vi "Hardware-DI-B-Host.vi"() -> ()   [LabVIEW 2016]
uses:
  <vilib>/Powertrain Controls/Device Drivers/DCM/Rev0/UI/Bank B.ctl
  Shared/Typedefs/DI-Phase-Array-2D.ctl
  <vilib>/Powertrain Controls/Device Drivers/DCM/DI/RT/Phase.ctl
  <vilib>/Powertrain Controls/Device Drivers/DCM/Rev0/FPGA/DI - Drive State.ctl
  <vilib>/Powertrain Controls/Device Drivers/DCM/DI/FPGA/Phase Step.ctl
  <vilib>/Powertrain Controls/Device Drivers/DCM/DI/FPGA/Control.ctl
  <vilib>/Powertrain Controls/Device Drivers/DCM/Rev0/RT/Configuration.ctl
  <vilib>/Powertrain Controls/Device Drivers/DCM/Rev0/FPGA/DI - Bank Configuration.ctl
  Host SubVIs/DI Command Element.ctl
  <vilib>/Powertrain Controls/Device Drivers/DCM/Rev0/FPGA/Digital Channel.ctl
  Shared/Typedefs/DI-Command-Array.ctl
  <vilib>/Powertrain Controls/Device Drivers/DCM/DI/RT/Command.ctl
  <vilib>/Powertrain Controls/Device Drivers/DCM/DI/FPGA/Mode.ctl
  <vilib>/Powertrain Controls/Device Drivers/DCM/DI/RT/Command Sequence.ctl
  <vilib>/Powertrain Controls/Device Drivers/DCM/DI/RT/Angle Control.ctl
  Shared/Typedefs/DI-Phase-Array-1D.ctl
  <vilib>/addons/Software Calibration Management/XControls/SubHost.xctl
  <vilib>/Powertrain Controls/Device Drivers/DCM/Rev0/FPGA/DI - Faults.ctl
  Host SubVIs/Pump Command Element.ctl
  <vilib>/Powertrain Controls/Device Drivers/DCM/Rev0/FPGA/DI - ADC Signals.ctl
  <vilib>/Powertrain Controls/Device Drivers/DCM/DI/FPGA/Capture Event.ctl
  <vilib>/Powertrain Controls/Device Drivers/DCM/Rev0/RT/System State.ctl
  <vilib>/Powertrain Controls/Device Drivers/DCM/Rev0/RT/System ADC.ctl
  <vilib>/Powertrain Controls/Device Drivers/DCM/Rev0/RT/Internal Fault.ctl
  <vilib>/Powertrain Controls/Device Drivers/DCM/Rev0/RT/Run State.ctl
  <vilib>/Powertrain Controls/Device Drivers/DCM/Rev0/UI/Configuration.ctl
  <vilib>/Powertrain Controls/Device Drivers/DCM/Rev0/UI/System Configuration.ctl
  <vilib>/Powertrain Controls/Device Drivers/DCM/Rev0/UI/Injector Configuration.ctl
  <vilib>/Powertrain Controls/Device Drivers/DCM/Rev0/UI/Test Comparators.vi
  <vilib>/Powertrain Controls/Device Drivers/DCM/Rev0/UI/DAC Delay.vi
  <vilib>/Powertrain Controls/Device Drivers/DCM/DI/RT/Phase Convert.vi
  <vilib>/Powertrain Controls/Device Drivers/DCM/DI/RT/Skew.vi
  <vilib>/Powertrain Controls/Device Drivers/DCM/Rev0/UI/Calibrations.vi
  <vilib>/Powertrain Controls/Device Drivers/DCM/Rev0/UI/One Injection Command.vi
  <vilib>/Powertrain Controls/Device Drivers/DCM/DI/FPGA/Simulate Phase Array.vi
  <vilib>/Powertrain Controls/Device Drivers/DCM/Rev0/FPGA/DI - Setpoints.vi
  <vilib>/Powertrain Controls/Device Drivers/DCM/Rev0/UI/Phase State Control.vi
  <vilib>/Powertrain Controls/Device Drivers/DCM/Rev0/UI/Circuit Model Step.vi
  <vilib>/Powertrain Controls/Device Drivers/DCM/Rev0/UI/FET Movie Data.vi
  <vilib>/Powertrain Controls/Device Drivers/DCM/DI/FPGA/DCM - FPGA - DI.lvlib
  <vilib>/Powertrain Controls/Device Drivers/DCM/Rev0/UI/DCM - UI.lvlib
  <vilib>/Powertrain Controls/Device Drivers/DCM/Rev0/FPGA/DCM - FPGA.lvlib
  <vilib>/Powertrain Controls/Device Drivers/DCM/DI/RT/DCM - RT - DI.lvlib
  <vilib>/Powertrain Controls/Device Drivers/DCM/Rev0/RT/DCM - RT.lvclass
  Shared/DSI-Shared.lvlib
panel:
  out "RunState":T1
  out "_BoostSlider":cluster{dbl, dbl, dbl, dbl}(slide)={0.0, 166.94117647058823, 117.76470588235294, 190.23529411764707} scale=0.0..220.0
  out "_Bank B Status":T2 caption="Injector and Pump Simulation Settings" {"Boost Clamp [V]" format="%#_3p"; "Ext HV [V]" format="%#_3p"; "DRVP [V]" format="%#_3p"; "Pump Zener [V]" format="%#_3p"; "DI Zener [V]" format="%#_3p"; "Secondary 3-4 [V]" format="%#_3p"; "Secondary 1-2 [V]" format="%#_3p"; "Primary 3-4 [V]" format="%#_3p"; "Primary 1-2 [V]" format="%#_3p"}
  in  "_DI Bank_Configuration":T3 caption="DI Bank A_Configuration" {"Pump Zener Voltage [V]" min=0 max=240 format="%#_13g"; "DI Zener Voltage [V]" min=0 max=100 format="%#_13g"; "Boost Clamp [V]" min=0 max=220 format="%#_13g"; "Boost Voltage [V]" min=0 max=220 format="%#_13g"}
  in  "DI Scope":T5(xcontrol)
  in  "UserOS":bool
  in  "UserOSTime":sgl caption="[s]" format="%#.3p"
  in  "_Hidden Items":enum32{"DI-A Configurations Items"}(tab)
  out "dt":sgl=13.7
  out "_Bank A?":bool
  in  "_Redraw Slider":bool
  out "SYS|Exec|CalLoading":bool
  in  "_Refresh All":bool
  in  "_Redraw Pump Command":bool
  in  "_Redraw DI Command":bool
  in  "InjCmd":T6=[{"Mode"=enum."Off", "Digital Input"=enum."Unused", "Default Profile Index"=0, "Cal Freq [Hz]"=0.0, "Cal Duration [s]"=0.0, "Cal Increment [s]"=0.0, "Cal Pulses"=0, "TMP Command Sequence"=[{"Duration [s]"=0.0, "Level"=FALSE, "Run/Stop"=FALSE, "Profile Index"=0}, {"Duration [s]"=0.0, "Level"=FALSE, "Run/Stop"=FALSE, "Profile Index"=0}, {"Duration [s]"=0.0, "Level"=FALSE, "Run/Stop"=FALSE, "Profile Index"=0}, {"Duration [s]"=0.0, "Level"=FALSE, "Run/Stop"=FALSE, "Profile Index"=0}, {"Duration [s]"=0.0, "Level"=FALSE, "Run/Stop"=FALSE, "Profile Index"=0}, {"Duration [s]"=0.0, "Level"=FALSE, "Run/Stop"=FALSE, "Profile Index"=0}, {"Duration [s]"=0.0, "Level"=FALSE, "Run/Stop"=FALSE, "Profile Index"=0}, {"Duration [s]"=0.0, "Level"=FALSE, "Run/Stop"=FALSE, "Profile Index"=0}], "EPT TDC Offset [CAD]"=0.0, "EPT Window Start [DBTDC]"=0.0, "EPT Window End [DBTDC]"=0.0, "EPT Angles"=[{"Enable"=FALSE, "Timing [DBTDC]"=0.0, "Duration [s]"=0.0, "Profile Index"=0}, {"Enable"=FALSE, "Timing [DBTDC]"=0.0, "Duration [s]"=0.0, "Profile Index"=0}, {"Enable"=FALSE, "Timing [DBTDC]"=0.0, "Duration [s]"=0.0, "Profile Index"=0}, {"Enable"=FALSE, "Timing [DBTDC]"=0.0, "Duration [s]"=0.0, "Profile Index"=0}], "EPT Skip Fire"=FALSE, "EPT Skip Index"=0, "EPT Precharge Duration [s]"=0.0, "EPT Precharge Profile Index"=0}, {"Mode"=enum."Off", "Digital Input"=enum."Unused", "Default Profile Index"=0, "Cal Freq [Hz]"=0.0, "Cal Duration [s]"=0.0, "Cal Increment [s]"=0.0, "Cal Pulses"=0, "TMP Command Sequence"=[{"Duration [s]"=0.0, "Level"=FALSE, "Run/Stop"=FALSE, "Profile Index"=0}, {"Duration [s]"=0.0, "Level"=FALSE, "Run/Stop"=FALSE, "Profile Index"=0}, {"Duration [s]"=0.0, "Level"=FALSE, "Run/Stop"=FALSE, "Profile Index"=0}, {"Duration [s]"=0.0, "Level"=FALSE, "Run/Stop"=FALSE, "Profile Index"=0}, {"Duration [s]"=0.0, "Level"=FALSE, "Run/Stop"=FALSE, "Profile Index"=0}, {"Duration [s]"=0.0, "Level"=FALSE, "Run/Stop"=FALSE, "Profile Index"=0}, {"Duration [s]"=0.0, "Level"=FALSE, "Run/Stop"=FALSE, "Profile Index"=0}, {"Duration [s]"=0.0, "Level"=FALSE, "Run/Stop"=FALSE, "Profile Index"=0}], "EPT TDC Offset [CAD]"=0.0, "EPT Window Start [DBTDC]"=0.0, "EPT Window End [DBTDC]"=0.0, "EPT Angles"=[{"Enable"=FALSE, "Timing [DBTDC]"=0.0, "Duration [s]"=0.0, "Profile Index"=0}, {"Enable"=FALSE, "Timing [DBTDC]"=0.0, "Duration [s]"=0.0, "Profile Index"=0}, {"Enable"=FALSE, "Timing [DBTDC]"=0.0, "Duration [s]"=0.0, "Profile Index"=0}, {"Enable"=FALSE, "Timing [DBTDC]"=0.0, "Duration [s]"=0.0, "Profile Index"=0}], "EPT Skip Fire"=FALSE, "EPT Skip Index"=0, "EPT Precharge Duration [s]"=0.0, "EPT Precharge Profile Index"=0}, {"Mode"=enum."Off", "Digital Input"=enum."Unused", "Default Profile Index"=0, "Cal Freq [Hz]"=0.0, "Cal Duration [s]"=0.0, "Cal Increment [s]"=0.0, "Cal Pulses"=0, "TMP Command Sequence"=[{"Duration [s]"=0.0, "Level"=FALSE, "Run/Stop"=FALSE, "Profile Index"=0}, {"Duration [s]"=0.0, "Level"=FALSE, "Run/Stop"=FALSE, "Profile Index"=0}, {"Duration [s]"=0.0, "Level"=FALSE, "Run/Stop"=FALSE, "Profile Index"=0}, {"Duration [s]"=0.0, "Level"=FALSE, "Run/Stop"=FALSE, "Profile Index"=0}, {"Duration [s]"=0.0, "Level"=FALSE, "Run/Stop"=FALSE, "Profile Index"=0}, {"Duration [s]"=0.0, "Level"=FALSE, "Run/Stop"=FALSE, "Profile Index"=0}, {"Duration [s]"=0.0, "Level"=FALSE, "Run/Stop"=FALSE, "Profile Index"=0}, {"Duration [s]"=0.0, "Level"=FALSE, "Run/Stop"=FALSE, "Profile Index"=0}], "EPT TDC Offset [CAD]"=0.0, "EPT Window Start [DBTDC]"=0.0, "EPT Window End [DBTDC]"=0.0, "EPT Angles"=[{"Enable"=FALSE, "Timing [DBTDC]"=0.0, "Duration [s]"=0.0, "Profile Index"=0}, {"Enable"=FALSE, "Timing [DBTDC]"=0.0, "Duration [s]"=0.0, "Profile Index"=0}, {"Enable"=FALSE, "Timing [DBTDC]"=0.0, "Duration [s]"=0.0, "Profile Index"=0}, {"Enable"=FALSE, "Timing [DBTDC]"=0.0, "Duration [s]"=0.0, "Profile Index"=0}], "EPT Skip Fire"=FALSE, "EPT Skip Index"=0, "EPT Precharge Duration [s]"=0.0, "EPT Precharge Profile Index"=0}, {"Mode"=enum."Off", "Digital Input"=enum."Unused", "Default Profile Index"=0, "Cal Freq [Hz]"=0.0, "Cal Duration [s]"=0.0, "Cal Increment [s]"=0.0, "Cal Pulses"=0, "TMP Command Sequence"=[{"Duration [s]"=0.0, "Level"=FALSE, "Run/Stop"=FALSE, "Profile Index"=0}, {"Duration [s]"=0.0, "Level"=FALSE, "Run/Stop"=FALSE, "Profile Index"=0}, {"Duration [s]"=0.0, "Level"=FALSE, "Run/Stop"=FALSE, "Profile Index"=0}, {"Duration [s]"=0.0, "Level"=FALSE, "Run/Stop"=FALSE, "Profile Index"=0}, {"Duration [s]"=0.0, "Level"=FALSE, "Run/Stop"=FALSE, "Profile Index"=0}, {"Duration [s]"=0.0, "Level"=FALSE, "Run/Stop"=FALSE, "Profile Index"=0}, {"Duration [s]"=0.0, "Level"=FALSE, "Run/Stop"=FALSE, "Profile Index"=0}, {"Duration [s]"=0.0, "Level"=FALSE, "Run/Stop"=FALSE, "Profile Index"=0}], "EPT TDC Offset [CAD]"=0.0, "EPT Window Start [DBTDC]"=0.0, "EPT Window End [DBTDC]"=0.0, "EPT Angles"=[{"Enable"=FALSE, "Timing [DBTDC]"=0.0, "Duration [s]"=0.0, "Profile Index"=0}, {"Enable"=FALSE, "Timing [DBTDC]"=0.0, "Duration [s]"=0.0, "Profile Index"=0}, {"Enable"=FALSE, "Timing [DBTDC]"=0.0, "Duration [s]"=0.0, "Profile Index"=0}, {"Enable"=FALSE, "Timing [DBTDC]"=0.0, "Duration [s]"=0.0, "Profile Index"=0}], "EPT Skip Fire"=FALSE, "EPT Skip Index"=0, "EPT Precharge Duration [s]"=0.0, "EPT Precharge Profile Index"=0}, {"Mode"=enum."Off", "Digital Input"=enum."Unused", "Default Profile Index"=0, "Cal Freq [Hz]"=0.0, "Cal Duration [s]"=0.0, "Cal Increment [s]"=0.0, "Cal Pulses"=0, "TMP Command Sequence"=[{"Duration [s]"=0.0, "Level"=FALSE, "Run/Stop"=FALSE, "Profile Index"=0}, {"Duration [s]"=0.0, "Level"=FALSE, "Run/Stop"=FALSE, "Profile Index"=0}, {"Duration [s]"=0.0, "Level"=FALSE, "Run/Stop"=FALSE, "Profile Index"=0}, {"Duration [s]"=0.0, "Level"=FALSE, "Run/Stop"=FALSE, "Profile Index"=0}, {"Duration [s]"=0.0, "Level"=FALSE, "Run/Stop"=FALSE, "Profile Index"=0}, {"Duration [s]"=0.0, "Level"=FALSE, "Run/Stop"=FALSE, "Profile Index"=0}, {"Duration [s]"=0.0, "Level"=FALSE, "Run/Stop"=FALSE, "Profile Index"=0}, {"Duration [s]"=0.0, "Level"=FALSE, "Run/Stop"=FALSE, "Profile Index"=0}], "EPT TDC Offset [CAD]"=0.0, "EPT Window Start [DBTDC]"=0.0, "EPT Window End [DBTDC]"=0.0, "EPT Angles"=[{"Enable"=FALSE, "Timing [DBTDC]"=0.0, "Duration [s]"=0.0, "Profile Index"=0}, {"Enable"=FALSE, "Timing [DBTDC]"=0.0, "Duration [s]"=0.0, "Profile Index"=0}, {"Enable"=FALSE, "Timing [DBTDC]"=0.0, "Duration [s]"=0.0, "Profile Index"=0}, {"Enable"=FALSE, "Timing [DBTDC]"=0.0, "Duration [s]"=0.0, "Profile Index"=0}], "EPT Skip Fire"=FALSE, "EPT Skip Index"=0, "EPT Precharge Duration [s]"=0.0, "EPT Precharge Profile Index"=0}, {"Mode"=enum."Off", "Digital Input"=enum."Unused", "Default Profile Index"=0, "Cal Freq [Hz]"=0.0, "Cal Duration [s]"=0.0, "Cal Increment [s]"=0.0, "Cal Pulses"=0, "TMP Command Sequence"=[{"Duration [s]"=0.0, "Level"=FALSE, "Run/Stop"=FALSE, "Profile Index"=0}, {"Duration [s]"=0.0, "Level"=FALSE, "Run/Stop"=FALSE, "Profile Index"=0}, {"Duration [s]"=0.0, "Level"=FALSE, "Run/Stop"=FALSE, "Profile Index"=0}, {"Duration [s]"=0.0, "Level"=FALSE, "Run/Stop"=FALSE, "Profile Index"=0}, {"Duration [s]"=0.0, "Level"=FALSE, "Run/Stop"=FALSE, "Profile Index"=0}, {"Duration [s]"=0.0, "Level"=FALSE, "Run/Stop"=FALSE, "Profile Index"=0}, {"Duration [s]"=0.0, "Level"=FALSE, "Run/Stop"=FALSE, "Profile Index"=0}, {"Duration [s]"=0.0, "Level"=FALSE, "Run/Stop"=FALSE, "Profile Index"=0}], "EPT TDC Offset [CAD]"=0.0, "EPT Window Start [DBTDC]"=0.0, "EPT Window End [DBTDC]"=0.0, "EPT Angles"=[{"Enable"=FALSE, "Timing [DBTDC]"=0.0, "Duration [s]"=0.0, "Profile Index"=0}, {"Enable"=FALSE, "Timing [DBTDC]"=0.0, "Duration [s]"=0.0, "Profile Index"=0}, {"Enable"=FALSE, "Timing [DBTDC]"=0.0, "Duration [s]"=0.0, "Profile Index"=0}, {"Enable"=FALSE, "Timing [DBTDC]"=0.0, "Duration [s]"=0.0, "Profile Index"=0}], "EPT Skip Fire"=FALSE, "EPT Skip Index"=0, "EPT Precharge Duration [s]"=0.0, "EPT Precharge Profile Index"=0}, {"Mode"=enum."Off", "Digital Input"=enum."Unused", "Default Profile Index"=0, "Cal Freq [Hz]"=0.0, "Cal Duration [s]"=0.0, "Cal Increment [s]"=0.0, "Cal Pulses"=0, "TMP Command Sequence"=[{"Duration [s]"=0.0, "Level"=FALSE, "Run/Stop"=FALSE, "Profile Index"=0}, {"Duration [s]"=0.0, "Level"=FALSE, "Run/Stop"=FALSE, "Profile Index"=0}, {"Duration [s]"=0.0, "Level"=FALSE, "Run/Stop"=FALSE, "Profile Index"=0}, {"Duration [s]"=0.0, "Level"=FALSE, "Run/Stop"=FALSE, "Profile Index"=0}, {"Duration [s]"=0.0, "Level"=FALSE, "Run/Stop"=FALSE, "Profile Index"=0}, {"Duration [s]"=0.0, "Level"=FALSE, "Run/Stop"=FALSE, "Profile Index"=0}, {"Duration [s]"=0.0, "Level"=FALSE, "Run/Stop"=FALSE, "Profile Index"=0}, {"Duration [s]"=0.0, "Level"=FALSE, "Run/Stop"=FALSE, "Profile Index"=0}], "EPT TDC Offset [CAD]"=0.0, "EPT Window Start [DBTDC]"=0.0, "EPT Window End [DBTDC]"=0.0, "EPT Angles"=[{"Enable"=FALSE, "Timing [DBTDC]"=0.0, "Duration [s]"=0.0, "Profile Index"=0}, {"Enable"=FALSE, "Timing [DBTDC]"=0.0, "Duration [s]"=0.0, "Profile Index"=0}, {"Enable"=FALSE, "Timing [DBTDC]"=0.0, "Duration [s]"=0.0, "Profile Index"=0}, {"Enable"=FALSE, "Timing [DBTDC]"=0.0, "Duration [s]"=0.0, "Profile Index"=0}], "EPT Skip Fire"=FALSE, "EPT Skip Index"=0, "EPT Precharge Duration [s]"=0.0, "EPT Precharge Profile Index"=0}, {"Mode"=enum."Off", "Digital Input"=enum."Unused", "Default Profile Index"=0, "Cal Freq [Hz]"=0.0, "Cal Duration [s]"=0.0, "Cal Increment [s]"=0.0, "Cal Pulses"=0, "TMP Command Sequence"=[{"Duration [s]"=0.0, "Level"=FALSE, "Run/Stop"=FALSE, "Profile Index"=0}, {"Duration [s]"=0.0, "Level"=FALSE, "Run/Stop"=FALSE, "Profile Index"=0}, {"Duration [s]"=0.0, "Level"=FALSE, "Run/Stop"=FALSE, "Profile Index"=0}, {"Duration [s]"=0.0, "Level"=FALSE, "Run/Stop"=FALSE, "Profile Index"=0}, {"Duration [s]"=0.0, "Level"=FALSE, "Run/Stop"=FALSE, "Profile Index"=0}, {"Duration [s]"=0.0, "Level"=FALSE, "Run/Stop"=FALSE, "Profile Index"=0}, {"Duration [s]"=0.0, "Level"=FALSE, "Run/Stop"=FALSE, "Profile Index"=0}, {"Duration [s]"=0.0, "Level"=FALSE, "Run/Stop"=FALSE, "Profile Index"=0}], "EPT TDC Offset [CAD]"=0.0, "EPT Window Start [DBTDC]"=0.0, "EPT Window End [DBTDC]"=0.0, "EPT Angles"=[{"Enable"=FALSE, "Timing [DBTDC]"=0.0, "Duration [s]"=0.0, "Profile Index"=0}, {"Enable"=FALSE, "Timing [DBTDC]"=0.0, "Duration [s]"=0.0, "Profile Index"=0}, {"Enable"=FALSE, "Timing [DBTDC]"=0.0, "Duration [s]"=0.0, "Profile Index"=0}, {"Enable"=FALSE, "Timing [DBTDC]"=0.0, "Duration [s]"=0.0, "Profile Index"=0}], "EPT Skip Fire"=FALSE, "EPT Skip Index"=0, "EPT Precharge Duration [s]"=0.0, "EPT Precharge Profile Index"=0}] {"EPT Precharge Profile Index" max=15; "EPT Precharge Duration [s]" min=0 format="%#_4p"; "Default Profile Index" max=15; "Cal Increment [s]" format="%#_3p"; "TMP Command Sequence"."Profile Index" max=7; "TMP Command Sequence"."Duration [s]" min=0 max=100 format="%#_3p"; "Cal Pulses" max=511; "EPT Skip Index" max=7; "EPT Angles"."Profile Index" max=7; "EPT Angles"."Duration [s]" min=0 max=100 format="%#_3p"; "Cal Duration [s]" format="%#_3p"; "Cal Freq [Hz]" format="%#_3p"}
  in  "ChanSelect4":u8(ring) items=["I LS A1/A5", "I LS A2/A6", "I LS A3/A7", "I LS A4", "I LS A8/PumpA", "V PZ A1", "V PZ A2", "V PZ A3", "V PZ A4", "V S A1", "V S A2", "V S A3", "V S A4", "V S A5", "V S A6", "V S A7", "V S A8", "V Pump A", "V Secondary A1A2", "V Secondary A3A4", "V Ext HV A", "------------------------ ", "I LS B1/B5", "I LS B2/B6", "I LS B3/B7", "I LS B4", "I LS B8/PumpB", "V PZ B1", "V PZ B2", "V PZ B3", "V PZ B4", "V S B1", "V S B2", "V S B3", "V S B4", "V S B5", "V S B6", "V S B7", "V S B8", "V Pump B", "V Secondary B1B2", "V Secondary B3B4", "V Ext HV B", "-------------------------  ", "AI 1", "AI 2", "AI 3", "AI 4", "AI 5", "AI 6", "AI 7", "AI 8", "AI 9", "AI 10", "AI 11", "AI 12", "-------------------------   ", "V DRVP"]
  in  "ChanSelect3":u8(ring) items=["I LS A1/A5", "I LS A2/A6", "I LS A3/A7", "I LS A4", "I LS A8/PumpA", "V PZ A1", "V PZ A2", "V PZ A3", "V PZ A4", "V S A1", "V S A2", "V S A3", "V S A4", "V S A5", "V S A6", "V S A7", "V S A8", "V Pump A", "V Secondary A1A2", "V Secondary A3A4", "V Ext HV A", "------------------------ ", "I LS B1/B5", "I LS B2/B6", "I LS B3/B7", "I LS B4", "I LS B8/PumpB", "V PZ B1", "V PZ B2", "V PZ B3", "V PZ B4", "V S B1", "V S B2", "V S B3", "V S B4", "V S B5", "V S B6", "V S B7", "V S B8", "V Pump B", "V Secondary B1B2", "V Secondary B3B4", "V Ext HV B", "-------------------------  ", "AI 1", "AI 2", "AI 3", "AI 4", "AI 5", "AI 6", "AI 7", "AI 8", "AI 9", "AI 10", "AI 11", "AI 12", "-------------------------   ", "V DRVP"]
  in  "_Redraw Profiles Usage Tracker":bool
  in  "_Redraw Pump Timing Plot":bool
  in  "InjectEnable":bool
  in  "PSEnable":bool
  in  "Configuration":u8
  in  "BoostV":sgl format="%#_13g"
  in  "ZenerV":sgl format="%#_13g"
  in  "ZenerEnable":bool
  in  "PumpZenerV":sgl format="%#_13g"
  in  "BoostClampV":sgl format="%#_13g"
  in  "_Redraw Phase":bool
  in  "_Redraw Phase Plot":bool
  in  "_Redraw Phase Lists":bool
  in  "_Redraw Pump Phase Plot":bool
  in  "_Redraw Pump Phase List":bool
  in  "FaultClear":u8
  in  "ChanSelect2":u8(ring) items=["I LS A1/A5", "I LS A2/A6", "I LS A3/A7", "I LS A4", "I LS A8/PumpA", "V PZ A1", "V PZ A2", "V PZ A3", "V PZ A4", "V S A1", "V S A2", "V S A3", "V S A4", "V S A5", "V S A6", "V S A7", "V S A8", "V Pump A", "V Secondary A1A2", "V Secondary A3A4", "V Ext HV A", "------------------------ ", "I LS B1/B5", "I LS B2/B6", "I LS B3/B7", "I LS B4", "I LS B8/PumpB", "V PZ B1", "V PZ B2", "V PZ B3", "V PZ B4", "V S B1", "V S B2", "V S B3", "V S B4", "V S B5", "V S B6", "V S B7", "V S B8", "V Pump B", "V Secondary B1B2", "V Secondary B3B4", "V Ext HV B", "-------------------------  ", "AI 1", "AI 2", "AI 3", "AI 4", "AI 5", "AI 6", "AI 7", "AI 8", "AI 9", "AI 10", "AI 11", "AI 12", "-------------------------   ", "V DRVP"]
  in  "ChanSelect1":u8(ring) items=["I LS A1/A5", "I LS A2/A6", "I LS A3/A7", "I LS A4", "I LS A8/PumpA", "V PZ A1", "V PZ A2", "V PZ A3", "V PZ A4", "V S A1", "V S A2", "V S A3", "V S A4", "V S A5", "V S A6", "V S A7", "V S A8", "V Pump A", "V Secondary A1A2", "V Secondary A3A4", "V Ext HV A", "------------------------ ", "I LS B1/B5", "I LS B2/B6", "I LS B3/B7", "I LS B4", "I LS B8/PumpB", "V PZ B1", "V PZ B2", "V PZ B3", "V PZ B4", "V S B1", "V S B2", "V S B3", "V S B4", "V S B5", "V S B6", "V S B7", "V S B8", "V Pump B", "V Secondary B1B2", "V Secondary B3B4", "V Ext HV B", "-------------------------  ", "AI 1", "AI 2", "AI 3", "AI 4", "AI 5", "AI 6", "AI 7", "AI 8", "AI 9", "AI 10", "AI 11", "AI 12", "-------------------------   ", "V DRVP"]
  in  "ScopeEnable":bool
  in  "ScopeEvent":u8(ring) items=["Unused", "Injector A1", "Injector A2", "Injector A3", "Injector A4", "Injector A5", "Injector A6", "Injector A7", "Injector A8/PumpA", "Injector B1", "Injector B2", "Injector B3", "Injector B4", "Injector B5", "Injector B6", "Injector B7", "Injector B8/PumpB", "Diff IO 1", "Diff IO 2", "Diff IO 3", "Diff IO 4", "Diff IO 5", "Diff IO 6", "Diff IO 7", "Diff IO 8", "Aux 1", "Aux 2", "Aux 3", "Aux 4", "Aux 5", "Aux 6", "Aux 7", "Aux 8", "User OS"]
  out "Data":sgl[][](array[numeric])
  out "_Ref Pump Profiles":cluster{"Array":dbl[], "Array":dbl[]}[](array[cluster])
  out "_Ref Inj Profiles":cluster{"Array":dbl[], "Array":dbl[]}[](array[cluster])
  out "_SimuXY":cluster{"Array":dbl[], "Array":dbl[]}[](array[cluster])
  in  "PumpPhase":T12=[{"Drive"=enum."Idle", "Direction"=FALSE, "Phase Step"=enum."Duration", "Duration [s]"=0.0, "Current High [A]"=0.0, "Current Low [A]"=0.0, "Voltage High [V]"=0.0, "Voltage Low [V]"=0.0, "Change"=FALSE, "Current Control"=enum."Closed Loop", "Period [s]"=0.0, "Pulse Width [s]"=0.0, "Profile"=0, "Voltage Control"=FALSE}, {"Drive"=enum."Idle", "Direction"=FALSE, "Phase Step"=enum."Duration", "Duration [s]"=0.0, "Current High [A]"=0.0, "Current Low [A]"=0.0, "Voltage High [V]"=0.0, "Voltage Low [V]"=0.0, "Change"=FALSE, "Current Control"=enum."Closed Loop", "Period [s]"=0.0, "Pulse Width [s]"=0.0, "Profile"=0, "Voltage Control"=FALSE}, {"Drive"=enum."Idle", "Direction"=FALSE, "Phase Step"=enum."Duration", "Duration [s]"=0.0, "Current High [A]"=0.0, "Current Low [A]"=0.0, "Voltage High [V]"=0.0, "Voltage Low [V]"=0.0, "Change"=FALSE, "Current Control"=enum."Closed Loop", "Period [s]"=0.0, "Pulse Width [s]"=0.0, "Profile"=0, "Voltage Control"=FALSE}, {"Drive"=enum."Idle", "Direction"=FALSE, "Phase Step"=enum."Duration", "Duration [s]"=0.0, "Current High [A]"=0.0, "Current Low [A]"=0.0, "Voltage High [V]"=0.0, "Voltage Low [V]"=0.0, "Change"=FALSE, "Current Control"=enum."Closed Loop", "Period [s]"=0.0, "Pulse Width [s]"=0.0, "Profile"=0, "Voltage Control"=FALSE}, {"Drive"=enum."Idle", "Direction"=FALSE, "Phase Step"=enum."Duration", "Duration [s]"=0.0, "Current High [A]"=0.0, "Current Low [A]"=0.0, "Voltage High [V]"=0.0, "Voltage Low [V]"=0.0, "Change"=FALSE, "Current Control"=enum."Closed Loop", "Period [s]"=0.0, "Pulse Width [s]"=0.0, "Profile"=0, "Voltage Control"=FALSE}, {"Drive"=enum."Idle", "Direction"=FALSE, "Phase Step"=enum."Duration", "Duration [s]"=0.0, "Current High [A]"=0.0, "Current Low [A]"=0.0, "Voltage High [V]"=0.0, "Voltage Low [V]"=0.0, "Change"=FALSE, "Current Control"=enum."Closed Loop", "Period [s]"=0.0, "Pulse Width [s]"=0.0, "Profile"=0, "Voltage Control"=FALSE}, {"Drive"=enum."Idle", "Direction"=FALSE, "Phase Step"=enum."Duration", "Duration [s]"=0.0, "Current High [A]"=0.0, "Current Low [A]"=0.0, "Voltage High [V]"=0.0, "Voltage Low [V]"=0.0, "Change"=FALSE, "Current Control"=enum."Closed Loop", "Period [s]"=0.0, "Pulse Width [s]"=0.0, "Profile"=0, "Voltage Control"=FALSE}, {"Drive"=enum."Idle", "Direction"=FALSE, "Phase Step"=enum."Duration", "Duration [s]"=0.0, "Current High [A]"=0.0, "Current Low [A]"=0.0, "Voltage High [V]"=0.0, "Voltage Low [V]"=0.0, "Change"=FALSE, "Current Control"=enum."Closed Loop", "Period [s]"=0.0, "Pulse Width [s]"=0.0, "Profile"=0, "Voltage Control"=FALSE}, {"Drive"=enum."Idle", "Direction"=FALSE, "Phase Step"=enum."Duration", "Duration [s]"=0.0, "Current High [A]"=0.0, "Current Low [A]"=0.0, "Voltage High [V]"=0.0, "Voltage Low [V]"=0.0, "Change"=FALSE, "Current Control"=enum."Closed Loop", "Period [s]"=0.0, "Pulse Width [s]"=0.0, "Profile"=0, "Voltage Control"=FALSE}, {"Drive"=enum."Idle", "Direction"=FALSE, "Phase Step"=enum."Duration", "Duration [s]"=0.0, "Current High [A]"=0.0, "Current Low [A]"=0.0, "Voltage High [V]"=0.0, "Voltage Low [V]"=0.0, "Change"=FALSE, "Current Control"=enum."Closed Loop", "Period [s]"=0.0, "Pulse Width [s]"=0.0, "Profile"=0, "Voltage Control"=FALSE}, {"Drive"=enum."Idle", "Direction"=FALSE, "Phase Step"=enum."Duration", "Duration [s]"=0.0, "Current High [A]"=0.0, "Current Low [A]"=0.0, "Voltage High [V]"=0.0, "Voltage Low [V]"=0.0, "Change"=FALSE, "Current Control"=enum."Closed Loop", "Period [s]"=0.0, "Pulse Width [s]"=0.0, "Profile"=0, "Voltage Control"=FALSE}, {"Drive"=enum."Idle", "Direction"=FALSE, "Phase Step"=enum."Duration", "Duration [s]"=0.0, "Current High [A]"=0.0, "Current Low [A]"=0.0, "Voltage High [V]"=0.0, "Voltage Low [V]"=0.0, "Change"=FALSE, "Current Control"=enum."Closed Loop", "Period [s]"=0.0, "Pulse Width [s]"=0.0, "Profile"=0, "Voltage Control"=FALSE}, {"Drive"=enum."Idle", "Direction"=FALSE, "Phase Step"=enum."Duration", "Duration [s]"=0.0, "Current High [A]"=0.0, "Current Low [A]"=0.0, "Voltage High [V]"=0.0, "Voltage Low [V]"=0.0, "Change"=FALSE, "Current Control"=enum."Closed Loop", "Period [s]"=0.0, "Pulse Width [s]"=0.0, "Profile"=0, "Voltage Control"=FALSE}, {"Drive"=enum."Idle", "Direction"=FALSE, "Phase Step"=enum."Duration", "Duration [s]"=0.0, "Current High [A]"=0.0, "Current Low [A]"=0.0, "Voltage High [V]"=0.0, "Voltage Low [V]"=0.0, "Change"=FALSE, "Current Control"=enum."Closed Loop", "Period [s]"=0.0, "Pulse Width [s]"=0.0, "Profile"=0, "Voltage Control"=FALSE}, {"Drive"=enum."Idle", "Direction"=FALSE, "Phase Step"=enum."Duration", "Duration [s]"=0.0, "Current High [A]"=0.0, "Current Low [A]"=0.0, "Voltage High [V]"=0.0, "Voltage Low [V]"=0.0, "Change"=FALSE, "Current Control"=enum."Closed Loop", "Period [s]"=0.0, "Pulse Width [s]"=0.0, "Profile"=0, "Voltage Control"=FALSE}, {"Drive"=enum."Idle", "Direction"=FALSE, "Phase Step"=enum."Duration", "Duration [s]"=0.0, "Current High [A]"=0.0, "Current Low [A]"=0.0, "Voltage High [V]"=0.0, "Voltage Low [V]"=0.0, "Change"=FALSE, "Current Control"=enum."Closed Loop", "Period [s]"=0.0, "Pulse Width [s]"=0.0, "Profile"=0, "Voltage Control"=FALSE}] caption="Pump A Phase Arrays" {"Profile" max=15; "Period [s]" min=4e-06 max=0.000102 format="%#_3p"; "Pulse Width [s]" min=0 max=0.000102 format="%#_3p"; "Voltage Low [V]" min=-220 max=220 format="%#_3p"; "Voltage High [V]" min=-220 max=220 format="%#_3p"; "Current Low [A]" min=-40 max=40 format="%#_3p"; "Current High [A]" min=-40 max=40 format="%#_3p"; "Duration [s]" min=0 max=1.67772 format="%#_3p"}
  in  "_Redraw Timing Plot":bool
  in  "_Redraw Injection List":bool
  in  "InjAdaptMode":u32
  in  "InjPhasePlotColors":sgl[](array[numeric])
  in  "RefInjTimeAxisMultiplier":sgl
  in  "RefInjTimeAxisOffset":sgl
  in  "RefInjCurrentMultiplier":sgl
  in  "RefInjCurrentOffset":sgl
  in  "RefInjVoltageMultiplier":sgl
  in  "RefInjVoltageOffset":sgl
  in  "RefPumpTimeAxisMultiplier":sgl
  in  "RefPumpTimeAxisOffset":sgl
  in  "RefPumpCurrentMultiplier":sgl
  in  "RefPumpCurrentOffset":sgl
  in  "RefPumpVoltageMultiplier":sgl
  in  "RefPumpVoltageOffset":sgl
  in  "InjPhasePlotLineWidths":sgl[](array[numeric])
  in  "InjPhasePlotLineTypes":sgl[](array[numeric])
  in  "InjCmdPlotColors":sgl[](array[numeric])
  in  "InjCmdPlotLineWidths":sgl[](array[numeric])
  in  "InjCmdPlotLineTypes":sgl[](array[numeric])
  in  "PumpPhasePlotColors":sgl[](array[numeric])
  in  "PumpPhasePlotLineWidths":sgl[](array[numeric])
  in  "PumpPhasePlotLineTypes":sgl[](array[numeric])
  in  "PumpCmdPlotColors":sgl[](array[numeric])
  in  "PumpCmdPlotLineWidths":sgl[](array[numeric])
  in  "PumpCmdPlotLineTypes":sgl[](array[numeric])
  in  "PumpCapacitance":sgl=5e-06 format="%#_6p"
  in  "PumpInductance":sgl=0.0001 format="%#_6p"
  in  "PumpResistance":sgl=1.0 format="%#_6p"
  in  "SimSpeed":sgl=5e-06 format="%#_6p"
  in  "SimRotations":u8
  in  "InjCapacitance":sgl=5e-06 format="%#_6p"
  in  "InjInductance":sgl=0.0001 format="%#_6p"
  in  "InjResistance":sgl=1.0 format="%#_6p"
  in  "SimBatt":sgl=13.7 min=6 max=32
  in  "_Redraw Pump Phase":bool
  in  "InjPhase":T17=[[{"Drive"=enum."Idle", "Direction"=FALSE, "Phase Step"=enum."Duration", "Duration [s]"=0.0, "Current High [A]"=0.0, "Current Low [A]"=0.0, "Voltage High [V]"=0.0, "Voltage Low [V]"=0.0, "Change"=FALSE, "Current Control"=enum."Closed Loop", "Period [s]"=0.0, "Pulse Width [s]"=0.0, "Profile"=0, "Voltage Control"=FALSE}, {"Drive"=enum."Idle", "Direction"=FALSE, "Phase Step"=enum."Duration", "Duration [s]"=0.0, "Current High [A]"=0.0, "Current Low [A]"=0.0, "Voltage High [V]"=0.0, "Voltage Low [V]"=0.0, "Change"=FALSE, "Current Control"=enum."Closed Loop", "Period [s]"=0.0, "Pulse Width [s]"=0.0, "Profile"=0, "Voltage Control"=FALSE}, {"Drive"=enum."Idle", "Direction"=FALSE, "Phase Step"=enum."Duration", "Duration [s]"=0.0, "Current High [A]"=0.0, "Current Low [A]"=0.0, "Voltage High [V]"=0.0, "Voltage Low [V]"=0.0, "Change"=FALSE, "Current Control"=enum."Closed Loop", "Period [s]"=0.0, "Pulse Width [s]"=0.0, "Profile"=0, "Voltage Control"=FALSE}, {"Drive"=enum."Idle", "Direction"=FALSE, "Phase Step"=enum."Duration", "Duration [s]"=0.0, "Current High [A]"=0.0, "Current Low [A]"=0.0, "Voltage High [V]"=0.0, "Voltage Low [V]"=0.0, "Change"=FALSE, "Current Control"=enum."Closed Loop", "Period [s]"=0.0, "Pulse Width [s]"=0.0, "Profile"=0, "Voltage Control"=FALSE}, {"Drive"=enum."Idle", "Direction"=FALSE, "Phase Step"=enum."Duration", "Duration [s]"=0.0, "Current High [A]"=0.0, "Current Low [A]"=0.0, "Voltage High [V]"=0.0, "Voltage Low [V]"=0.0, "Change"=FALSE, "Current Control"=enum."Closed Loop", "Period [s]"=0.0, "Pulse Width [s]"=0.0, "Profile"=0, "Voltage Control"=FALSE}, {"Drive"=enum."Idle", "Direction"=FALSE, "Phase Step"=enum."Duration", "Duration [s]"=0.0, "Current High [A]"=0.0, "Current Low [A]"=0.0, "Voltage High [V]"=0.0, "Voltage Low [V]"=0.0, "Change"=FALSE, "Current Control"=enum."Closed Loop", "Period [s]"=0.0, "Pulse Width [s]"=0.0, "Profile"=0, "Voltage Control"=FALSE}, {"Drive"=enum."Idle", "Direction"=FALSE, "Phase Step"=enum."Duration", "Duration [s]"=0.0, "Current High [A]"=0.0, "Current Low [A]"=0.0, "Voltage High [V]"=0.0, "Voltage Low [V]"=0.0, "Change"=FALSE, "Current Control"=enum."Closed Loop", "Period [s]"=0.0, "Pulse Width [s]"=0.0, "Profile"=0, "Voltage Control"=FALSE}, {"Drive"=enum."Idle", "Direction"=FALSE, "Phase Step"=enum."Duration", "Duration [s]"=0.0, "Current High [A]"=0.0, "Current Low [A]"=0.0, "Voltage High [V]"=0.0, "Voltage Low [V]"=0.0, "Change"=FALSE, "Current Control"=enum."Closed Loop", "Period [s]"=0.0, "Pulse Width [s]"=0.0, "Profile"=0, "Voltage Control"=FALSE}, {"Drive"=enum."Idle", "Direction"=FALSE, "Phase Step"=enum."Duration", "Duration [s]"=0.0, "Current High [A]"=0.0, "Current Low [A]"=0.0, "Voltage High [V]"=0.0, "Voltage Low [V]"=0.0, "Change"=FALSE, "Current Control"=enum."Closed Loop", "Period [s]"=0.0, "Pulse Width [s]"=0.0, "Profile"=0, "Voltage Control"=FALSE}, {"Drive"=enum."Idle", "Direction"=FALSE, "Phase Step"=enum."Duration", "Duration [s]"=0.0, "Current High [A]"=0.0, "Current Low [A]"=0.0, "Voltage High [V]"=0.0, "Voltage Low [V]"=0.0, "Change"=FALSE, "Current Control"=enum."Closed Loop", "Period [s]"=0.0, "Pulse Width [s]"=0.0, "Profile"=0, "Voltage Control"=FALSE}, {"Drive"=enum."Idle", "Direction"=FALSE, "Phase Step"=enum."Duration", "Duration [s]"=0.0, "Current High [A]"=0.0, "Current Low [A]"=0.0, "Voltage High [V]"=0.0, "Voltage Low [V]"=0.0, "Change"=FALSE, "Current Control"=enum."Closed Loop", "Period [s]"=0.0, "Pulse Width [s]"=0.0, "Profile"=0, "Voltage Control"=FALSE}, {"Drive"=enum."Idle", "Direction"=FALSE, "Phase Step"=enum."Duration", "Duration [s]"=0.0, "Current High [A]"=0.0, "Current Low [A]"=0.0, "Voltage High [V]"=0.0, "Voltage Low [V]"=0.0, "Change"=FALSE, "Current Control"=enum."Closed Loop", "Period [s]"=0.0, "Pulse Width [s]"=0.0, "Profile"=0, "Voltage Control"=FALSE}, {"Drive"=enum."Idle", "Direction"=FALSE, "Phase Step"=enum."Duration", "Duration [s]"=0.0, "Current High [A]"=0.0, "Current Low [A]"=0.0, "Voltage High [V]"=0.0, "Voltage Low [V]"=0.0, "Change"=FALSE, "Current Control"=enum."Closed Loop", "Period [s]"=0.0, "Pulse Width [s]"=0.0, "Profile"=0, "Voltage Control"=FALSE}, {"Drive"=enum."Idle", "Direction"=FALSE, "Phase Step"=enum."Duration", "Duration [s]"=0.0, "Current High [A]"=0.0, "Current Low [A]"=0.0, "Voltage High [V]"=0.0, "Voltage Low [V]"=0.0, "Change"=FALSE, "Current Control"=enum."Closed Loop", "Period [s]"=0.0, "Pulse Width [s]"=0.0, "Profile"=0, "Voltage Control"=FALSE}, {"Drive"=enum."Idle", "Direction"=FALSE, "Phase Step"=enum."Duration", "Duration [s]"=0.0, "Current High [A]"=0.0, "Current Low [A]"=0.0, "Voltage High [V]"=0.0, "Voltage Low [V]"=0.0, "Change"=FALSE, "Current Control"=enum."Closed Loop", "Period [s]"=0.0, "Pulse Width [s]"=0.0, "Profile"=0, "Voltage Control"=FALSE}, {"Drive"=enum."Idle", "Direction"=FALSE, "Phase Step"=enum."Duration", "Duration [s]"=0.0, "Current High [A]"=0.0, "Current Low [A]"=0.0, "Voltage High [V]"=0.0, "Voltage Low [V]"=0.0, "Change"=FALSE, "Current Control"=enum."Closed Loop", "Period [s]"=0.0, "Pulse Width [s]"=0.0, "Profile"=0, "Voltage Control"=FALSE}], [{"Drive"=enum."Idle", "Direction"=FALSE, "Phase Step"=enum."Duration", "Duration [s]"=0.0, "Current High [A]"=0.0, "Current Low [A]"=0.0, "Voltage High [V]"=0.0, "Voltage Low [V]"=0.0, "Change"=FALSE, "Current Control"=enum."Closed Loop", "Period [s]"=0.0, "Pulse Width [s]"=0.0, "Profile"=0, "Voltage Control"=FALSE}, {"Drive"=enum."Idle", "Direction"=FALSE, "Phase Step"=enum."Duration", "Duration [s]"=0.0, "Current High [A]"=0.0, "Current Low [A]"=0.0, "Voltage High [V]"=0.0, "Voltage Low [V]"=0.0, "Change"=FALSE, "Current Control"=enum."Closed Loop", "Period [s]"=0.0, "Pulse Width [s]"=0.0, "Profile"=0, "Voltage Control"=FALSE}, {"Drive"=enum."Idle", "Direction"=FALSE, "Phase Step"=enum."Duration", "Duration [s]"=0.0, "Current High [A]"=0.0, "Current Low [A]"=0.0, "Voltage High [V]"=0.0, "Voltage Low [V]"=0.0, "Change"=FALSE, "Current Control"=enum."Closed Loop", "Period [s]"=0.0, "Pulse Width [s]"=0.0, "Profile"=0, "Voltage Control"=FALSE}, {"Drive"=enum."Idle", "Direction"=FALSE, "Phase Step"=enum."Duration", "Duration [s]"=0.0, "Current High [A]"=0.0, "Current Low [A]"=0.0, "Voltage High [V]"=0.0, "Voltage Low [V]"=0.0, "Change"=FALSE, "Current Control"=enum."Closed Loop", "Period [s]"=0.0, "Pulse Width [s]"=0.0, "Profile"=0, "Voltage Control"=FALSE}, {"Drive"=enum."Idle", "Direction"=FALSE, "Phase Step"=enum."Duration", "Duration [s]"=0.0, "Current High [A]"=0.0, "Current Low [A]"=0.0, "Voltage High [V]"=0.0, "Voltage Low [V]"=0.0, "Change"=FALSE, "Current Control"=enum."Closed Loop", "Period [s]"=0.0, "Pulse Width [s]"=0.0, "Profile"=0, "Voltage Control"=FALSE}, {"Drive"=enum."Idle", "Direction"=FALSE, "Phase Step"=enum."Duration", "Duration [s]"=0.0, "Current High [A]"=0.0, "Current Low [A]"=0.0, "Voltage High [V]"=0.0, "Voltage Low [V]"=0.0, "Change"=FALSE, "Current Control"=enum."Closed Loop", "Period [s]"=0.0, "Pulse Width [s]"=0.0, "Profile"=0, "Voltage Control"=FALSE}, {"Drive"=enum."Idle", "Direction"=FALSE, "Phase Step"=enum."Duration", "Duration [s]"=0.0, "Current High [A]"=0.0, "Current Low [A]"=0.0, "Voltage High [V]"=0.0, "Voltage Low [V]"=0.0, "Change"=FALSE, "Current Control"=enum."Closed Loop", "Period [s]"=0.0, "Pulse Width [s]"=0.0, "Profile"=0, "Voltage Control"=FALSE}, {"Drive"=enum."Idle", "Direction"=FALSE, "Phase Step"=enum."Duration", "Duration [s]"=0.0, "Current High [A]"=0.0, "Current Low [A]"=0.0, "Voltage High [V]"=0.0, "Voltage Low [V]"=0.0, "Change"=FALSE, "Current Control"=enum."Closed Loop", "Period [s]"=0.0, "Pulse Width [s]"=0.0, "Profile"=0, "Voltage Control"=FALSE}, {"Drive"=enum."Idle", "Direction"=FALSE, "Phase Step"=enum."Duration", "Duration [s]"=0.0, "Current High [A]"=0.0, "Current Low [A]"=0.0, "Voltage High [V]"=0.0, "Voltage Low [V]"=0.0, "Change"=FALSE, "Current Control"=enum."Closed Loop", "Period [s]"=0.0, "Pulse Width [s]"=0.0, "Profile"=0, "Voltage Control"=FALSE}, {"Drive"=enum."Idle", "Direction"=FALSE, "Phase Step"=enum."Duration", "Duration [s]"=0.0, "Current High [A]"=0.0, "Current Low [A]"=0.0, "Voltage High [V]"=0.0, "Voltage Low [V]"=0.0, "Change"=FALSE, "Current Control"=enum."Closed Loop", "Period [s]"=0.0, "Pulse Width [s]"=0.0, "Profile"=0, "Voltage Control"=FALSE}, {"Drive"=enum."Idle", "Direction"=FALSE, "Phase Step"=enum."Duration", "Duration [s]"=0.0, "Current High [A]"=0.0, "Current Low [A]"=0.0, "Voltage High [V]"=0.0, "Voltage Low [V]"=0.0, "Change"=FALSE, "Current Control"=enum."Closed Loop", "Period [s]"=0.0, "Pulse Width [s]"=0.0, "Profile"=0, "Voltage Control"=FALSE}, {"Drive"=enum."Idle", "Direction"=FALSE, "Phase Step"=enum."Duration", "Duration [s]"=0.0, "Current High [A]"=0.0, "Current Low [A]"=0.0, "Voltage High [V]"=0.0, "Voltage Low [V]"=0.0, "Change"=FALSE, "Current Control"=enum."Closed Loop", "Period [s]"=0.0, "Pulse Width [s]"=0.0, "Profile"=0, "Voltage Control"=FALSE}, {"Drive"=enum."Idle", "Direction"=FALSE, "Phase Step"=enum."Duration", "Duration [s]"=0.0, "Current High [A]"=0.0, "Current Low [A]"=0.0, "Voltage High [V]"=0.0, "Voltage Low [V]"=0.0, "Change"=FALSE, "Current Control"=enum."Closed Loop", "Period [s]"=0.0, "Pulse Width [s]"=0.0, "Profile"=0, "Voltage Control"=FALSE}, {"Drive"=enum."Idle", "Direction"=FALSE, "Phase Step"=enum."Duration", "Duration [s]"=0.0, "Current High [A]"=0.0, "Current Low [A]"=0.0, "Voltage High [V]"=0.0, "Voltage Low [V]"=0.0, "Change"=FALSE, "Current Control"=enum."Closed Loop", "Period [s]"=0.0, "Pulse Width [s]"=0.0, "Profile"=0, "Voltage Control"=FALSE}, {"Drive"=enum."Idle", "Direction"=FALSE, "Phase Step"=enum."Duration", "Duration [s]"=0.0, "Current High [A]"=0.0, "Current Low [A]"=0.0, "Voltage High [V]"=0.0, "Voltage Low [V]"=0.0, "Change"=FALSE, "Current Control"=enum."Closed Loop", "Period [s]"=0.0, "Pulse Width [s]"=0.0, "Profile"=0, "Voltage Control"=FALSE}, {"Drive"=enum."Idle", "Direction"=FALSE, "Phase Step"=enum."Duration", "Duration [s]"=0.0, "Current High [A]"=0.0, "Current Low [A]"=0.0, "Voltage High [V]"=0.0, "Voltage Low [V]"=0.0, "Change"=FALSE, "Current Control"=enum."Closed Loop", "Period [s]"=0.0, "Pulse Width [s]"=0.0, "Profile"=0, "Voltage Control"=FALSE}], [{"Drive"=enum."Idle", "Direction"=FALSE, "Phase Step"=enum."Duration", "Duration [s]"=0.0, "Current High [A]"=0.0, "Current Low [A]"=0.0, "Voltage High [V]"=0.0, "Voltage Low [V]"=0.0, "Change"=FALSE, "Current Control"=enum."Closed Loop", "Period [s]"=0.0, "Pulse Width [s]"=0.0, "Profile"=0, "Voltage Control"=FALSE}, {"Drive"=enum."Idle", "Direction"=FALSE, "Phase Step"=enum."Duration", "Duration [s]"=0.0, "Current High [A]"=0.0, "Current Low [A]"=0.0, "Voltage High [V]"=0.0, "Voltage Low [V]"=0.0, "Change"=FALSE, "Current Control"=enum."Closed Loop", "Period [s]"=0.0, "Pulse Width [s]"=0.0, "Profile"=0, "Voltage Control"=FALSE}, {"Drive"=enum."Idle", "Direction"=FALSE, "Phase Step"=enum."Duration", "Duration [s]"=0.0, "Current High [A]"=0.0, "Current Low [A]"=0.0, "Voltage High [V]"=0.0, "Voltage Low [V]"=0.0, "Change"=FALSE, "Current Control"=enum."Closed Loop", "Period [s]"=0.0, "Pulse Width [s]"=0.0, "Profile"=0, "Voltage Control"=FALSE}, {"Drive"=enum."Idle", "Direction"=FALSE, "Phase Step"=enum."Duration", "Duration [s]"=0.0, "Current High [A]"=0.0, "Current Low [A]"=0.0, "Voltage High [V]"=0.0, "Voltage Low [V]"=0.0, "Change"=FALSE, "Current Control"=enum."Closed Loop", "Period [s]"=0.0, "Pulse Width [s]"=0.0, "Profile"=0, "Voltage Control"=FALSE}, {"Drive"=enum."Idle", "Direction"=FALSE, "Phase Step"=enum."Duration", "Duration [s]"=0.0, "Current High [A]"=0.0, "Current Low [A]"=0.0, "Voltage High [V]"=0.0, "Voltage Low [V]"=0.0, "Change"=FALSE, "Current Control"=enum."Closed Loop", "Period [s]"=0.0, "Pulse Width [s]"=0.0, "Profile"=0, "Voltage Control"=FALSE}, {"Drive"=enum."Idle", "Direction"=FALSE, "Phase Step"=enum."Duration", "Duration [s]"=0.0, "Current High [A]"=0.0, "Current Low [A]"=0.0, "Voltage High [V]"=0.0, "Voltage Low [V]"=0.0, "Change"=FALSE, "Current Control"=enum."Closed Loop", "Period [s]"=0.0, "Pulse Width [s]"=0.0, "Profile"=0, "Voltage Control"=FALSE}, {"Drive"=enum."Idle", "Direction"=FALSE, "Phase Step"=enum."Duration", "Duration [s]"=0.0, "Current High [A]"=0.0, "Current Low [A]"=0.0, "Voltage High [V]"=0.0, "Voltage Low [V]"=0.0, "Change"=FALSE, "Current Control"=enum."Closed Loop", "Period [s]"=0.0, "Pulse Width [s]"=0.0, "Profile"=0, "Voltage Control"=FALSE}, {"Drive"=enum."Idle", "Direction"=FALSE, "Phase Step"=enum."Duration", "Duration [s]"=0.0, "Current High [A]"=0.0, "Current Low [A]"=0.0, "Voltage High [V]"=0.0, "Voltage Low [V]"=0.0, "Change"=FALSE, "Current Control"=enum."Closed Loop", "Period [s]"=0.0, "Pulse Width [s]"=0.0, "Profile"=0, "Voltage Control"=FALSE}, {"Drive"=enum."Idle", "Direction"=FALSE, "Phase Step"=enum."Duration", "Duration [s]"=0.0, "Current High [A]"=0.0, "Current Low [A]"=0.0, "Voltage High [V]"=0.0, "Voltage Low [V]"=0.0, "Change"=FALSE, "Current Control"=enum."Closed Loop", "Period [s]"=0.0, "Pulse Width [s]"=0.0, "Profile"=0, "Voltage Control"=FALSE}, {"Drive"=enum."Idle", "Direction"=FALSE, "Phase Step"=enum."Duration", "Duration [s]"=0.0, "Current High [A]"=0.0, "Current Low [A]"=0.0, "Voltage High [V]"=0.0, "Voltage Low [V]"=0.0, "Change"=FALSE, "Current Control"=enum."Closed Loop", "Period [s]"=0.0, "Pulse Width [s]"=0.0, "Profile"=0, "Voltage Control"=FALSE}, {"Drive"=enum."Idle", "Direction"=FALSE, "Phase Step"=enum."Duration", "Duration [s]"=0.0, "Current High [A]"=0.0, "Current Low [A]"=0.0, "Voltage High [V]"=0.0, "Voltage Low [V]"=0.0, "Change"=FALSE, "Current Control"=enum."Closed Loop", "Period [s]"=0.0, "Pulse Width [s]"=0.0, "Profile"=0, "Voltage Control"=FALSE}, {"Drive"=enum."Idle", "Direction"=FALSE, "Phase Step"=enum."Duration", "Duration [s]"=0.0, "Current High [A]"=0.0, "Current Low [A]"=0.0, "Voltage High [V]"=0.0, "Voltage Low [V]"=0.0, "Change"=FALSE, "Current Control"=enum."Closed Loop", "Period [s]"=0.0, "Pulse Width [s]"=0.0, "Profile"=0, "Voltage Control"=FALSE}, {"Drive"=enum."Idle", "Direction"=FALSE, "Phase Step"=enum."Duration", "Duration [s]"=0.0, "Current High [A]"=0.0, "Current Low [A]"=0.0, "Voltage High [V]"=0.0, "Voltage Low [V]"=0.0, "Change"=FALSE, "Current Control"=enum."Closed Loop", "Period [s]"=0.0, "Pulse Width [s]"=0.0, "Profile"=0, "Voltage Control"=FALSE}, {"Drive"=enum."Idle", "Direction"=FALSE, "Phase Step"=enum."Duration", "Duration [s]"=0.0, "Current High [A]"=0.0, "Current Low [A]"=0.0, "Voltage High [V]"=0.0, "Voltage Low [V]"=0.0, "Change"=FALSE, "Current Control"=enum."Closed Loop", "Period [s]"=0.0, "Pulse Width [s]"=0.0, "Profile"=0, "Voltage Control"=FALSE}, {"Drive"=enum."Idle", "Direction"=FALSE, "Phase Step"=enum."Duration", "Duration [s]"=0.0, "Current High [A]"=0.0, "Current Low [A]"=0.0, "Voltage High [V]"=0.0, "Voltage Low [V]"=0.0, "Change"=FALSE, "Current Control"=enum."Closed Loop", "Period [s]"=0.0, "Pulse Width [s]"=0.0, "Profile"=0, "Voltage Control"=FALSE}, {"Drive"=enum."Idle", "Direction"=FALSE, "Phase Step"=enum."Duration", "Duration [s]"=0.0, "Current High [A]"=0.0, "Current Low [A]"=0.0, "Voltage High [V]"=0.0, "Voltage Low [V]"=0.0, "Change"=FALSE, "Current Control"=enum."Closed Loop", "Period [s]"=0.0, "Pulse Width [s]"=0.0, "Profile"=0, "Voltage Control"=FALSE}], [{"Drive"=enum."Idle", "Direction"=FALSE, "Phase Step"=enum."Duration", "Duration [s]"=0.0, "Current High [A]"=0.0, "Current Low [A]"=0.0, "Voltage High [V]"=0.0, "Voltage Low [V]"=0.0, "Change"=FALSE, "Current Control"=enum."Closed Loop", "Period [s]"=0.0, "Pulse Width [s]"=0.0, "Profile"=0, "Voltage Control"=FALSE}, {"Drive"=enum."Idle", "Direction"=FALSE, "Phase Step"=enum."Duration", "Duration [s]"=0.0, "Current High [A]"=0.0, "Current Low [A]"=0.0, "Voltage High [V]"=0.0, "Voltage Low [V]"=0.0, "Change"=FALSE, "Current Control"=enum."Closed Loop", "Period [s]"=0.0, "Pulse Width [s]"=0.0, "Profile"=0, "Voltage Control"=FALSE}, {"Drive"=enum."Idle", "Direction"=FALSE, "Phase Step"=enum."Duration", "Duration [s]"=0.0, "Current High [A]"=0.0, "Current Low [A]"=0.0, "Voltage High [V]"=0.0, "Voltage Low [V]"=0.0, "Change"=FALSE, "Current Control"=enum."Closed Loop", "Period [s]"=0.0, "Pulse Width [s]"=0.0, "Profile"=0, "Voltage Control"=FALSE}, {"Drive"=enum."Idle", "Direction"=FALSE, "Phase Step"=enum."Duration", "Duration [s]"=0.0, "Current High [A]"=0.0, "Current Low [A]"=0.0, "Voltage High [V]"=0.0, "Voltage Low [V]"=0.0, "Change"=FALSE, "Current Control"=enum."Closed Loop", "Period [s]"=0.0, "Pulse Width [s]"=0.0, "Profile"=0, "Voltage Control"=FALSE}, {"Drive"=enum."Idle", "Direction"=FALSE, "Phase Step"=enum."Duration", "Duration [s]"=0.0, "Current High [A]"=0.0, "Current Low [A]"=0.0, "Voltage High [V]"=0.0, "Voltage Low [V]"=0.0, "Change"=FALSE, "Current Control"=enum."Closed Loop", "Period [s]"=0.0, "Pulse Width [s]"=0.0, "Profile"=0, "Voltage Control"=FALSE}, {"Drive"=enum."Idle", "Direction"=FALSE, "Phase Step"=enum."Duration", "Duration [s]"=0.0, "Current High [A]"=0.0, "Current Low [A]"=0.0, "Voltage High [V]"=0.0, "Voltage Low [V]"=0.0, "Change"=FALSE, "Current Control"=enum."Closed Loop", "Period [s]"=0.0, "Pulse Width [s]"=0.0, "Profile"=0, "Voltage Control"=FALSE}, {"Drive"=enum."Idle", "Direction"=FALSE, "Phase Step"=enum."Duration", "Duration [s]"=0.0, "Current High [A]"=0.0, "Current Low [A]"=0.0, "Voltage High [V]"=0.0, "Voltage Low [V]"=0.0, "Change"=FALSE, "Current Control"=enum."Closed Loop", "Period [s]"=0.0, "Pulse Width [s]"=0.0, "Profile"=0, "Voltage Control"=FALSE}, {"Drive"=enum."Idle", "Direction"=FALSE, "Phase Step"=enum."Duration", "Duration [s]"=0.0, "Current High [A]"=0.0, "Current Low [A]"=0.0, "Voltage High [V]"=0.0, "Voltage Low [V]"=0.0, "Change"=FALSE, "Current Control"=enum."Closed Loop", "Period [s]"=0.0, "Pulse Width [s]"=0.0, "Profile"=0, "Voltage Control"=FALSE}, {"Drive"=enum."Idle", "Direction"=FALSE, "Phase Step"=enum."Duration", "Duration [s]"=0.0, "Current High [A]"=0.0, "Current Low [A]"=0.0, "Voltage High [V]"=0.0, "Voltage Low [V]"=0.0, "Change"=FALSE, "Current Control"=enum."Closed Loop", "Period [s]"=0.0, "Pulse Width [s]"=0.0, "Profile"=0, "Voltage Control"=FALSE}, {"Drive"=enum."Idle", "Direction"=FALSE, "Phase Step"=enum."Duration", "Duration [s]"=0.0, "Current High [A]"=0.0, "Current Low [A]"=0.0, "Voltage High [V]"=0.0, "Voltage Low [V]"=0.0, "Change"=FALSE, "Current Control"=enum."Closed Loop", "Period [s]"=0.0, "Pulse Width [s]"=0.0, "Profile"=0, "Voltage Control"=FALSE}, {"Drive"=enum."Idle", "Direction"=FALSE, "Phase Step"=enum."Duration", "Duration [s]"=0.0, "Current High [A]"=0.0, "Current Low [A]"=0.0, "Voltage High [V]"=0.0, "Voltage Low [V]"=0.0, "Change"=FALSE, "Current Control"=enum."Closed Loop", "Period [s]"=0.0, "Pulse Width [s]"=0.0, "Profile"=0, "Voltage Control"=FALSE}, {"Drive"=enum."Idle", "Direction"=FALSE, "Phase Step"=enum."Duration", "Duration [s]"=0.0, "Current High [A]"=0.0, "Current Low [A]"=0.0, "Voltage High [V]"=0.0, "Voltage Low [V]"=0.0, "Change"=FALSE, "Current Control"=enum."Closed Loop", "Period [s]"=0.0, "Pulse Width [s]"=0.0, "Profile"=0, "Voltage Control"=FALSE}, {"Drive"=enum."Idle", "Direction"=FALSE, "Phase Step"=enum."Duration", "Duration [s]"=0.0, "Current High [A]"=0.0, "Current Low [A]"=0.0, "Voltage High [V]"=0.0, "Voltage Low [V]"=0.0, "Change"=FALSE, "Current Control"=enum."Closed Loop", "Period [s]"=0.0, "Pulse Width [s]"=0.0, "Profile"=0, "Voltage Control"=FALSE}, {"Drive"=enum."Idle", "Direction"=FALSE, "Phase Step"=enum."Duration", "Duration [s]"=0.0, "Current High [A]"=0.0, "Current Low [A]"=0.0, "Voltage High [V]"=0.0, "Voltage Low [V]"=0.0, "Change"=FALSE, "Current Control"=enum."Closed Loop", "Period [s]"=0.0, "Pulse Width [s]"=0.0, "Profile"=0, "Voltage Control"=FALSE}, {"Drive"=enum."Idle", "Direction"=FALSE, "Phase Step"=enum."Duration", "Duration [s]"=0.0, "Current High [A]"=0.0, "Current Low [A]"=0.0, "Voltage High [V]"=0.0, "Voltage Low [V]"=0.0, "Change"=FALSE, "Current Control"=enum."Closed Loop", "Period [s]"=0.0, "Pulse Width [s]"=0.0, "Profile"=0, "Voltage Control"=FALSE}, {"Drive"=enum."Idle", "Direction"=FALSE, "Phase Step"=enum."Duration", "Duration [s]"=0.0, "Current High [A]"=0.0, "Current Low [A]"=0.0, "Voltage High [V]"=0.0, "Voltage Low [V]"=0.0, "Change"=FALSE, "Current Control"=enum."Closed Loop", "Period [s]"=0.0, "Pulse Width [s]"=0.0, "Profile"=0, "Voltage Control"=FALSE}], [{"Drive"=enum."Idle", "Direction"=FALSE, "Phase Step"=enum."Duration", "Duration [s]"=0.0, "Current High [A]"=0.0, "Current Low [A]"=0.0, "Voltage High [V]"=0.0, "Voltage Low [V]"=0.0, "Change"=FALSE, "Current Control"=enum."Closed Loop", "Period [s]"=0.0, "Pulse Width [s]"=0.0, "Profile"=0, "Voltage Control"=FALSE}, {"Drive"=enum."Idle", "Direction"=FALSE, "Phase Step"=enum."Duration", "Duration [s]"=0.0, "Current High [A]"=0.0, "Current Low [A]"=0.0, "Voltage High [V]"=0.0, "Voltage Low [V]"=0.0, "Change"=FALSE, "Current Control"=enum."Closed Loop", "Period [s]"=0.0, "Pulse Width [s]"=0.0, "Profile"=0, "Voltage Control"=FALSE}, {"Drive"=enum."Idle", "Direction"=FALSE, "Phase Step"=enum."Duration", "Duration [s]"=0.0, "Current High [A]"=0.0, "Current Low [A]"=0.0, "Voltage High [V]"=0.0, "Voltage Low [V]"=0.0, "Change"=FALSE, "Current Control"=enum."Closed Loop", "Period [s]"=0.0, "Pulse Width [s]"=0.0, "Profile"=0, "Voltage Control"=FALSE}, {"Drive"=enum."Idle", "Direction"=FALSE, "Phase Step"=enum."Duration", "Duration [s]"=0.0, "Current High [A]"=0.0, "Current Low [A]"=0.0, "Voltage High [V]"=0.0, "Voltage Low [V]"=0.0, "Change"=FALSE, "Current Control"=enum."Closed Loop", "Period [s]"=0.0, "Pulse Width [s]"=0.0, "Profile"=0, "Voltage Control"=FALSE}, {"Drive"=enum."Idle", "Direction"=FALSE, "Phase Step"=enum."Duration", "Duration [s]"=0.0, "Current High [A]"=0.0, "Current Low [A]"=0.0, "Voltage High [V]"=0.0, "Voltage Low [V]"=0.0, "Change"=FALSE, "Current Control"=enum."Closed Loop", "Period [s]"=0.0, "Pulse Width [s]"=0.0, "Profile"=0, "Voltage Control"=FALSE}, {"Drive"=enum."Idle", "Direction"=FALSE, "Phase Step"=enum."Duration", "Duration [s]"=0.0, "Current High [A]"=0.0, "Current Low [A]"=0.0, "Voltage High [V]"=0.0, "Voltage Low [V]"=0.0, "Change"=FALSE, "Current Control"=enum."Closed Loop", "Period [s]"=0.0, "Pulse Width [s]"=0.0, "Profile"=0, "Voltage Control"=FALSE}, {"Drive"=enum."Idle", "Direction"=FALSE, "Phase Step"=enum."Duration", "Duration [s]"=0.0, "Current High [A]"=0.0, "Current Low [A]"=0.0, "Voltage High [V]"=0.0, "Voltage Low [V]"=0.0, "Change"=FALSE, "Current Control"=enum."Closed Loop", "Period [s]"=0.0, "Pulse Width [s]"=0.0, "Profile"=0, "Voltage Control"=FALSE}, {"Drive"=enum."Idle", "Direction"=FALSE, "Phase Step"=enum."Duration", "Duration [s]"=0.0, "Current High [A]"=0.0, "Current Low [A]"=0.0, "Voltage High [V]"=0.0, "Voltage Low [V]"=0.0, "Change"=FALSE, "Current Control"=enum."Closed Loop", "Period [s]"=0.0, "Pulse Width [s]"=0.0, "Profile"=0, "Voltage Control"=FALSE}, {"Drive"=enum."Idle", "Direction"=FALSE, "Phase Step"=enum."Duration", "Duration [s]"=0.0, "Current High [A]"=0.0, "Current Low [A]"=0.0, "Voltage High [V]"=0.0, "Voltage Low [V]"=0.0, "Change"=FALSE, "Current Control"=enum."Closed Loop", "Period [s]"=0.0, "Pulse Width [s]"=0.0, "Profile"=0, "Voltage Control"=FALSE}, {"Drive"=enum."Idle", "Direction"=FALSE, "Phase Step"=enum."Duration", "Duration [s]"=0.0, "Current High [A]"=0.0, "Current Low [A]"=0.0, "Voltage High [V]"=0.0, "Voltage Low [V]"=0.0, "Change"=FALSE, "Current Control"=enum."Closed Loop", "Period [s]"=0.0, "Pulse Width [s]"=0.0, "Profile"=0, "Voltage Control"=FALSE}, {"Drive"=enum."Idle", "Direction"=FALSE, "Phase Step"=enum."Duration", "Duration [s]"=0.0, "Current High [A]"=0.0, "Current Low [A]"=0.0, "Voltage High [V]"=0.0, "Voltage Low [V]"=0.0, "Change"=FALSE, "Current Control"=enum."Closed Loop", "Period [s]"=0.0, "Pulse Width [s]"=0.0, "Profile"=0, "Voltage Control"=FALSE}, {"Drive"=enum."Idle", "Direction"=FALSE, "Phase Step"=enum."Duration", "Duration [s]"=0.0, "Current High [A]"=0.0, "Current Low [A]"=0.0, "Voltage High [V]"=0.0, "Voltage Low [V]"=0.0, "Change"=FALSE, "Current Control"=enum."Closed Loop", "Period [s]"=0.0, "Pulse Width [s]"=0.0, "Profile"=0, "Voltage Control"=FALSE}, {"Drive"=enum."Idle", "Direction"=FALSE, "Phase Step"=enum."Duration", "Duration [s]"=0.0, "Current High [A]"=0.0, "Current Low [A]"=0.0, "Voltage High [V]"=0.0, "Voltage Low [V]"=0.0, "Change"=FALSE, "Current Control"=enum."Closed Loop", "Period [s]"=0.0, "Pulse Width [s]"=0.0, "Profile"=0, "Voltage Control"=FALSE}, {"Drive"=enum."Idle", "Direction"=FALSE, "Phase Step"=enum."Duration", "Duration [s]"=0.0, "Current High [A]"=0.0, "Current Low [A]"=0.0, "Voltage High [V]"=0.0, "Voltage Low [V]"=0.0, "Change"=FALSE, "Current Control"=enum."Closed Loop", "Period [s]"=0.0, "Pulse Width [s]"=0.0, "Profile"=0, "Voltage Control"=FALSE}, {"Drive"=enum."Idle", "Direction"=FALSE, "Phase Step"=enum."Duration", "Duration [s]"=0.0, "Current High [A]"=0.0, "Current Low [A]"=0.0, "Voltage High [V]"=0.0, "Voltage Low [V]"=0.0, "Change"=FALSE, "Current Control"=enum."Closed Loop", "Period [s]"=0.0, "Pulse Width [s]"=0.0, "Profile"=0, "Voltage Control"=FALSE}, {"Drive"=enum."Idle", "Direction"=FALSE, "Phase Step"=enum."Duration", "Duration [s]"=0.0, "Current High [A]"=0.0, "Current Low [A]"=0.0, "Voltage High [V]"=0.0, "Voltage Low [V]"=0.0, "Change"=FALSE, "Current Control"=enum."Closed Loop", "Period [s]"=0.0, "Pulse Width [s]"=0.0, "Profile"=0, "Voltage Control"=FALSE}], [{"Drive"=enum."Idle", "Direction"=FALSE, "Phase Step"=enum."Duration", "Duration [s]"=0.0, "Current High [A]"=0.0, "Current Low [A]"=0.0, "Voltage High [V]"=0.0, "Voltage Low [V]"=0.0, "Change"=FALSE, "Current Control"=enum."Closed Loop", "Period [s]"=0.0, "Pulse Width [s]"=0.0, "Profile"=0, "Voltage Control"=FALSE}, {"Drive"=enum."Idle", "Direction"=FALSE, "Phase Step"=enum."Duration", "Duration [s]"=0.0, "Current High [A]"=0.0, "Current Low [A]"=0.0, "Voltage High [V]"=0.0, "Voltage Low [V]"=0.0, "Change"=FALSE, "Current Control"=enum."Closed Loop", "Period [s]"=0.0, "Pulse Width [s]"=0.0, "Profile"=0, "Voltage Control"=FALSE}, {"Drive"=enum."Idle", "Direction"=FALSE, "Phase Step"=enum."Duration", "Duration [s]"=0.0, "Current High [A]"=0.0, "Current Low [A]"=0.0, "Voltage High [V]"=0.0, "Voltage Low [V]"=0.0, "Change"=FALSE, "Current Control"=enum."Closed Loop", "Period [s]"=0.0, "Pulse Width [s]"=0.0, "Profile"=0, "Voltage Control"=FALSE}, {"Drive"=enum."Idle", "Direction"=FALSE, "Phase Step"=enum."Duration", "Duration [s]"=0.0, "Current High [A]"=0.0, "Current Low [A]"=0.0, "Voltage High [V]"=0.0, "Voltage Low [V]"=0.0, "Change"=FALSE, "Current Control"=enum."Closed Loop", "Period [s]"=0.0, "Pulse Width [s]"=0.0, "Profile"=0, "Voltage Control"=FALSE}, {"Drive"=enum."Idle", "Direction"=FALSE, "Phase Step"=enum."Duration", "Duration [s]"=0.0, "Current High [A]"=0.0, "Current Low [A]"=0.0, "Voltage High [V]"=0.0, "Voltage Low [V]"=0.0, "Change"=FALSE, "Current Control"=enum."Closed Loop", "Period [s]"=0.0, "Pulse Width [s]"=0.0, "Profile"=0, "Voltage Control"=FALSE}, {"Drive"=enum."Idle", "Direction"=FALSE, "Phase Step"=enum."Duration", "Duration [s]"=0.0, "Current High [A]"=0.0, "Current Low [A]"=0.0, "Voltage High [V]"=0.0, "Voltage Low [V]"=0.0, "Change"=FALSE, "Current Control"=enum."Closed Loop", "Period [s]"=0.0, "Pulse Width [s]"=0.0, "Profile"=0, "Voltage Control"=FALSE}, {"Drive"=enum."Idle", "Direction"=FALSE, "Phase Step"=enum."Duration", "Duration [s]"=0.0, "Current High [A]"=0.0, "Current Low [A]"=0.0, "Voltage High [V]"=0.0, "Voltage Low [V]"=0.0, "Change"=FALSE, "Current Control"=enum."Closed Loop", "Period [s]"=0.0, "Pulse Width [s]"=0.0, "Profile"=0, "Voltage Control"=FALSE}, {"Drive"=enum."Idle", "Direction"=FALSE, "Phase Step"=enum."Duration", "Duration [s]"=0.0, "Current High [A]"=0.0, "Current Low [A]"=0.0, "Voltage High [V]"=0.0, "Voltage Low [V]"=0.0, "Change"=FALSE, "Current Control"=enum."Closed Loop", "Period [s]"=0.0, "Pulse Width [s]"=0.0, "Profile"=0, "Voltage Control"=FALSE}, {"Drive"=enum."Idle", "Direction"=FALSE, "Phase Step"=enum."Duration", "Duration [s]"=0.0, "Current High [A]"=0.0, "Current Low [A]"=0.0, "Voltage High [V]"=0.0, "Voltage Low [V]"=0.0, "Change"=FALSE, "Current Control"=enum."Closed Loop", "Period [s]"=0.0, "Pulse Width [s]"=0.0, "Profile"=0, "Voltage Control"=FALSE}, {"Drive"=enum."Idle", "Direction"=FALSE, "Phase Step"=enum."Duration", "Duration [s]"=0.0, "Current High [A]"=0.0, "Current Low [A]"=0.0, "Voltage High [V]"=0.0, "Voltage Low [V]"=0.0, "Change"=FALSE, "Current Control"=enum."Closed Loop", "Period [s]"=0.0, "Pulse Width [s]"=0.0, "Profile"=0, "Voltage Control"=FALSE}, {"Drive"=enum."Idle", "Direction"=FALSE, "Phase Step"=enum."Duration", "Duration [s]"=0.0, "Current High [A]"=0.0, "Current Low [A]"=0.0, "Voltage High [V]"=0.0, "Voltage Low [V]"=0.0, "Change"=FALSE, "Current Control"=enum."Closed Loop", "Period [s]"=0.0, "Pulse Width [s]"=0.0, "Profile"=0, "Voltage Control"=FALSE}, {"Drive"=enum."Idle", "Direction"=FALSE, "Phase Step"=enum."Duration", "Duration [s]"=0.0, "Current High [A]"=0.0, "Current Low [A]"=0.0, "Voltage High [V]"=0.0, "Voltage Low [V]"=0.0, "Change"=FALSE, "Current Control"=enum."Closed Loop", "Period [s]"=0.0, "Pulse Width [s]"=0.0, "Profile"=0, "Voltage Control"=FALSE}, {"Drive"=enum."Idle", "Direction"=FALSE, "Phase Step"=enum."Duration", "Duration [s]"=0.0, "Current High [A]"=0.0, "Current Low [A]"=0.0, "Voltage High [V]"=0.0, "Voltage Low [V]"=0.0, "Change"=FALSE, "Current Control"=enum."Closed Loop", "Period [s]"=0.0, "Pulse Width [s]"=0.0, "Profile"=0, "Voltage Control"=FALSE}, {"Drive"=enum."Idle", "Direction"=FALSE, "Phase Step"=enum."Duration", "Duration [s]"=0.0, "Current High [A]"=0.0, "Current Low [A]"=0.0, "Voltage High [V]"=0.0, "Voltage Low [V]"=0.0, "Change"=FALSE, "Current Control"=enum."Closed Loop", "Period [s]"=0.0, "Pulse Width [s]"=0.0, "Profile"=0, "Voltage Control"=FALSE}, {"Drive"=enum."Idle", "Direction"=FALSE, "Phase Step"=enum."Duration", "Duration [s]"=0.0, "Current High [A]"=0.0, "Current Low [A]"=0.0, "Voltage High [V]"=0.0, "Voltage Low [V]"=0.0, "Change"=FALSE, "Current Control"=enum."Closed Loop", "Period [s]"=0.0, "Pulse Width [s]"=0.0, "Profile"=0, "Voltage Control"=FALSE}, {"Drive"=enum."Idle", "Direction"=FALSE, "Phase Step"=enum."Duration", "Duration [s]"=0.0, "Current High [A]"=0.0, "Current Low [A]"=0.0, "Voltage High [V]"=0.0, "Voltage Low [V]"=0.0, "Change"=FALSE, "Current Control"=enum."Closed Loop", "Period [s]"=0.0, "Pulse Width [s]"=0.0, "Profile"=0, "Voltage Control"=FALSE}], [{"Drive"=enum."Idle", "Direction"=FALSE, "Phase Step"=enum."Duration", "Duration [s]"=0.0, "Current High [A]"=0.0, "Current Low [A]"=0.0, "Voltage High [V]"=0.0, "Voltage Low [V]"=0.0, "Change"=FALSE, "Current Control"=enum."Closed Loop", "Period [s]"=0.0, "Pulse Width [s]"=0.0, "Profile"=0, "Voltage Control"=FALSE}, {"Drive"=enum."Idle", "Direction"=FALSE, "Phase Step"=enum."Duration", "Duration [s]"=0.0, "Current High [A]"=0.0, "Current Low [A]"=0.0, "Voltage High [V]"=0.0, "Voltage Low [V]"=0.0, "Change"=FALSE, "Current Control"=enum."Closed Loop", "Period [s]"=0.0, "Pulse Width [s]"=0.0, "Profile"=0, "Voltage Control"=FALSE}, {"Drive"=enum."Idle", "Direction"=FALSE, "Phase Step"=enum."Duration", "Duration [s]"=0.0, "Current High [A]"=0.0, "Current Low [A]"=0.0, "Voltage High [V]"=0.0, "Voltage Low [V]"=0.0, "Change"=FALSE, "Current Control"=enum."Closed Loop", "Period [s]"=0.0, "Pulse Width [s]"=0.0, "Profile"=0, "Voltage Control"=FALSE}, {"Drive"=enum."Idle", "Direction"=FALSE, "Phase Step"=enum."Duration", "Duration [s]"=0.0, "Current High [A]"=0.0, "Current Low [A]"=0.0, "Voltage High [V]"=0.0, "Voltage Low [V]"=0.0, "Change"=FALSE, "Current Control"=enum."Closed Loop", "Period [s]"=0.0, "Pulse Width [s]"=0.0, "Profile"=0, "Voltage Control"=FALSE}, {"Drive"=enum."Idle", "Direction"=FALSE, "Phase Step"=enum."Duration", "Duration [s]"=0.0, "Current High [A]"=0.0, "Current Low [A]"=0.0, "Voltage High [V]"=0.0, "Voltage Low [V]"=0.0, "Change"=FALSE, "Current Control"=enum."Closed Loop", "Period [s]"=0.0, "Pulse Width [s]"=0.0, "Profile"=0, "Voltage Control"=FALSE}, {"Drive"=enum."Idle", "Direction"=FALSE, "Phase Step"=enum."Duration", "Duration [s]"=0.0, "Current High [A]"=0.0, "Current Low [A]"=0.0, "Voltage High [V]"=0.0, "Voltage Low [V]"=0.0, "Change"=FALSE, "Current Control"=enum."Closed Loop", "Period [s]"=0.0, "Pulse Width [s]"=0.0, "Profile"=0, "Voltage Control"=FALSE}, {"Drive"=enum."Idle", "Direction"=FALSE, "Phase Step"=enum."Duration", "Duration [s]"=0.0, "Current High [A]"=0.0, "Current Low [A]"=0.0, "Voltage High [V]"=0.0, "Voltage Low [V]"=0.0, "Change"=FALSE, "Current Control"=enum."Closed Loop", "Period [s]"=0.0, "Pulse Width [s]"=0.0, "Profile"=0, "Voltage Control"=FALSE}, {"Drive"=enum."Idle", "Direction"=FALSE, "Phase Step"=enum."Duration", "Duration [s]"=0.0, "Current High [A]"=0.0, "Current Low [A]"=0.0, "Voltage High [V]"=0.0, "Voltage Low [V]"=0.0, "Change"=FALSE, "Current Control"=enum."Closed Loop", "Period [s]"=0.0, "Pulse Width [s]"=0.0, "Profile"=0, "Voltage Control"=FALSE}, {"Drive"=enum."Idle", "Direction"=FALSE, "Phase Step"=enum."Duration", "Duration [s]"=0.0, "Current High [A]"=0.0, "Current Low [A]"=0.0, "Voltage High [V]"=0.0, "Voltage Low [V]"=0.0, "Change"=FALSE, "Current Control"=enum."Closed Loop", "Period [s]"=0.0, "Pulse Width [s]"=0.0, "Profile"=0, "Voltage Control"=FALSE}, {"Drive"=enum."Idle", "Direction"=FALSE, "Phase Step"=enum."Duration", "Duration [s]"=0.0, "Current High [A]"=0.0, "Current Low [A]"=0.0, "Voltage High [V]"=0.0, "Voltage Low [V]"=0.0, "Change"=FALSE, "Current Control"=enum."Closed Loop", "Period [s]"=0.0, "Pulse Width [s]"=0.0, "Profile"=0, "Voltage Control"=FALSE}, {"Drive"=enum."Idle", "Direction"=FALSE, "Phase Step"=enum."Duration", "Duration [s]"=0.0, "Current High [A]"=0.0, "Current Low [A]"=0.0, "Voltage High [V]"=0.0, "Voltage Low [V]"=0.0, "Change"=FALSE, "Current Control"=enum."Closed Loop", "Period [s]"=0.0, "Pulse Width [s]"=0.0, "Profile"=0, "Voltage Control"=FALSE}, {"Drive"=enum."Idle", "Direction"=FALSE, "Phase Step"=enum."Duration", "Duration [s]"=0.0, "Current High [A]"=0.0, "Current Low [A]"=0.0, "Voltage High [V]"=0.0, "Voltage Low [V]"=0.0, "Change"=FALSE, "Current Control"=enum."Closed Loop", "Period [s]"=0.0, "Pulse Width [s]"=0.0, "Profile"=0, "Voltage Control"=FALSE}, {"Drive"=enum."Idle", "Direction"=FALSE, "Phase Step"=enum."Duration", "Duration [s]"=0.0, "Current High [A]"=0.0, "Current Low [A]"=0.0, "Voltage High [V]"=0.0, "Voltage Low [V]"=0.0, "Change"=FALSE, "Current Control"=enum."Closed Loop", "Period [s]"=0.0, "Pulse Width [s]"=0.0, "Profile"=0, "Voltage Control"=FALSE}, {"Drive"=enum."Idle", "Direction"=FALSE, "Phase Step"=enum."Duration", "Duration [s]"=0.0, "Current High [A]"=0.0, "Current Low [A]"=0.0, "Voltage High [V]"=0.0, "Voltage Low [V]"=0.0, "Change"=FALSE, "Current Control"=enum."Closed Loop", "Period [s]"=0.0, "Pulse Width [s]"=0.0, "Profile"=0, "Voltage Control"=FALSE}, {"Drive"=enum."Idle", "Direction"=FALSE, "Phase Step"=enum."Duration", "Duration [s]"=0.0, "Current High [A]"=0.0, "Current Low [A]"=0.0, "Voltage High [V]"=0.0, "Voltage Low [V]"=0.0, "Change"=FALSE, "Current Control"=enum."Closed Loop", "Period [s]"=0.0, "Pulse Width [s]"=0.0, "Profile"=0, "Voltage Control"=FALSE}, {"Drive"=enum."Idle", "Direction"=FALSE, "Phase Step"=enum."Duration", "Duration [s]"=0.0, "Current High [A]"=0.0, "Current Low [A]"=0.0, "Voltage High [V]"=0.0, "Voltage Low [V]"=0.0, "Change"=FALSE, "Current Control"=enum."Closed Loop", "Period [s]"=0.0, "Pulse Width [s]"=0.0, "Profile"=0, "Voltage Control"=FALSE}], [{"Drive"=enum."Idle", "Direction"=FALSE, "Phase Step"=enum."Duration", "Duration [s]"=0.0, "Current High [A]"=0.0, "Current Low [A]"=0.0, "Voltage High [V]"=0.0, "Voltage Low [V]"=0.0, "Change"=FALSE, "Current Control"=enum."Closed Loop", "Period [s]"=0.0, "Pulse Width [s]"=0.0, "Profile"=0, "Voltage Control"=FALSE}, {"Drive"=enum."Idle", "Direction"=FALSE, "Phase Step"=enum."Duration", "Duration [s]"=0.0, "Current High [A]"=0.0, "Current Low [A]"=0.0, "Voltage High [V]"=0.0, "Voltage Low [V]"=0.0, "Change"=FALSE, "Current Control"=enum."Closed Loop", "Period [s]"=0.0, "Pulse Width [s]"=0.0, "Profile"=0, "Voltage Control"=FALSE}, {"Drive"=enum."Idle", "Direction"=FALSE, "Phase Step"=enum."Duration", "Duration [s]"=0.0, "Current High [A]"=0.0, "Current Low [A]"=0.0, "Voltage High [V]"=0.0, "Voltage Low [V]"=0.0, "Change"=FALSE, "Current Control"=enum."Closed Loop", "Period [s]"=0.0, "Pulse Width [s]"=0.0, "Profile"=0, "Voltage Control"=FALSE}, {"Drive"=enum."Idle", "Direction"=FALSE, "Phase Step"=enum."Duration", "Duration [s]"=0.0, "Current High [A]"=0.0, "Current Low [A]"=0.0, "Voltage High [V]"=0.0, "Voltage Low [V]"=0.0, "Change"=FALSE, "Current Control"=enum."Closed Loop", "Period [s]"=0.0, "Pulse Width [s]"=0.0, "Profile"=0, "Voltage Control"=FALSE}, {"Drive"=enum."Idle", "Direction"=FALSE, "Phase Step"=enum."Duration", "Duration [s]"=0.0, "Current High [A]"=0.0, "Current Low [A]"=0.0, "Voltage High [V]"=0.0, "Voltage Low [V]"=0.0, "Change"=FALSE, "Current Control"=enum."Closed Loop", "Period [s]"=0.0, "Pulse Width [s]"=0.0, "Profile"=0, "Voltage Control"=FALSE}, {"Drive"=enum."Idle", "Direction"=FALSE, "Phase Step"=enum."Duration", "Duration [s]"=0.0, "Current High [A]"=0.0, "Current Low [A]"=0.0, "Voltage High [V]"=0.0, "Voltage Low [V]"=0.0, "Change"=FALSE, "Current Control"=enum."Closed Loop", "Period [s]"=0.0, "Pulse Width [s]"=0.0, "Profile"=0, "Voltage Control"=FALSE}, {"Drive"=enum."Idle", "Direction"=FALSE, "Phase Step"=enum."Duration", "Duration [s]"=0.0, "Current High [A]"=0.0, "Current Low [A]"=0.0, "Voltage High [V]"=0.0, "Voltage Low [V]"=0.0, "Change"=FALSE, "Current Control"=enum."Closed Loop", "Period [s]"=0.0, "Pulse Width [s]"=0.0, "Profile"=0, "Voltage Control"=FALSE}, {"Drive"=enum."Idle", "Direction"=FALSE, "Phase Step"=enum."Duration", "Duration [s]"=0.0, "Current High [A]"=0.0, "Current Low [A]"=0.0, "Voltage High [V]"=0.0, "Voltage Low [V]"=0.0, "Change"=FALSE, "Current Control"=enum."Closed Loop", "Period [s]"=0.0, "Pulse Width [s]"=0.0, "Profile"=0, "Voltage Control"=FALSE}, {"Drive"=enum."Idle", "Direction"=FALSE, "Phase Step"=enum."Duration", "Duration [s]"=0.0, "Current High [A]"=0.0, "Current Low [A]"=0.0, "Voltage High [V]"=0.0, "Voltage Low [V]"=0.0, "Change"=FALSE, "Current Control"=enum."Closed Loop", "Period [s]"=0.0, "Pulse Width [s]"=0.0, "Profile"=0, "Voltage Control"=FALSE}, {"Drive"=enum."Idle", "Direction"=FALSE, "Phase Step"=enum."Duration", "Duration [s]"=0.0, "Current High [A]"=0.0, "Current Low [A]"=0.0, "Voltage High [V]"=0.0, "Voltage Low [V]"=0.0, "Change"=FALSE, "Current Control"=enum."Closed Loop", "Period [s]"=0.0, "Pulse Width [s]"=0.0, "Profile"=0, "Voltage Control"=FALSE}, {"Drive"=enum."Idle", "Direction"=FALSE, "Phase Step"=enum."Duration", "Duration [s]"=0.0, "Current High [A]"=0.0, "Current Low [A]"=0.0, "Voltage High [V]"=0.0, "Voltage Low [V]"=0.0, "Change"=FALSE, "Current Control"=enum."Closed Loop", "Period [s]"=0.0, "Pulse Width [s]"=0.0, "Profile"=0, "Voltage Control"=FALSE}, {"Drive"=enum."Idle", "Direction"=FALSE, "Phase Step"=enum."Duration", "Duration [s]"=0.0, "Current High [A]"=0.0, "Current Low [A]"=0.0, "Voltage High [V]"=0.0, "Voltage Low [V]"=0.0, "Change"=FALSE, "Current Control"=enum."Closed Loop", "Period [s]"=0.0, "Pulse Width [s]"=0.0, "Profile"=0, "Voltage Control"=FALSE}, {"Drive"=enum."Idle", "Direction"=FALSE, "Phase Step"=enum."Duration", "Duration [s]"=0.0, "Current High [A]"=0.0, "Current Low [A]"=0.0, "Voltage High [V]"=0.0, "Voltage Low [V]"=0.0, "Change"=FALSE, "Current Control"=enum."Closed Loop", "Period [s]"=0.0, "Pulse Width [s]"=0.0, "Profile"=0, "Voltage Control"=FALSE}, {"Drive"=enum."Idle", "Direction"=FALSE, "Phase Step"=enum."Duration", "Duration [s]"=0.0, "Current High [A]"=0.0, "Current Low [A]"=0.0, "Voltage High [V]"=0.0, "Voltage Low [V]"=0.0, "Change"=FALSE, "Current Control"=enum."Closed Loop", "Period [s]"=0.0, "Pulse Width [s]"=0.0, "Profile"=0, "Voltage Control"=FALSE}, {"Drive"=enum."Idle", "Direction"=FALSE, "Phase Step"=enum."Duration", "Duration [s]"=0.0, "Current High [A]"=0.0, "Current Low [A]"=0.0, "Voltage High [V]"=0.0, "Voltage Low [V]"=0.0, "Change"=FALSE, "Current Control"=enum."Closed Loop", "Period [s]"=0.0, "Pulse Width [s]"=0.0, "Profile"=0, "Voltage Control"=FALSE}, {"Drive"=enum."Idle", "Direction"=FALSE, "Phase Step"=enum."Duration", "Duration [s]"=0.0, "Current High [A]"=0.0, "Current Low [A]"=0.0, "Voltage High [V]"=0.0, "Voltage Low [V]"=0.0, "Change"=FALSE, "Current Control"=enum."Closed Loop", "Period [s]"=0.0, "Pulse Width [s]"=0.0, "Profile"=0, "Voltage Control"=FALSE}], [{"Drive"=enum."Idle", "Direction"=FALSE, "Phase Step"=enum."Duration", "Duration [s]"=0.0, "Current High [A]"=0.0, "Current Low [A]"=0.0, "Voltage High [V]"=0.0, "Voltage Low [V]"=0.0, "Change"=FALSE, "Current Control"=enum."Closed Loop", "Period [s]"=0.0, "Pulse Width [s]"=0.0, "Profile"=0, "Voltage Control"=FALSE}, {"Drive"=enum."Idle", "Direction"=FALSE, "Phase Step"=enum."Duration", "Duration [s]"=0.0, "Current High [A]"=0.0, "Current Low [A]"=0.0, "Voltage High [V]"=0.0, "Voltage Low [V]"=0.0, "Change"=FALSE, "Current Control"=enum."Closed Loop", "Period [s]"=0.0, "Pulse Width [s]"=0.0, "Profile"=0, "Voltage Control"=FALSE}, {"Drive"=enum."Idle", "Direction"=FALSE, "Phase Step"=enum."Duration", "Duration [s]"=0.0, "Current High [A]"=0.0, "Current Low [A]"=0.0, "Voltage High [V]"=0.0, "Voltage Low [V]"=0.0, "Change"=FALSE, "Current Control"=enum."Closed Loop", "Period [s]"=0.0, "Pulse Width [s]"=0.0, "Profile"=0, "Voltage Control"=FALSE}, {"Drive"=enum."Idle", "Direction"=FALSE, "Phase Step"=enum."Duration", "Duration [s]"=0.0, "Current High [A]"=0.0, "Current Low [A]"=0.0, "Voltage High [V]"=0.0, "Voltage Low [V]"=0.0, "Change"=FALSE, "Current Control"=enum."Closed Loop", "Period [s]"=0.0, "Pulse Width [s]"=0.0, "Profile"=0, "Voltage Control"=FALSE}, {"Drive"=enum."Idle", "Direction"=FALSE, "Phase Step"=enum."Duration", "Duration [s]"=0.0, "Current High [A]"=0.0, "Current Low [A]"=0.0, "Voltage High [V]"=0.0, "Voltage Low [V]"=0.0, "Change"=FALSE, "Current Control"=enum."Closed Loop", "Period [s]"=0.0, "Pulse Width [s]"=0.0, "Profile"=0, "Voltage Control"=FALSE}, {"Drive"=enum."Idle", "Direction"=FALSE, "Phase Step"=enum."Duration", "Duration [s]"=0.0, "Current High [A]"=0.0, "Current Low [A]"=0.0, "Voltage High [V]"=0.0, "Voltage Low [V]"=0.0, "Change"=FALSE, "Current Control"=enum."Closed Loop", "Period [s]"=0.0, "Pulse Width [s]"=0.0, "Profile"=0, "Voltage Control"=FALSE}, {"Drive"=enum."Idle", "Direction"=FALSE, "Phase Step"=enum."Duration", "Duration [s]"=0.0, "Current High [A]"=0.0, "Current Low [A]"=0.0, "Voltage High [V]"=0.0, "Voltage Low [V]"=0.0, "Change"=FALSE, "Current Control"=enum."Closed Loop", "Period [s]"=0.0, "Pulse Width [s]"=0.0, "Profile"=0, "Voltage Control"=FALSE}, {"Drive"=enum."Idle", "Direction"=FALSE, "Phase Step"=enum."Duration", "Duration [s]"=0.0, "Current High [A]"=0.0, "Current Low [A]"=0.0, "Voltage High [V]"=0.0, "Voltage Low [V]"=0.0, "Change"=FALSE, "Current Control"=enum."Closed Loop", "Period [s]"=0.0, "Pulse Width [s]"=0.0, "Profile"=0, "Voltage Control"=FALSE}, {"Drive"=enum."Idle", "Direction"=FALSE, "Phase Step"=enum."Duration", "Duration [s]"=0.0, "Current High [A]"=0.0, "Current Low [A]"=0.0, "Voltage High [V]"=0.0, "Voltage Low [V]"=0.0, "Change"=FALSE, "Current Control"=enum."Closed Loop", "Period [s]"=0.0, "Pulse Width [s]"=0.0, "Profile"=0, "Voltage Control"=FALSE}, {"Drive"=enum."Idle", "Direction"=FALSE, "Phase Step"=enum."Duration", "Duration [s]"=0.0, "Current High [A]"=0.0, "Current Low [A]"=0.0, "Voltage High [V]"=0.0, "Voltage Low [V]"=0.0, "Change"=FALSE, "Current Control"=enum."Closed Loop", "Period [s]"=0.0, "Pulse Width [s]"=0.0, "Profile"=0, "Voltage Control"=FALSE}, {"Drive"=enum."Idle", "Direction"=FALSE, "Phase Step"=enum."Duration", "Duration [s]"=0.0, "Current High [A]"=0.0, "Current Low [A]"=0.0, "Voltage High [V]"=0.0, "Voltage Low [V]"=0.0, "Change"=FALSE, "Current Control"=enum."Closed Loop", "Period [s]"=0.0, "Pulse Width [s]"=0.0, "Profile"=0, "Voltage Control"=FALSE}, {"Drive"=enum."Idle", "Direction"=FALSE, "Phase Step"=enum."Duration", "Duration [s]"=0.0, "Current High [A]"=0.0, "Current Low [A]"=0.0, "Voltage High [V]"=0.0, "Voltage Low [V]"=0.0, "Change"=FALSE, "Current Control"=enum."Closed Loop", "Period [s]"=0.0, "Pulse Width [s]"=0.0, "Profile"=0, "Voltage Control"=FALSE}, {"Drive"=enum."Idle", "Direction"=FALSE, "Phase Step"=enum."Duration", "Duration [s]"=0.0, "Current High [A]"=0.0, "Current Low [A]"=0.0, "Voltage High [V]"=0.0, "Voltage Low [V]"=0.0, "Change"=FALSE, "Current Control"=enum."Closed Loop", "Period [s]"=0.0, "Pulse Width [s]"=0.0, "Profile"=0, "Voltage Control"=FALSE}, {"Drive"=enum."Idle", "Direction"=FALSE, "Phase Step"=enum."Duration", "Duration [s]"=0.0, "Current High [A]"=0.0, "Current Low [A]"=0.0, "Voltage High [V]"=0.0, "Voltage Low [V]"=0.0, "Change"=FALSE, "Current Control"=enum."Closed Loop", "Period [s]"=0.0, "Pulse Width [s]"=0.0, "Profile"=0, "Voltage Control"=FALSE}, {"Drive"=enum."Idle", "Direction"=FALSE, "Phase Step"=enum."Duration", "Duration [s]"=0.0, "Current High [A]"=0.0, "Current Low [A]"=0.0, "Voltage High [V]"=0.0, "Voltage Low [V]"=0.0, "Change"=FALSE, "Current Control"=enum."Closed Loop", "Period [s]"=0.0, "Pulse Width [s]"=0.0, "Profile"=0, "Voltage Control"=FALSE}, {"Drive"=enum."Idle", "Direction"=FALSE, "Phase Step"=enum."Duration", "Duration [s]"=0.0, "Current High [A]"=0.0, "Current Low [A]"=0.0, "Voltage High [V]"=0.0, "Voltage Low [V]"=0.0, "Change"=FALSE, "Current Control"=enum."Closed Loop", "Period [s]"=0.0, "Pulse Width [s]"=0.0, "Profile"=0, "Voltage Control"=FALSE}], [{"Drive"=enum."Idle", "Direction"=FALSE, "Phase Step"=enum."Duration", "Duration [s]"=0.0, "Current High [A]"=0.0, "Current Low [A]"=0.0, "Voltage High [V]"=0.0, "Voltage Low [V]"=0.0, "Change"=FALSE, "Current Control"=enum."Closed Loop", "Period [s]"=0.0, "Pulse Width [s]"=0.0, "Profile"=0, "Voltage Control"=FALSE}, {"Drive"=enum."Idle", "Direction"=FALSE, "Phase Step"=enum."Duration", "Duration [s]"=0.0, "Current High [A]"=0.0, "Current Low [A]"=0.0, "Voltage High [V]"=0.0, "Voltage Low [V]"=0.0, "Change"=FALSE, "Current Control"=enum."Closed Loop", "Period [s]"=0.0, "Pulse Width [s]"=0.0, "Profile"=0, "Voltage Control"=FALSE}, {"Drive"=enum."Idle", "Direction"=FALSE, "Phase Step"=enum."Duration", "Duration [s]"=0.0, "Current High [A]"=0.0, "Current Low [A]"=0.0, "Voltage High [V]"=0.0, "Voltage Low [V]"=0.0, "Change"=FALSE, "Current Control"=enum."Closed Loop", "Period [s]"=0.0, "Pulse Width [s]"=0.0, "Profile"=0, "Voltage Control"=FALSE}, {"Drive"=enum."Idle", "Direction"=FALSE, "Phase Step"=enum."Duration", "Duration [s]"=0.0, "Current High [A]"=0.0, "Current Low [A]"=0.0, "Voltage High [V]"=0.0, "Voltage Low [V]"=0.0, "Change"=FALSE, "Current Control"=enum."Closed Loop", "Period [s]"=0.0, "Pulse Width [s]"=0.0, "Profile"=0, "Voltage Control"=FALSE}, {"Drive"=enum."Idle", "Direction"=FALSE, "Phase Step"=enum."Duration", "Duration [s]"=0.0, "Current High [A]"=0.0, "Current Low [A]"=0.0, "Voltage High [V]"=0.0, "Voltage Low [V]"=0.0, "Change"=FALSE, "Current Control"=enum."Closed Loop", "Period [s]"=0.0, "Pulse Width [s]"=0.0, "Profile"=0, "Voltage Control"=FALSE}, {"Drive"=enum."Idle", "Direction"=FALSE, "Phase Step"=enum."Duration", "Duration [s]"=0.0, "Current High [A]"=0.0, "Current Low [A]"=0.0, "Voltage High [V]"=0.0, "Voltage Low [V]"=0.0, "Change"=FALSE, "Current Control"=enum."Closed Loop", "Period [s]"=0.0, "Pulse Width [s]"=0.0, "Profile"=0, "Voltage Control"=FALSE}, {"Drive"=enum."Idle", "Direction"=FALSE, "Phase Step"=enum."Duration", "Duration [s]"=0.0, "Current High [A]"=0.0, "Current Low [A]"=0.0, "Voltage High [V]"=0.0, "Voltage Low [V]"=0.0, "Change"=FALSE, "Current Control"=enum."Closed Loop", "Period [s]"=0.0, "Pulse Width [s]"=0.0, "Profile"=0, "Voltage Control"=FALSE}, {"Drive"=enum."Idle", "Direction"=FALSE, "Phase Step"=enum."Duration", "Duration [s]"=0.0, "Current High [A]"=0.0, "Current Low [A]"=0.0, "Voltage High [V]"=0.0, "Voltage Low [V]"=0.0, "Change"=FALSE, "Current Control"=enum."Closed Loop", "Period [s]"=0.0, "Pulse Width [s]"=0.0, "Profile"=0, "Voltage Control"=FALSE}, {"Drive"=enum."Idle", "Direction"=FALSE, "Phase Step"=enum."Duration", "Duration [s]"=0.0, "Current High [A]"=0.0, "Current Low [A]"=0.0, "Voltage High [V]"=0.0, "Voltage Low [V]"=0.0, "Change"=FALSE, "Current Control"=enum."Closed Loop", "Period [s]"=0.0, "Pulse Width [s]"=0.0, "Profile"=0, "Voltage Control"=FALSE}, {"Drive"=enum."Idle", "Direction"=FALSE, "Phase Step"=enum."Duration", "Duration [s]"=0.0, "Current High [A]"=0.0, "Current Low [A]"=0.0, "Voltage High [V]"=0.0, "Voltage Low [V]"=0.0, "Change"=FALSE, "Current Control"=enum."Closed Loop", "Period [s]"=0.0, "Pulse Width [s]"=0.0, "Profile"=0, "Voltage Control"=FALSE}, {"Drive"=enum."Idle", "Direction"=FALSE, "Phase Step"=enum."Duration", "Duration [s]"=0.0, "Current High [A]"=0.0, "Current Low [A]"=0.0, "Voltage High [V]"=0.0, "Voltage Low [V]"=0.0, "Change"=FALSE, "Current Control"=enum."Closed Loop", "Period [s]"=0.0, "Pulse Width [s]"=0.0, "Profile"=0, "Voltage Control"=FALSE}, {"Drive"=enum."Idle", "Direction"=FALSE, "Phase Step"=enum."Duration", "Duration [s]"=0.0, "Current High [A]"=0.0, "Current Low [A]"=0.0, "Voltage High [V]"=0.0, "Voltage Low [V]"=0.0, "Change"=FALSE, "Current Control"=enum."Closed Loop", "Period [s]"=0.0, "Pulse Width [s]"=0.0, "Profile"=0, "Voltage Control"=FALSE}, {"Drive"=enum."Idle", "Direction"=FALSE, "Phase Step"=enum."Duration", "Duration [s]"=0.0, "Current High [A]"=0.0, "Current Low [A]"=0.0, "Voltage High [V]"=0.0, "Voltage Low [V]"=0.0, "Change"=FALSE, "Current Control"=enum."Closed Loop", "Period [s]"=0.0, "Pulse Width [s]"=0.0, "Profile"=0, "Voltage Control"=FALSE}, {"Drive"=enum."Idle", "Direction"=FALSE, "Phase Step"=enum."Duration", "Duration [s]"=0.0, "Current High [A]"=0.0, "Current Low [A]"=0.0, "Voltage High [V]"=0.0, "Voltage Low [V]"=0.0, "Change"=FALSE, "Current Control"=enum."Closed Loop", "Period [s]"=0.0, "Pulse Width [s]"=0.0, "Profile"=0, "Voltage Control"=FALSE}, {"Drive"=enum."Idle", "Direction"=FALSE, "Phase Step"=enum."Duration", "Duration [s]"=0.0, "Current High [A]"=0.0, "Current Low [A]"=0.0, "Voltage High [V]"=0.0, "Voltage Low [V]"=0.0, "Change"=FALSE, "Current Control"=enum."Closed Loop", "Period [s]"=0.0, "Pulse Width [s]"=0.0, "Profile"=0, "Voltage Control"=FALSE}, {"Drive"=enum."Idle", "Direction"=FALSE, "Phase Step"=enum."Duration", "Duration [s]"=0.0, "Current High [A]"=0.0, "Current Low [A]"=0.0, "Voltage High [V]"=0.0, "Voltage Low [V]"=0.0, "Change"=FALSE, "Current Control"=enum."Closed Loop", "Period [s]"=0.0, "Pulse Width [s]"=0.0, "Profile"=0, "Voltage Control"=FALSE}], [{"Drive"=enum."Idle", "Direction"=FALSE, "Phase Step"=enum."Duration", "Duration [s]"=0.0, "Current High [A]"=0.0, "Current Low [A]"=0.0, "Voltage High [V]"=0.0, "Voltage Low [V]"=0.0, "Change"=FALSE, "Current Control"=enum."Closed Loop", "Period [s]"=0.0, "Pulse Width [s]"=0.0, "Profile"=0, "Voltage Control"=FALSE}, {"Drive"=enum."Idle", "Direction"=FALSE, "Phase Step"=enum."Duration", "Duration [s]"=0.0, "Current High [A]"=0.0, "Current Low [A]"=0.0, "Voltage High [V]"=0.0, "Voltage Low [V]"=0.0, "Change"=FALSE, "Current Control"=enum."Closed Loop", "Period [s]"=0.0, "Pulse Width [s]"=0.0, "Profile"=0, "Voltage Control"=FALSE}, {"Drive"=enum."Idle", "Direction"=FALSE, "Phase Step"=enum."Duration", "Duration [s]"=0.0, "Current High [A]"=0.0, "Current Low [A]"=0.0, "Voltage High [V]"=0.0, "Voltage Low [V]"=0.0, "Change"=FALSE, "Current Control"=enum."Closed Loop", "Period [s]"=0.0, "Pulse Width [s]"=0.0, "Profile"=0, "Voltage Control"=FALSE}, {"Drive"=enum."Idle", "Direction"=FALSE, "Phase Step"=enum."Duration", "Duration [s]"=0.0, "Current High [A]"=0.0, "Current Low [A]"=0.0, "Voltage High [V]"=0.0, "Voltage Low [V]"=0.0, "Change"=FALSE, "Current Control"=enum."Closed Loop", "Period [s]"=0.0, "Pulse Width [s]"=0.0, "Profile"=0, "Voltage Control"=FALSE}, {"Drive"=enum."Idle", "Direction"=FALSE, "Phase Step"=enum."Duration", "Duration [s]"=0.0, "Current High [A]"=0.0, "Current Low [A]"=0.0, "Voltage High [V]"=0.0, "Voltage Low [V]"=0.0, "Change"=FALSE, "Current Control"=enum."Closed Loop", "Period [s]"=0.0, "Pulse Width [s]"=0.0, "Profile"=0, "Voltage Control"=FALSE}, {"Drive"=enum."Idle", "Direction"=FALSE, "Phase Step"=enum."Duration", "Duration [s]"=0.0, "Current High [A]"=0.0, "Current Low [A]"=0.0, "Voltage High [V]"=0.0, "Voltage Low [V]"=0.0, "Change"=FALSE, "Current Control"=enum."Closed Loop", "Period [s]"=0.0, "Pulse Width [s]"=0.0, "Profile"=0, "Voltage Control"=FALSE}, {"Drive"=enum."Idle", "Direction"=FALSE, "Phase Step"=enum."Duration", "Duration [s]"=0.0, "Current High [A]"=0.0, "Current Low [A]"=0.0, "Voltage High [V]"=0.0, "Voltage Low [V]"=0.0, "Change"=FALSE, "Current Control"=enum."Closed Loop", "Period [s]"=0.0, "Pulse Width [s]"=0.0, "Profile"=0, "Voltage Control"=FALSE}, {"Drive"=enum."Idle", "Direction"=FALSE, "Phase Step"=enum."Duration", "Duration [s]"=0.0, "Current High [A]"=0.0, "Current Low [A]"=0.0, "Voltage High [V]"=0.0, "Voltage Low [V]"=0.0, "Change"=FALSE, "Current Control"=enum."Closed Loop", "Period [s]"=0.0, "Pulse Width [s]"=0.0, "Profile"=0, "Voltage Control"=FALSE}, {"Drive"=enum."Idle", "Direction"=FALSE, "Phase Step"=enum."Duration", "Duration [s]"=0.0, "Current High [A]"=0.0, "Current Low [A]"=0.0, "Voltage High [V]"=0.0, "Voltage Low [V]"=0.0, "Change"=FALSE, "Current Control"=enum."Closed Loop", "Period [s]"=0.0, "Pulse Width [s]"=0.0, "Profile"=0, "Voltage Control"=FALSE}, {"Drive"=enum."Idle", "Direction"=FALSE, "Phase Step"=enum."Duration", "Duration [s]"=0.0, "Current High [A]"=0.0, "Current Low [A]"=0.0, "Voltage High [V]"=0.0, "Voltage Low [V]"=0.0, "Change"=FALSE, "Current Control"=enum."Closed Loop", "Period [s]"=0.0, "Pulse Width [s]"=0.0, "Profile"=0, "Voltage Control"=FALSE}, {"Drive"=enum."Idle", "Direction"=FALSE, "Phase Step"=enum."Duration", "Duration [s]"=0.0, "Current High [A]"=0.0, "Current Low [A]"=0.0, "Voltage High [V]"=0.0, "Voltage Low [V]"=0.0, "Change"=FALSE, "Current Control"=enum."Closed Loop", "Period [s]"=0.0, "Pulse Width [s]"=0.0, "Profile"=0, "Voltage Control"=FALSE}, {"Drive"=enum."Idle", "Direction"=FALSE, "Phase Step"=enum."Duration", "Duration [s]"=0.0, "Current High [A]"=0.0, "Current Low [A]"=0.0, "Voltage High [V]"=0.0, "Voltage Low [V]"=0.0, "Change"=FALSE, "Current Control"=enum."Closed Loop", "Period [s]"=0.0, "Pulse Width [s]"=0.0, "Profile"=0, "Voltage Control"=FALSE}, {"Drive"=enum."Idle", "Direction"=FALSE, "Phase Step"=enum."Duration", "Duration [s]"=0.0, "Current High [A]"=0.0, "Current Low [A]"=0.0, "Voltage High [V]"=0.0, "Voltage Low [V]"=0.0, "Change"=FALSE, "Current Control"=enum."Closed Loop", "Period [s]"=0.0, "Pulse Width [s]"=0.0, "Profile"=0, "Voltage Control"=FALSE}, {"Drive"=enum."Idle", "Direction"=FALSE, "Phase Step"=enum."Duration", "Duration [s]"=0.0, "Current High [A]"=0.0, "Current Low [A]"=0.0, "Voltage High [V]"=0.0, "Voltage Low [V]"=0.0, "Change"=FALSE, "Current Control"=enum."Closed Loop", "Period [s]"=0.0, "Pulse Width [s]"=0.0, "Profile"=0, "Voltage Control"=FALSE}, {"Drive"=enum."Idle", "Direction"=FALSE, "Phase Step"=enum."Duration", "Duration [s]"=0.0, "Current High [A]"=0.0, "Current Low [A]"=0.0, "Voltage High [V]"=0.0, "Voltage Low [V]"=0.0, "Change"=FALSE, "Current Control"=enum."Closed Loop", "Period [s]"=0.0, "Pulse Width [s]"=0.0, "Profile"=0, "Voltage Control"=FALSE}, {"Drive"=enum."Idle", "Direction"=FALSE, "Phase Step"=enum."Duration", "Duration [s]"=0.0, "Current High [A]"=0.0, "Current Low [A]"=0.0, "Voltage High [V]"=0.0, "Voltage Low [V]"=0.0, "Change"=FALSE, "Current Control"=enum."Closed Loop", "Period [s]"=0.0, "Pulse Width [s]"=0.0, "Profile"=0, "Voltage Control"=FALSE}], [{"Drive"=enum."Idle", "Direction"=FALSE, "Phase Step"=enum."Duration", "Duration [s]"=0.0, "Current High [A]"=0.0, "Current Low [A]"=0.0, "Voltage High [V]"=0.0, "Voltage Low [V]"=0.0, "Change"=FALSE, "Current Control"=enum."Closed Loop", "Period [s]"=0.0, "Pulse Width [s]"=0.0, "Profile"=0, "Voltage Control"=FALSE}, {"Drive"=enum."Idle", "Direction"=FALSE, "Phase Step"=enum."Duration", "Duration [s]"=0.0, "Current High [A]"=0.0, "Current Low [A]"=0.0, "Voltage High [V]"=0.0, "Voltage Low [V]"=0.0, "Change"=FALSE, "Current Control"=enum."Closed Loop", "Period [s]"=0.0, "Pulse Width [s]"=0.0, "Profile"=0, "Voltage Control"=FALSE}, {"Drive"=enum."Idle", "Direction"=FALSE, "Phase Step"=enum."Duration", "Duration [s]"=0.0, "Current High [A]"=0.0, "Current Low [A]"=0.0, "Voltage High [V]"=0.0, "Voltage Low [V]"=0.0, "Change"=FALSE, "Current Control"=enum."Closed Loop", "Period [s]"=0.0, "Pulse Width [s]"=0.0, "Profile"=0, "Voltage Control"=FALSE}, {"Drive"=enum."Idle", "Direction"=FALSE, "Phase Step"=enum."Duration", "Duration [s]"=0.0, "Current High [A]"=0.0, "Current Low [A]"=0.0, "Voltage High [V]"=0.0, "Voltage Low [V]"=0.0, "Change"=FALSE, "Current Control"=enum."Closed Loop", "Period [s]"=0.0, "Pulse Width [s]"=0.0, "Profile"=0, "Voltage Control"=FALSE}, {"Drive"=enum."Idle", "Direction"=FALSE, "Phase Step"=enum."Duration", "Duration [s]"=0.0, "Current High [A]"=0.0, "Current Low [A]"=0.0, "Voltage High [V]"=0.0, "Voltage Low [V]"=0.0, "Change"=FALSE, "Current Control"=enum."Closed Loop", "Period [s]"=0.0, "Pulse Width [s]"=0.0, "Profile"=0, "Voltage Control"=FALSE}, {"Drive"=enum."Idle", "Direction"=FALSE, "Phase Step"=enum."Duration", "Duration [s]"=0.0, "Current High [A]"=0.0, "Current Low [A]"=0.0, "Voltage High [V]"=0.0, "Voltage Low [V]"=0.0, "Change"=FALSE, "Current Control"=enum."Closed Loop", "Period [s]"=0.0, "Pulse Width [s]"=0.0, "Profile"=0, "Voltage Control"=FALSE}, {"Drive"=enum."Idle", "Direction"=FALSE, "Phase Step"=enum."Duration", "Duration [s]"=0.0, "Current High [A]"=0.0, "Current Low [A]"=0.0, "Voltage High [V]"=0.0, "Voltage Low [V]"=0.0, "Change"=FALSE, "Current Control"=enum."Closed Loop", "Period [s]"=0.0, "Pulse Width [s]"=0.0, "Profile"=0, "Voltage Control"=FALSE}, {"Drive"=enum."Idle", "Direction"=FALSE, "Phase Step"=enum."Duration", "Duration [s]"=0.0, "Current High [A]"=0.0, "Current Low [A]"=0.0, "Voltage High [V]"=0.0, "Voltage Low [V]"=0.0, "Change"=FALSE, "Current Control"=enum."Closed Loop", "Period [s]"=0.0, "Pulse Width [s]"=0.0, "Profile"=0, "Voltage Control"=FALSE}, {"Drive"=enum."Idle", "Direction"=FALSE, "Phase Step"=enum."Duration", "Duration [s]"=0.0, "Current High [A]"=0.0, "Current Low [A]"=0.0, "Voltage High [V]"=0.0, "Voltage Low [V]"=0.0, "Change"=FALSE, "Current Control"=enum."Closed Loop", "Period [s]"=0.0, "Pulse Width [s]"=0.0, "Profile"=0, "Voltage Control"=FALSE}, {"Drive"=enum."Idle", "Direction"=FALSE, "Phase Step"=enum."Duration", "Duration [s]"=0.0, "Current High [A]"=0.0, "Current Low [A]"=0.0, "Voltage High [V]"=0.0, "Voltage Low [V]"=0.0, "Change"=FALSE, "Current Control"=enum."Closed Loop", "Period [s]"=0.0, "Pulse Width [s]"=0.0, "Profile"=0, "Voltage Control"=FALSE}, {"Drive"=enum."Idle", "Direction"=FALSE, "Phase Step"=enum."Duration", "Duration [s]"=0.0, "Current High [A]"=0.0, "Current Low [A]"=0.0, "Voltage High [V]"=0.0, "Voltage Low [V]"=0.0, "Change"=FALSE, "Current Control"=enum."Closed Loop", "Period [s]"=0.0, "Pulse Width [s]"=0.0, "Profile"=0, "Voltage Control"=FALSE}, {"Drive"=enum."Idle", "Direction"=FALSE, "Phase Step"=enum."Duration", "Duration [s]"=0.0, "Current High [A]"=0.0, "Current Low [A]"=0.0, "Voltage High [V]"=0.0, "Voltage Low [V]"=0.0, "Change"=FALSE, "Current Control"=enum."Closed Loop", "Period [s]"=0.0, "Pulse Width [s]"=0.0, "Profile"=0, "Voltage Control"=FALSE}, {"Drive"=enum."Idle", "Direction"=FALSE, "Phase Step"=enum."Duration", "Duration [s]"=0.0, "Current High [A]"=0.0, "Current Low [A]"=0.0, "Voltage High [V]"=0.0, "Voltage Low [V]"=0.0, "Change"=FALSE, "Current Control"=enum."Closed Loop", "Period [s]"=0.0, "Pulse Width [s]"=0.0, "Profile"=0, "Voltage Control"=FALSE}, {"Drive"=enum."Idle", "Direction"=FALSE, "Phase Step"=enum."Duration", "Duration [s]"=0.0, "Current High [A]"=0.0, "Current Low [A]"=0.0, "Voltage High [V]"=0.0, "Voltage Low [V]"=0.0, "Change"=FALSE, "Current Control"=enum."Closed Loop", "Period [s]"=0.0, "Pulse Width [s]"=0.0, "Profile"=0, "Voltage Control"=FALSE}, {"Drive"=enum."Idle", "Direction"=FALSE, "Phase Step"=enum."Duration", "Duration [s]"=0.0, "Current High [A]"=0.0, "Current Low [A]"=0.0, "Voltage High [V]"=0.0, "Voltage Low [V]"=0.0, "Change"=FALSE, "Current Control"=enum."Closed Loop", "Period [s]"=0.0, "Pulse Width [s]"=0.0, "Profile"=0, "Voltage Control"=FALSE}, {"Drive"=enum."Idle", "Direction"=FALSE, "Phase Step"=enum."Duration", "Duration [s]"=0.0, "Current High [A]"=0.0, "Current Low [A]"=0.0, "Voltage High [V]"=0.0, "Voltage Low [V]"=0.0, "Change"=FALSE, "Current Control"=enum."Closed Loop", "Period [s]"=0.0, "Pulse Width [s]"=0.0, "Profile"=0, "Voltage Control"=FALSE}], [{"Drive"=enum."Idle", "Direction"=FALSE, "Phase Step"=enum."Duration", "Duration [s]"=0.0, "Current High [A]"=0.0, "Current Low [A]"=0.0, "Voltage High [V]"=0.0, "Voltage Low [V]"=0.0, "Change"=FALSE, "Current Control"=enum."Closed Loop", "Period [s]"=0.0, "Pulse Width [s]"=0.0, "Profile"=0, "Voltage Control"=FALSE}, {"Drive"=enum."Idle", "Direction"=FALSE, "Phase Step"=enum."Duration", "Duration [s]"=0.0, "Current High [A]"=0.0, "Current Low [A]"=0.0, "Voltage High [V]"=0.0, "Voltage Low [V]"=0.0, "Change"=FALSE, "Current Control"=enum."Closed Loop", "Period [s]"=0.0, "Pulse Width [s]"=0.0, "Profile"=0, "Voltage Control"=FALSE}, {"Drive"=enum."Idle", "Direction"=FALSE, "Phase Step"=enum."Duration", "Duration [s]"=0.0, "Current High [A]"=0.0, "Current Low [A]"=0.0, "Voltage High [V]"=0.0, "Voltage Low [V]"=0.0, "Change"=FALSE, "Current Control"=enum."Closed Loop", "Period [s]"=0.0, "Pulse Width [s]"=0.0, "Profile"=0, "Voltage Control"=FALSE}, {"Drive"=enum."Idle", "Direction"=FALSE, "Phase Step"=enum."Duration", "Duration [s]"=0.0, "Current High [A]"=0.0, "Current Low [A]"=0.0, "Voltage High [V]"=0.0, "Voltage Low [V]"=0.0, "Change"=FALSE, "Current Control"=enum."Closed Loop", "Period [s]"=0.0, "Pulse Width [s]"=0.0, "Profile"=0, "Voltage Control"=FALSE}, {"Drive"=enum."Idle", "Direction"=FALSE, "Phase Step"=enum."Duration", "Duration [s]"=0.0, "Current High [A]"=0.0, "Current Low [A]"=0.0, "Voltage High [V]"=0.0, "Voltage Low [V]"=0.0, "Change"=FALSE, "Current Control"=enum."Closed Loop", "Period [s]"=0.0, "Pulse Width [s]"=0.0, "Profile"=0, "Voltage Control"=FALSE}, {"Drive"=enum."Idle", "Direction"=FALSE, "Phase Step"=enum."Duration", "Duration [s]"=0.0, "Current High [A]"=0.0, "Current Low [A]"=0.0, "Voltage High [V]"=0.0, "Voltage Low [V]"=0.0, "Change"=FALSE, "Current Control"=enum."Closed Loop", "Period [s]"=0.0, "Pulse Width [s]"=0.0, "Profile"=0, "Voltage Control"=FALSE}, {"Drive"=enum."Idle", "Direction"=FALSE, "Phase Step"=enum."Duration", "Duration [s]"=0.0, "Current High [A]"=0.0, "Current Low [A]"=0.0, "Voltage High [V]"=0.0, "Voltage Low [V]"=0.0, "Change"=FALSE, "Current Control"=enum."Closed Loop", "Period [s]"=0.0, "Pulse Width [s]"=0.0, "Profile"=0, "Voltage Control"=FALSE}, {"Drive"=enum."Idle", "Direction"=FALSE, "Phase Step"=enum."Duration", "Duration [s]"=0.0, "Current High [A]"=0.0, "Current Low [A]"=0.0, "Voltage High [V]"=0.0, "Voltage Low [V]"=0.0, "Change"=FALSE, "Current Control"=enum."Closed Loop", "Period [s]"=0.0, "Pulse Width [s]"=0.0, "Profile"=0, "Voltage Control"=FALSE}, {"Drive"=enum."Idle", "Direction"=FALSE, "Phase Step"=enum."Duration", "Duration [s]"=0.0, "Current High [A]"=0.0, "Current Low [A]"=0.0, "Voltage High [V]"=0.0, "Voltage Low [V]"=0.0, "Change"=FALSE, "Current Control"=enum."Closed Loop", "Period [s]"=0.0, "Pulse Width [s]"=0.0, "Profile"=0, "Voltage Control"=FALSE}, {"Drive"=enum."Idle", "Direction"=FALSE, "Phase Step"=enum."Duration", "Duration [s]"=0.0, "Current High [A]"=0.0, "Current Low [A]"=0.0, "Voltage High [V]"=0.0, "Voltage Low [V]"=0.0, "Change"=FALSE, "Current Control"=enum."Closed Loop", "Period [s]"=0.0, "Pulse Width [s]"=0.0, "Profile"=0, "Voltage Control"=FALSE}, {"Drive"=enum."Idle", "Direction"=FALSE, "Phase Step"=enum."Duration", "Duration [s]"=0.0, "Current High [A]"=0.0, "Current Low [A]"=0.0, "Voltage High [V]"=0.0, "Voltage Low [V]"=0.0, "Change"=FALSE, "Current Control"=enum."Closed Loop", "Period [s]"=0.0, "Pulse Width [s]"=0.0, "Profile"=0, "Voltage Control"=FALSE}, {"Drive"=enum."Idle", "Direction"=FALSE, "Phase Step"=enum."Duration", "Duration [s]"=0.0, "Current High [A]"=0.0, "Current Low [A]"=0.0, "Voltage High [V]"=0.0, "Voltage Low [V]"=0.0, "Change"=FALSE, "Current Control"=enum."Closed Loop", "Period [s]"=0.0, "Pulse Width [s]"=0.0, "Profile"=0, "Voltage Control"=FALSE}, {"Drive"=enum."Idle", "Direction"=FALSE, "Phase Step"=enum."Duration", "Duration [s]"=0.0, "Current High [A]"=0.0, "Current Low [A]"=0.0, "Voltage High [V]"=0.0, "Voltage Low [V]"=0.0, "Change"=FALSE, "Current Control"=enum."Closed Loop", "Period [s]"=0.0, "Pulse Width [s]"=0.0, "Profile"=0, "Voltage Control"=FALSE}, {"Drive"=enum."Idle", "Direction"=FALSE, "Phase Step"=enum."Duration", "Duration [s]"=0.0, "Current High [A]"=0.0, "Current Low [A]"=0.0, "Voltage High [V]"=0.0, "Voltage Low [V]"=0.0, "Change"=FALSE, "Current Control"=enum."Closed Loop", "Period [s]"=0.0, "Pulse Width [s]"=0.0, "Profile"=0, "Voltage Control"=FALSE}, {"Drive"=enum."Idle", "Direction"=FALSE, "Phase Step"=enum."Duration", "Duration [s]"=0.0, "Current High [A]"=0.0, "Current Low [A]"=0.0, "Voltage High [V]"=0.0, "Voltage Low [V]"=0.0, "Change"=FALSE, "Current Control"=enum."Closed Loop", "Period [s]"=0.0, "Pulse Width [s]"=0.0, "Profile"=0, "Voltage Control"=FALSE}, {"Drive"=enum."Idle", "Direction"=FALSE, "Phase Step"=enum."Duration", "Duration [s]"=0.0, "Current High [A]"=0.0, "Current Low [A]"=0.0, "Voltage High [V]"=0.0, "Voltage Low [V]"=0.0, "Change"=FALSE, "Current Control"=enum."Closed Loop", "Period [s]"=0.0, "Pulse Width [s]"=0.0, "Profile"=0, "Voltage Control"=FALSE}], [{"Drive"=enum."Idle", "Direction"=FALSE, "Phase Step"=enum."Duration", "Duration [s]"=0.0, "Current High [A]"=0.0, "Current Low [A]"=0.0, "Voltage High [V]"=0.0, "Voltage Low [V]"=0.0, "Change"=FALSE, "Current Control"=enum."Closed Loop", "Period [s]"=0.0, "Pulse Width [s]"=0.0, "Profile"=0, "Voltage Control"=FALSE}, {"Drive"=enum."Idle", "Direction"=FALSE, "Phase Step"=enum."Duration", "Duration [s]"=0.0, "Current High [A]"=0.0, "Current Low [A]"=0.0, "Voltage High [V]"=0.0, "Voltage Low [V]"=0.0, "Change"=FALSE, "Current Control"=enum."Closed Loop", "Period [s]"=0.0, "Pulse Width [s]"=0.0, "Profile"=0, "Voltage Control"=FALSE}, {"Drive"=enum."Idle", "Direction"=FALSE, "Phase Step"=enum."Duration", "Duration [s]"=0.0, "Current High [A]"=0.0, "Current Low [A]"=0.0, "Voltage High [V]"=0.0, "Voltage Low [V]"=0.0, "Change"=FALSE, "Current Control"=enum."Closed Loop", "Period [s]"=0.0, "Pulse Width [s]"=0.0, "Profile"=0, "Voltage Control"=FALSE}, {"Drive"=enum."Idle", "Direction"=FALSE, "Phase Step"=enum."Duration", "Duration [s]"=0.0, "Current High [A]"=0.0, "Current Low [A]"=0.0, "Voltage High [V]"=0.0, "Voltage Low [V]"=0.0, "Change"=FALSE, "Current Control"=enum."Closed Loop", "Period [s]"=0.0, "Pulse Width [s]"=0.0, "Profile"=0, "Voltage Control"=FALSE}, {"Drive"=enum."Idle", "Direction"=FALSE, "Phase Step"=enum."Duration", "Duration [s]"=0.0, "Current High [A]"=0.0, "Current Low [A]"=0.0, "Voltage High [V]"=0.0, "Voltage Low [V]"=0.0, "Change"=FALSE, "Current Control"=enum."Closed Loop", "Period [s]"=0.0, "Pulse Width [s]"=0.0, "Profile"=0, "Voltage Control"=FALSE}, {"Drive"=enum."Idle", "Direction"=FALSE, "Phase Step"=enum."Duration", "Duration [s]"=0.0, "Current High [A]"=0.0, "Current Low [A]"=0.0, "Voltage High [V]"=0.0, "Voltage Low [V]"=0.0, "Change"=FALSE, "Current Control"=enum."Closed Loop", "Period [s]"=0.0, "Pulse Width [s]"=0.0, "Profile"=0, "Voltage Control"=FALSE}, {"Drive"=enum."Idle", "Direction"=FALSE, "Phase Step"=enum."Duration", "Duration [s]"=0.0, "Current High [A]"=0.0, "Current Low [A]"=0.0, "Voltage High [V]"=0.0, "Voltage Low [V]"=0.0, "Change"=FALSE, "Current Control"=enum."Closed Loop", "Period [s]"=0.0, "Pulse Width [s]"=0.0, "Profile"=0, "Voltage Control"=FALSE}, {"Drive"=enum."Idle", "Direction"=FALSE, "Phase Step"=enum."Duration", "Duration [s]"=0.0, "Current High [A]"=0.0, "Current Low [A]"=0.0, "Voltage High [V]"=0.0, "Voltage Low [V]"=0.0, "Change"=FALSE, "Current Control"=enum."Closed Loop", "Period [s]"=0.0, "Pulse Width [s]"=0.0, "Profile"=0, "Voltage Control"=FALSE}, {"Drive"=enum."Idle", "Direction"=FALSE, "Phase Step"=enum."Duration", "Duration [s]"=0.0, "Current High [A]"=0.0, "Current Low [A]"=0.0, "Voltage High [V]"=0.0, "Voltage Low [V]"=0.0, "Change"=FALSE, "Current Control"=enum."Closed Loop", "Period [s]"=0.0, "Pulse Width [s]"=0.0, "Profile"=0, "Voltage Control"=FALSE}, {"Drive"=enum."Idle", "Direction"=FALSE, "Phase Step"=enum."Duration", "Duration [s]"=0.0, "Current High [A]"=0.0, "Current Low [A]"=0.0, "Voltage High [V]"=0.0, "Voltage Low [V]"=0.0, "Change"=FALSE, "Current Control"=enum."Closed Loop", "Period [s]"=0.0, "Pulse Width [s]"=0.0, "Profile"=0, "Voltage Control"=FALSE}, {"Drive"=enum."Idle", "Direction"=FALSE, "Phase Step"=enum."Duration", "Duration [s]"=0.0, "Current High [A]"=0.0, "Current Low [A]"=0.0, "Voltage High [V]"=0.0, "Voltage Low [V]"=0.0, "Change"=FALSE, "Current Control"=enum."Closed Loop", "Period [s]"=0.0, "Pulse Width [s]"=0.0, "Profile"=0, "Voltage Control"=FALSE}, {"Drive"=enum."Idle", "Direction"=FALSE, "Phase Step"=enum."Duration", "Duration [s]"=0.0, "Current High [A]"=0.0, "Current Low [A]"=0.0, "Voltage High [V]"=0.0, "Voltage Low [V]"=0.0, "Change"=FALSE, "Current Control"=enum."Closed Loop", "Period [s]"=0.0, "Pulse Width [s]"=0.0, "Profile"=0, "Voltage Control"=FALSE}, {"Drive"=enum."Idle", "Direction"=FALSE, "Phase Step"=enum."Duration", "Duration [s]"=0.0, "Current High [A]"=0.0, "Current Low [A]"=0.0, "Voltage High [V]"=0.0, "Voltage Low [V]"=0.0, "Change"=FALSE, "Current Control"=enum."Closed Loop", "Period [s]"=0.0, "Pulse Width [s]"=0.0, "Profile"=0, "Voltage Control"=FALSE}, {"Drive"=enum."Idle", "Direction"=FALSE, "Phase Step"=enum."Duration", "Duration [s]"=0.0, "Current High [A]"=0.0, "Current Low [A]"=0.0, "Voltage High [V]"=0.0, "Voltage Low [V]"=0.0, "Change"=FALSE, "Current Control"=enum."Closed Loop", "Period [s]"=0.0, "Pulse Width [s]"=0.0, "Profile"=0, "Voltage Control"=FALSE}, {"Drive"=enum."Idle", "Direction"=FALSE, "Phase Step"=enum."Duration", "Duration [s]"=0.0, "Current High [A]"=0.0, "Current Low [A]"=0.0, "Voltage High [V]"=0.0, "Voltage Low [V]"=0.0, "Change"=FALSE, "Current Control"=enum."Closed Loop", "Period [s]"=0.0, "Pulse Width [s]"=0.0, "Profile"=0, "Voltage Control"=FALSE}, {"Drive"=enum."Idle", "Direction"=FALSE, "Phase Step"=enum."Duration", "Duration [s]"=0.0, "Current High [A]"=0.0, "Current Low [A]"=0.0, "Voltage High [V]"=0.0, "Voltage Low [V]"=0.0, "Change"=FALSE, "Current Control"=enum."Closed Loop", "Period [s]"=0.0, "Pulse Width [s]"=0.0, "Profile"=0, "Voltage Control"=FALSE}], [{"Drive"=enum."Idle", "Direction"=FALSE, "Phase Step"=enum."Duration", "Duration [s]"=0.0, "Current High [A]"=0.0, "Current Low [A]"=0.0, "Voltage High [V]"=0.0, "Voltage Low [V]"=0.0, "Change"=FALSE, "Current Control"=enum."Closed Loop", "Period [s]"=0.0, "Pulse Width [s]"=0.0, "Profile"=0, "Voltage Control"=FALSE}, {"Drive"=enum."Idle", "Direction"=FALSE, "Phase Step"=enum."Duration", "Duration [s]"=0.0, "Current High [A]"=0.0, "Current Low [A]"=0.0, "Voltage High [V]"=0.0, "Voltage Low [V]"=0.0, "Change"=FALSE, "Current Control"=enum."Closed Loop", "Period [s]"=0.0, "Pulse Width [s]"=0.0, "Profile"=0, "Voltage Control"=FALSE}, {"Drive"=enum."Idle", "Direction"=FALSE, "Phase Step"=enum."Duration", "Duration [s]"=0.0, "Current High [A]"=0.0, "Current Low [A]"=0.0, "Voltage High [V]"=0.0, "Voltage Low [V]"=0.0, "Change"=FALSE, "Current Control"=enum."Closed Loop", "Period [s]"=0.0, "Pulse Width [s]"=0.0, "Profile"=0, "Voltage Control"=FALSE}, {"Drive"=enum."Idle", "Direction"=FALSE, "Phase Step"=enum."Duration", "Duration [s]"=0.0, "Current High [A]"=0.0, "Current Low [A]"=0.0, "Voltage High [V]"=0.0, "Voltage Low [V]"=0.0, "Change"=FALSE, "Current Control"=enum."Closed Loop", "Period [s]"=0.0, "Pulse Width [s]"=0.0, "Profile"=0, "Voltage Control"=FALSE}, {"Drive"=enum."Idle", "Direction"=FALSE, "Phase Step"=enum."Duration", "Duration [s]"=0.0, "Current High [A]"=0.0, "Current Low [A]"=0.0, "Voltage High [V]"=0.0, "Voltage Low [V]"=0.0, "Change"=FALSE, "Current Control"=enum."Closed Loop", "Period [s]"=0.0, "Pulse Width [s]"=0.0, "Profile"=0, "Voltage Control"=FALSE}, {"Drive"=enum."Idle", "Direction"=FALSE, "Phase Step"=enum."Duration", "Duration [s]"=0.0, "Current High [A]"=0.0, "Current Low [A]"=0.0, "Voltage High [V]"=0.0, "Voltage Low [V]"=0.0, "Change"=FALSE, "Current Control"=enum."Closed Loop", "Period [s]"=0.0, "Pulse Width [s]"=0.0, "Profile"=0, "Voltage Control"=FALSE}, {"Drive"=enum."Idle", "Direction"=FALSE, "Phase Step"=enum."Duration", "Duration [s]"=0.0, "Current High [A]"=0.0, "Current Low [A]"=0.0, "Voltage High [V]"=0.0, "Voltage Low [V]"=0.0, "Change"=FALSE, "Current Control"=enum."Closed Loop", "Period [s]"=0.0, "Pulse Width [s]"=0.0, "Profile"=0, "Voltage Control"=FALSE}, {"Drive"=enum."Idle", "Direction"=FALSE, "Phase Step"=enum."Duration", "Duration [s]"=0.0, "Current High [A]"=0.0, "Current Low [A]"=0.0, "Voltage High [V]"=0.0, "Voltage Low [V]"=0.0, "Change"=FALSE, "Current Control"=enum."Closed Loop", "Period [s]"=0.0, "Pulse Width [s]"=0.0, "Profile"=0, "Voltage Control"=FALSE}, {"Drive"=enum."Idle", "Direction"=FALSE, "Phase Step"=enum."Duration", "Duration [s]"=0.0, "Current High [A]"=0.0, "Current Low [A]"=0.0, "Voltage High [V]"=0.0, "Voltage Low [V]"=0.0, "Change"=FALSE, "Current Control"=enum."Closed Loop", "Period [s]"=0.0, "Pulse Width [s]"=0.0, "Profile"=0, "Voltage Control"=FALSE}, {"Drive"=enum."Idle", "Direction"=FALSE, "Phase Step"=enum."Duration", "Duration [s]"=0.0, "Current High [A]"=0.0, "Current Low [A]"=0.0, "Voltage High [V]"=0.0, "Voltage Low [V]"=0.0, "Change"=FALSE, "Current Control"=enum."Closed Loop", "Period [s]"=0.0, "Pulse Width [s]"=0.0, "Profile"=0, "Voltage Control"=FALSE}, {"Drive"=enum."Idle", "Direction"=FALSE, "Phase Step"=enum."Duration", "Duration [s]"=0.0, "Current High [A]"=0.0, "Current Low [A]"=0.0, "Voltage High [V]"=0.0, "Voltage Low [V]"=0.0, "Change"=FALSE, "Current Control"=enum."Closed Loop", "Period [s]"=0.0, "Pulse Width [s]"=0.0, "Profile"=0, "Voltage Control"=FALSE}, {"Drive"=enum."Idle", "Direction"=FALSE, "Phase Step"=enum."Duration", "Duration [s]"=0.0, "Current High [A]"=0.0, "Current Low [A]"=0.0, "Voltage High [V]"=0.0, "Voltage Low [V]"=0.0, "Change"=FALSE, "Current Control"=enum."Closed Loop", "Period [s]"=0.0, "Pulse Width [s]"=0.0, "Profile"=0, "Voltage Control"=FALSE}, {"Drive"=enum."Idle", "Direction"=FALSE, "Phase Step"=enum."Duration", "Duration [s]"=0.0, "Current High [A]"=0.0, "Current Low [A]"=0.0, "Voltage High [V]"=0.0, "Voltage Low [V]"=0.0, "Change"=FALSE, "Current Control"=enum."Closed Loop", "Period [s]"=0.0, "Pulse Width [s]"=0.0, "Profile"=0, "Voltage Control"=FALSE}, {"Drive"=enum."Idle", "Direction"=FALSE, "Phase Step"=enum."Duration", "Duration [s]"=0.0, "Current High [A]"=0.0, "Current Low [A]"=0.0, "Voltage High [V]"=0.0, "Voltage Low [V]"=0.0, "Change"=FALSE, "Current Control"=enum."Closed Loop", "Period [s]"=0.0, "Pulse Width [s]"=0.0, "Profile"=0, "Voltage Control"=FALSE}, {"Drive"=enum."Idle", "Direction"=FALSE, "Phase Step"=enum."Duration", "Duration [s]"=0.0, "Current High [A]"=0.0, "Current Low [A]"=0.0, "Voltage High [V]"=0.0, "Voltage Low [V]"=0.0, "Change"=FALSE, "Current Control"=enum."Closed Loop", "Period [s]"=0.0, "Pulse Width [s]"=0.0, "Profile"=0, "Voltage Control"=FALSE}, {"Drive"=enum."Idle", "Direction"=FALSE, "Phase Step"=enum."Duration", "Duration [s]"=0.0, "Current High [A]"=0.0, "Current Low [A]"=0.0, "Voltage High [V]"=0.0, "Voltage Low [V]"=0.0, "Change"=FALSE, "Current Control"=enum."Closed Loop", "Period [s]"=0.0, "Pulse Width [s]"=0.0, "Profile"=0, "Voltage Control"=FALSE}], [{"Drive"=enum."Idle", "Direction"=FALSE, "Phase Step"=enum."Duration", "Duration [s]"=0.0, "Current High [A]"=0.0, "Current Low [A]"=0.0, "Voltage High [V]"=0.0, "Voltage Low [V]"=0.0, "Change"=FALSE, "Current Control"=enum."Closed Loop", "Period [s]"=0.0, "Pulse Width [s]"=0.0, "Profile"=0, "Voltage Control"=FALSE}, {"Drive"=enum."Idle", "Direction"=FALSE, "Phase Step"=enum."Duration", "Duration [s]"=0.0, "Current High [A]"=0.0, "Current Low [A]"=0.0, "Voltage High [V]"=0.0, "Voltage Low [V]"=0.0, "Change"=FALSE, "Current Control"=enum."Closed Loop", "Period [s]"=0.0, "Pulse Width [s]"=0.0, "Profile"=0, "Voltage Control"=FALSE}, {"Drive"=enum."Idle", "Direction"=FALSE, "Phase Step"=enum."Duration", "Duration [s]"=0.0, "Current High [A]"=0.0, "Current Low [A]"=0.0, "Voltage High [V]"=0.0, "Voltage Low [V]"=0.0, "Change"=FALSE, "Current Control"=enum."Closed Loop", "Period [s]"=0.0, "Pulse Width [s]"=0.0, "Profile"=0, "Voltage Control"=FALSE}, {"Drive"=enum."Idle", "Direction"=FALSE, "Phase Step"=enum."Duration", "Duration [s]"=0.0, "Current High [A]"=0.0, "Current Low [A]"=0.0, "Voltage High [V]"=0.0, "Voltage Low [V]"=0.0, "Change"=FALSE, "Current Control"=enum."Closed Loop", "Period [s]"=0.0, "Pulse Width [s]"=0.0, "Profile"=0, "Voltage Control"=FALSE}, {"Drive"=enum."Idle", "Direction"=FALSE, "Phase Step"=enum."Duration", "Duration [s]"=0.0, "Current High [A]"=0.0, "Current Low [A]"=0.0, "Voltage High [V]"=0.0, "Voltage Low [V]"=0.0, "Change"=FALSE, "Current Control"=enum."Closed Loop", "Period [s]"=0.0, "Pulse Width [s]"=0.0, "Profile"=0, "Voltage Control"=FALSE}, {"Drive"=enum."Idle", "Direction"=FALSE, "Phase Step"=enum."Duration", "Duration [s]"=0.0, "Current High [A]"=0.0, "Current Low [A]"=0.0, "Voltage High [V]"=0.0, "Voltage Low [V]"=0.0, "Change"=FALSE, "Current Control"=enum."Closed Loop", "Period [s]"=0.0, "Pulse Width [s]"=0.0, "Profile"=0, "Voltage Control"=FALSE}, {"Drive"=enum."Idle", "Direction"=FALSE, "Phase Step"=enum."Duration", "Duration [s]"=0.0, "Current High [A]"=0.0, "Current Low [A]"=0.0, "Voltage High [V]"=0.0, "Voltage Low [V]"=0.0, "Change"=FALSE, "Current Control"=enum."Closed Loop", "Period [s]"=0.0, "Pulse Width [s]"=0.0, "Profile"=0, "Voltage Control"=FALSE}, {"Drive"=enum."Idle", "Direction"=FALSE, "Phase Step"=enum."Duration", "Duration [s]"=0.0, "Current High [A]"=0.0, "Current Low [A]"=0.0, "Voltage High [V]"=0.0, "Voltage Low [V]"=0.0, "Change"=FALSE, "Current Control"=enum."Closed Loop", "Period [s]"=0.0, "Pulse Width [s]"=0.0, "Profile"=0, "Voltage Control"=FALSE}, {"Drive"=enum."Idle", "Direction"=FALSE, "Phase Step"=enum."Duration", "Duration [s]"=0.0, "Current High [A]"=0.0, "Current Low [A]"=0.0, "Voltage High [V]"=0.0, "Voltage Low [V]"=0.0, "Change"=FALSE, "Current Control"=enum."Closed Loop", "Period [s]"=0.0, "Pulse Width [s]"=0.0, "Profile"=0, "Voltage Control"=FALSE}, {"Drive"=enum."Idle", "Direction"=FALSE, "Phase Step"=enum."Duration", "Duration [s]"=0.0, "Current High [A]"=0.0, "Current Low [A]"=0.0, "Voltage High [V]"=0.0, "Voltage Low [V]"=0.0, "Change"=FALSE, "Current Control"=enum."Closed Loop", "Period [s]"=0.0, "Pulse Width [s]"=0.0, "Profile"=0, "Voltage Control"=FALSE}, {"Drive"=enum."Idle", "Direction"=FALSE, "Phase Step"=enum."Duration", "Duration [s]"=0.0, "Current High [A]"=0.0, "Current Low [A]"=0.0, "Voltage High [V]"=0.0, "Voltage Low [V]"=0.0, "Change"=FALSE, "Current Control"=enum."Closed Loop", "Period [s]"=0.0, "Pulse Width [s]"=0.0, "Profile"=0, "Voltage Control"=FALSE}, {"Drive"=enum."Idle", "Direction"=FALSE, "Phase Step"=enum."Duration", "Duration [s]"=0.0, "Current High [A]"=0.0, "Current Low [A]"=0.0, "Voltage High [V]"=0.0, "Voltage Low [V]"=0.0, "Change"=FALSE, "Current Control"=enum."Closed Loop", "Period [s]"=0.0, "Pulse Width [s]"=0.0, "Profile"=0, "Voltage Control"=FALSE}, {"Drive"=enum."Idle", "Direction"=FALSE, "Phase Step"=enum."Duration", "Duration [s]"=0.0, "Current High [A]"=0.0, "Current Low [A]"=0.0, "Voltage High [V]"=0.0, "Voltage Low [V]"=0.0, "Change"=FALSE, "Current Control"=enum."Closed Loop", "Period [s]"=0.0, "Pulse Width [s]"=0.0, "Profile"=0, "Voltage Control"=FALSE}, {"Drive"=enum."Idle", "Direction"=FALSE, "Phase Step"=enum."Duration", "Duration [s]"=0.0, "Current High [A]"=0.0, "Current Low [A]"=0.0, "Voltage High [V]"=0.0, "Voltage Low [V]"=0.0, "Change"=FALSE, "Current Control"=enum."Closed Loop", "Period [s]"=0.0, "Pulse Width [s]"=0.0, "Profile"=0, "Voltage Control"=FALSE}, {"Drive"=enum."Idle", "Direction"=FALSE, "Phase Step"=enum."Duration", "Duration [s]"=0.0, "Current High [A]"=0.0, "Current Low [A]"=0.0, "Voltage High [V]"=0.0, "Voltage Low [V]"=0.0, "Change"=FALSE, "Current Control"=enum."Closed Loop", "Period [s]"=0.0, "Pulse Width [s]"=0.0, "Profile"=0, "Voltage Control"=FALSE}, {"Drive"=enum."Idle", "Direction"=FALSE, "Phase Step"=enum."Duration", "Duration [s]"=0.0, "Current High [A]"=0.0, "Current Low [A]"=0.0, "Voltage High [V]"=0.0, "Voltage Low [V]"=0.0, "Change"=FALSE, "Current Control"=enum."Closed Loop", "Period [s]"=0.0, "Pulse Width [s]"=0.0, "Profile"=0, "Voltage Control"=FALSE}]] {"Profile" max=15; "Period [s]" min=4e-06 max=0.000102 format="%#_3p"; "Pulse Width [s]" min=0 max=0.000102 format="%#_3p"; "Voltage Low [V]" min=-220 max=220 format="%#_3p"; "Voltage High [V]" min=-220 max=220 format="%#_3p"; "Current Low [A]" min=-40 max=40 format="%#_3p"; "Current High [A]" min=-40 max=40 format="%#_3p"; "Duration [s]" min=0 max=1.67772 format="%#_3p"}
  in  "_DI Scope Event":T18
  out "State":T19 {"System ADC"."Fan [V]" format="%#_3p"; "System ADC"."Primary B1B2 [V]" format="%#_3p"; "System ADC"."Primary B3B4 [V]" format="%#_3p"; "System ADC"."Primary A3A4 [V]" format="%#_3p"; "System ADC"."Primary A1A2 [V]" format="%#_3p"; "System ADC"."MPRD [V]" format="%#_3p"; "System ADC"."Ext HV B [V]" format="%#_3p"; "System ADC"."Ext HV A [V]" format="%#_3p"; "System ADC"."Pump Zener B [V]" format="%#_3p"; "System ADC"."Pump Zener A [V]" format="%#_3p"; "System ADC"."DI Zener B [V]" format="%#_3p"; "System ADC"."DI Zener A [V]" format="%#_3p"; "System ADC"."Key [V]" format="%#_3p"; "System ADC"."DRVP [V]" format="%#_3p"; "System ADC"."Battery [V]" format="%#_3p"; "System ADC"."FET Driver [V]" format="%#_3p"; "System ADC"."Secondary B1B2 [V]" format="%#_3p"; "System ADC"."Secondary B3B4 [V]" format="%#_3p"; "System ADC"."Secondary A3A4 [V]" format="%#_3p"; "System ADC"."Secondary A1A2 [V]" format="%#_3p"; "System ADC"."Primary Range [V]" format="%#_3p"; "System ADC"."Temp Boost B [C]" format="%#_3p"; "System ADC"."Temp Primary A [C]" format="%#_3p"; "System ADC"."Temp Secondary A [C]" format="%#_3p"; "System ADC"."Temp Fan Intake [C]" format="%#_3p"; "System ADC"."Temp CPU [C]" format="%#_3p"; "System ADC"."Temp DI Zener B [C]" format="%#_3p"; "System ADC"."Temp DI B [C]" format="%#_3p"; "System ADC"."Temp DI Zener A [C]" format="%#_3p"; "System ADC"."Temp DI A [C]" format="%#_3p"; "System ADC"."Temp HH 7-12 [C]" format="%#_3p"; "System ADC"."Temp HH 1-6 [C]" format="%#_3p"; "System ADC"."AI 12 [V]" format="%#_3p"; "System ADC"."AI 11 [V]" format="%#_3p"; "System ADC"."AI 10 [V]" format="%#_3p"; "System ADC"."AI 9 [V]" format="%#_3p"; "System ADC"."AI 8 [V]" format="%#_3p"; "System ADC"."AI 7 [V]" format="%#_3p"; "System ADC"."AI 6 [V]" format="%#_3p"; "System ADC"."AI 5 [V]" format="%#_3p"; "System ADC"."AI 4 [V]" format="%#_3p"; "System ADC"."AI 3 [V]" format="%#_3p"; "System ADC"."AI 2 [V]" format="%#_3p"; "System ADC"."AI 1 [V]" format="%#_3p"}
  in  "PumpZenerEnable":bool
  in  "_DI ADC Select":T22
  in  "_Tab Control":T23(tab)
  in  "DI-B Inj Ref Setup":T5(xcontrol)
  in  "_MovePhaseArrayListUp":bool
  in  "_MovePhaseArrayListDown":bool
  in  "_Remove Phase":bool
  in  "_Insert Phase":bool
  in  "Phase Array":i32(listbox)
  in  "PhaseArraysList":i32(listbox)
  out "_Phase Plot":cluster{"Array":dbl[], "Array":dbl[]}[](graph)
  in  "SimInjDuration":sgl=0.001 caption="Simulation Duration [s]" format="%#.3p"
  in  "_Phase":T13 caption="Phase" {"Profile" max=15; "Period [s]" min=4e-06 max=0.000102 format="%#_3p"; "Pulse Width [s]" min=0 max=0.000102 format="%#_3p"; "Voltage Low [V]" min=-220 max=220 format="%#_3p"; "Voltage High [V]" min=-220 max=220 format="%#_3p"; "Current Low [A]" min=-40 max=40 format="%#_3p"; "Current High [A]" min=-40 max=40 format="%#_3p"; "Duration [s]" min=0 max=1.67772 format="%#_3p"}
  in  "_Ref Inj FilePath":path caption="Reference Inj Profile File Path"
  in  "_Save Profile":bool
  in  "_Apply Profile":bool
  in  "DI-B Sim Settings":T5(xcontrol) caption="DI Scope"
  out "_Pump Phase Plot":cluster{"Array":dbl[], "Array":dbl[]}[](graph)
  in  "DI-B Pump Ref Setup":T5(xcontrol)
  in  "_Ref Pump Current Profile FilePath":path caption="Reference Pump Profile File Path"
  in  "_Remove Pump Phase":bool
  in  "_Insert Pump Phase":bool
  in  "PumpPhase Array":i32(listbox)
  in  "_Pump Phase":T13 caption="Pump Phase" {"Profile" max=15; "Period [s]" min=4e-06 max=0.000102 format="%#_3p"; "Pulse Width [s]" min=0 max=0.000102 format="%#_3p"; "Voltage Low [V]" min=-220 max=220 format="%#_3p"; "Voltage High [V]" min=-220 max=220 format="%#_3p"; "Current Low [A]" min=-40 max=40 format="%#_3p"; "Current High [A]" min=-40 max=40 format="%#_3p"; "Duration [s]" min=0 max=1.67772 format="%#_3p"}
  in  "SimPumpDuration":sgl=0.001 caption="Simulation Duration [s]" format="%#.3p"
  in  "DI-B Sim Settings":T5(xcontrol) caption="DI Scope"
  in  "ProfilesAdapt":bool
  out "_Profiles usage tracker":i32(listbox) caption="Profiles usage tracker [Profile, Phase]"
  in  "Profiles":sgl[][](array[numeric]) caption="[]" min=0 max=0.0001 format="%#_6p"
  in  "_InjAdaptMode":bool
  in  "_DI_CopyToAllChannelConf":bool
  in  "_ChannelConfigurationList":i32(listbox)
  in  "_InjCmd Element":T24={"Mode"=enum."Off", "Digital Input"=enum."Unused", "Default Profile Index"=0, "Cal Freq [Hz]"=0.0, "Cal Duration [s]"=0.0, "Cal Increment [s]"=0.0, "Cal Pulses"=0, "TMP Command Sequence"=[{"Duration [s]"=0.0, "CmdLevel"=FALSE, "Continue"=FALSE, "Profile Select"=0}, {"Duration [s]"=0.0, "CmdLevel"=FALSE, "Continue"=FALSE, "Profile Select"=0}, {"Duration [s]"=0.0, "CmdLevel"=FALSE, "Continue"=FALSE, "Profile Select"=0}, {"Duration [s]"=0.0, "CmdLevel"=FALSE, "Continue"=FALSE, "Profile Select"=0}, {"Duration [s]"=0.0, "CmdLevel"=FALSE, "Continue"=FALSE, "Profile Select"=0}, {"Duration [s]"=0.0, "CmdLevel"=FALSE, "Continue"=FALSE, "Profile Select"=0}, {"Duration [s]"=0.0, "CmdLevel"=FALSE, "Continue"=FALSE, "Profile Select"=0}, {"Duration [s]"=0.0, "CmdLevel"=FALSE, "Continue"=FALSE, "Profile Select"=0}], "EPT TDC Offset [CAD]"=0.0, "EPT Window Start [DBTDC]"=0.0, "EPT Window End [DBTDC]"=0.0, "EPT Angles"=[{"Enable"=FALSE, "Timing [CAD]"=0.0, "Duration [s]"=0.0, "Profile Select"=0}, {"Enable"=FALSE, "Timing [CAD]"=0.0, "Duration [s]"=0.0, "Profile Select"=0}, {"Enable"=FALSE, "Timing [CAD]"=0.0, "Duration [s]"=0.0, "Profile Select"=0}, {"Enable"=FALSE, "Timing [CAD]"=0.0, "Duration [s]"=0.0, "Profile Select"=0}, {"Enable"=FALSE, "Timing [CAD]"=0.0, "Duration [s]"=0.0, "Profile Select"=0}, {"Enable"=FALSE, "Timing [CAD]"=0.0, "Duration [s]"=0.0, "Profile Select"=0}, {"Enable"=FALSE, "Timing [CAD]"=0.0, "Duration [s]"=0.0, "Profile Select"=0}, {"Enable"=FALSE, "Timing [CAD]"=0.0, "Duration [s]"=0.0, "Profile Select"=0}], "EPT Skip Fire"=FALSE, "Skip Fire Index"=0, "EPT Precharge Duration [s]"=0.0, "EPT Precharge Profile Index"=0} {"EPT Precharge Profile Index" max=15; "EPT Precharge Duration [s]" min=0 format="%#_4p"; "EPT Angles"."Profile Select" max=15; "EPT Angles"."Duration [s]" min=0 max=1.677722 format="%#_4p"; "EPT Angles"."Timing [CAD]" min=-720 max=720 format="%#_3p"; "TMP Command Sequence"."Profile Select" max=15; "TMP Command Sequence"."Duration [s]" min=0 max=1.677722 format="%#_3p"; "Default Profile Index" max=15; "EPT Window End [DBTDC]" min=-720 max=720; "Skip Fire Index" max=15; "EPT Window Start [DBTDC]" min=-720 max=720; "EPT TDC Offset [CAD]" min=-720 max=720; "Cal Increment [s]" min=0 format="%#_4p"; "Cal Pulses" max=500; "Cal Duration [s]" min=0 max=1.677722 format="%#_4p"; "Cal Freq [Hz]" min=0 format="%#_4p"}
  in  "_Plot Selector (T=TMP, F=EPT)":bool
  out "_Timing Plot":cluster{sgl[], sgl[]}[](graph)
  in  "_Bank Wiring Diagram":T25
  in  "PumpCmd":T26={"Mode"=enum."Off", "Digital Input"=enum."Unused", "Default Profile Index"=0, "Cal Freq [Hz]"=0.0, "Cal Duration [s]"=0.0, "Cal Increment [s]"=0.0, "Cal Pulses"=0, "TMP Command Sequence"=[{"Duration [s]"=0.0, "CmdLevel"=FALSE, "Continue"=FALSE, "Profile Select"=0}, {"Duration [s]"=0.0, "CmdLevel"=FALSE, "Continue"=FALSE, "Profile Select"=0}, {"Duration [s]"=0.0, "CmdLevel"=FALSE, "Continue"=FALSE, "Profile Select"=0}, {"Duration [s]"=0.0, "CmdLevel"=FALSE, "Continue"=FALSE, "Profile Select"=0}, {"Duration [s]"=0.0, "CmdLevel"=FALSE, "Continue"=FALSE, "Profile Select"=0}, {"Duration [s]"=0.0, "CmdLevel"=FALSE, "Continue"=FALSE, "Profile Select"=0}, {"Duration [s]"=0.0, "CmdLevel"=FALSE, "Continue"=FALSE, "Profile Select"=0}, {"Duration [s]"=0.0, "CmdLevel"=FALSE, "Continue"=FALSE, "Profile Select"=0}], "EPT TDC Offset [CAD]"=0.0, "EPT Window Start [DBTDC]"=0.0, "EPT Window End [DBTDC]"=0.0, "EPT Angles"=[{"Enable"=FALSE, "Timing [CAD]"=0.0, "Duration [s]"=0.0, "Profile Select"=0}, {"Enable"=FALSE, "Timing [CAD]"=0.0, "Duration [s]"=0.0, "Profile Select"=0}, {"Enable"=FALSE, "Timing [CAD]"=0.0, "Duration [s]"=0.0, "Profile Select"=0}, {"Enable"=FALSE, "Timing [CAD]"=0.0, "Duration [s]"=0.0, "Profile Select"=0}, {"Enable"=FALSE, "Timing [CAD]"=0.0, "Duration [s]"=0.0, "Profile Select"=0}, {"Enable"=FALSE, "Timing [CAD]"=0.0, "Duration [s]"=0.0, "Profile Select"=0}, {"Enable"=FALSE, "Timing [CAD]"=0.0, "Duration [s]"=0.0, "Profile Select"=0}, {"Enable"=FALSE, "Timing [CAD]"=0.0, "Duration [s]"=0.0, "Profile Select"=0}], "EPT Skip Fire"=FALSE, "Skip Fire Index"=0, "EPT Precharge Duration [s]"=0.0, "EPT Precharge Profile Index"=0} {"EPT Precharge Profile Index" max=15; "EPT Precharge Duration [s]" min=0 format="%#_4p"; "EPT Angles"."Profile Select" max=15; "EPT Angles"."Duration [s]" min=0 max=1.677722 format="%#_4p"; "EPT Angles"."Timing [CAD]" min=-720 max=720 format="%#_3p"; "TMP Command Sequence"."Profile Select" max=15; "TMP Command Sequence"."Duration [s]" min=0 max=1.677722 format="%#_3p"; "Default Profile Index" max=15; "EPT Window End [DBTDC]" min=-720 max=720; "Skip Fire Index" max=15; "EPT Window Start [DBTDC]" min=-720 max=720; "EPT TDC Offset [CAD]" min=-720 max=720; "Cal Increment [s]" min=0 format="%#_4p"; "Cal Pulses" max=500; "Cal Duration [s]" min=0 max=1.677722 format="%#_4p"; "Cal Freq [Hz]" min=0 format="%#_4p"}
  in  "PumpAdaptMode":bool
  in  "_Pump A Plot Selector (T=TMP, F=EPT)":bool
  out "_Pump Timing Plot":cluster{sgl[], sgl[]}[](graph)
  out "_Temp DI":sgl(slide)=21.08 caption="[C]" scale=0.0..80.0 scale format="%#.4f"
  out "_Temp Boost Primary":sgl(slide)=100.0 caption="[C]" max=100 scale=0.0..80.0 scale format="%#_2f"
  out "_Temp DI Zener":sgl(slide)=21.08 caption="[C]" scale=0.0..80.0 scale format="%#.0f"
  in  "_DI-B Fault Clear":T27 caption="Bank A DI Fault Clear"
  out "Faults":T28[](array[typedef]) caption="DI Faults"
  # "DI Bank B Status"
  # "DI Bank B Configuration"
  # "Voltage [DV]"
  # "Voltage [V]"
  # "Sim Injection Duration [s]"
  # "Sim Pump Duration [s]"
  # "Injector Channel Command Configuration"
  # "Enable"
  # "Timing [DBTDC]"
  # "Duration [s]"
  # "Profile Index"
  # "Duration [s]"
  # "Level"
  # "Pause/Continue"
  # "Profile Index"
  # "Pump Channel Command Configuration"
  # "Enable"
  # "Timing [DBTDC]"
  # "Duration [s]"
  # "Profile Index"
  # "Duration [s]"
  # "Level"
  # "Pause/Continue"
  # "Profile Index"
  # "Temp DI"
  # "Temp DI Zener"
  # "Temp Boost"
  # "Bank B DI Fault Clear"
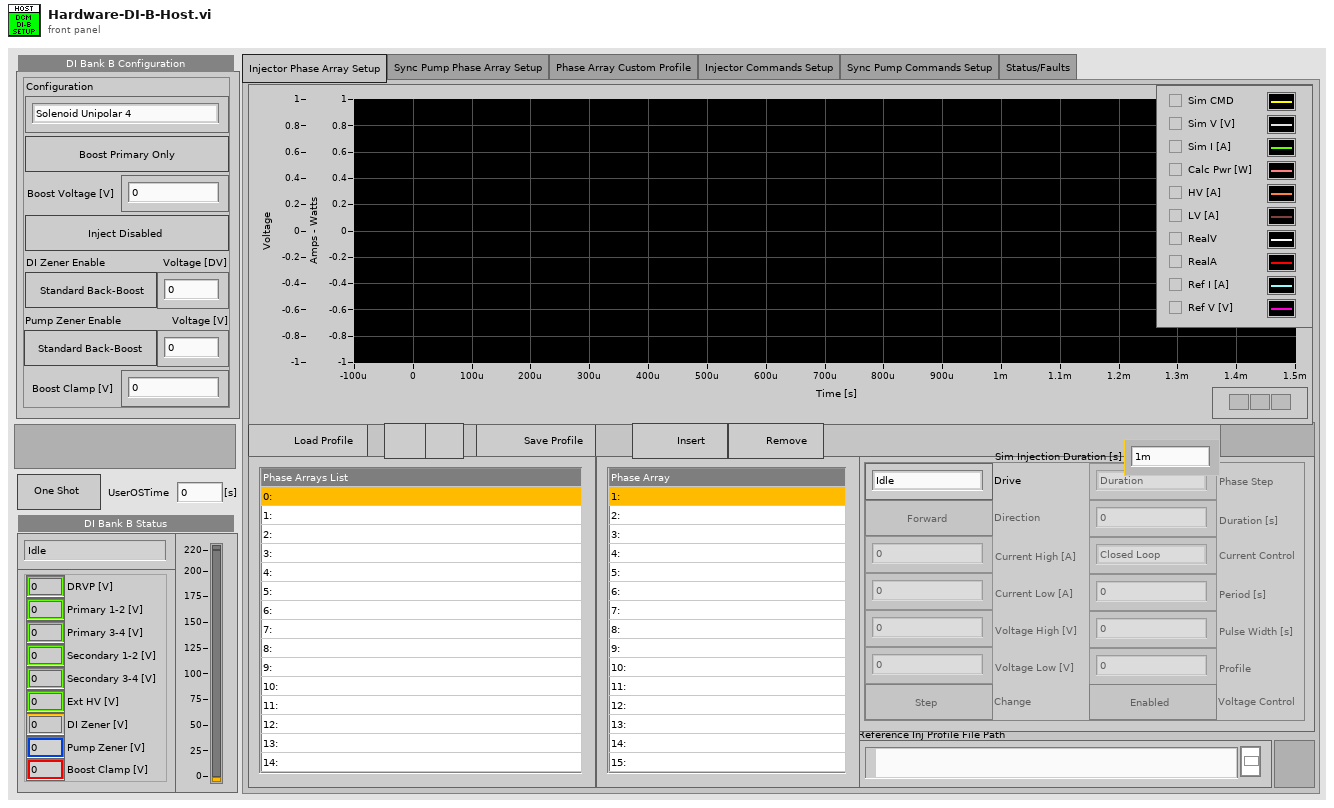
[diagram p1: front panel]
types:
  T1 = typedef "DCM - RT.lvclass/Run State.ctl" = enum8{"Idle", "Warmup", "Ready To Inject", "Cool Down"}
  T2 = cluster{"DRVP [V]":sgl, "Primary 1-2 [V]":sgl, "Primary 3-4 [V]":sgl, "Secondary 1-2 [V]":sgl, "Secondary 3-4 [V]":sgl, "Ext HV [V]":sgl, "DI Zener [V]":sgl, "Pump Zener [V]":sgl, "Boost Clamp [V]":sgl}
  T3 = typedef "DCM - RT.lvclass/Configuration.ctl" = cluster{"Configuration":T4, "Power Supply Enable":bool, "Boost Voltage [V]":sgl, "Inject Enable":bool, "DI Zener Enable":bool, "DI Zener Voltage [V]":sgl, "Pump Zener Enable":bool, "Pump Zener Voltage [V]":sgl, "Boost Clamp [V]":sgl}
  T4 = typedef "DCM - FPGA.lvlib/DI - Bank Configuration.ctl" = enum8{"Solenoid Unipolar 4", "Solenoid Unipolar 7 (Muxed)", "Solenoid Unipolar 8 (Muxed)", "Solenoid Bipolar 2", "Solenoid Bipolar 3 (Muxed)", "Piezo Unipolar 2", "Piezo Unipolar 3 (Muxed)", "Piezo Unipolar 4 (Muxed)", "Piezo Bipolar 2", "Piezo Bipolar 3 (Muxed)"}
  T5 = cluster{"Name":string, "Host VI":path, "Pairing File":path, "Display Name":string}
  T6 = typedef "DSI-Shared.lvlib/DI-Command-Array.ctl" = T7[]
  T7 = typedef "DCM - RT - DI.lvlib/Command.ctl" = cluster{"Mode":T8, "Digital Input":T9, "Default Profile Index":u8, "Cal Freq [Hz]":sgl, "Cal Duration [s]":sgl, "Cal Increment [s]":sgl, "Cal Pulses":u16, "TMP Command Sequence":T10[], "EPT TDC Offset [CAD]":sgl, "EPT Window Start [DBTDC]":sgl, "EPT Window End [DBTDC]":sgl, "EPT Angles":T11[], "EPT Skip Fire":bool, "EPT Skip Index":u8, "EPT Precharge Duration [s]":sgl, "EPT Precharge Profile Index":u8}
  T8 = typedef "DCM - FPGA - DI.lvlib/Mode.ctl" = enum8{"Off", "Direct", "Calibration", "Triggered Multi-Pulse", "Engine Position Tracking"}
  T9 = typedef "DCM - FPGA.lvlib/Digital Channel.ctl" = enum8{"Unused", "User OS", "Diff IO 1", "Diff IO 2", "Diff IO 3", "Diff IO 4", "Diff IO 5", "Diff IO 6", "Diff IO 7", "Diff IO 8", "Aux 1", "Aux 2", "Aux 3", "Aux 4", "Aux 5", "Aux 6", "Aux 7", "Aux 8", "Aux 9", "Aux 10", "Aux 11", "Aux 12", "Aux 13", "Aux 14", "Aux 15", "Aux 16"}
  T10 = typedef "DCM - RT - DI.lvlib/Command Sequence.ctl" = cluster{"Duration [s]":sgl, "Level":bool, "Run/Stop":bool, "Profile Index":u8}
  T11 = typedef "DCM - RT - DI.lvlib/Angle Control.ctl" = cluster{"Enable":bool, "Timing [DBTDC]":sgl, "Duration [s]":sgl, "Profile Index":u8}
  T12 = typedef "DSI-Shared.lvlib/DI-Phase-Array-1D.ctl" = T13[]
  T13 = typedef "DCM - RT - DI.lvlib/Phase.ctl" = cluster{"Drive":T14, "Direction":bool, "Phase Step":T15, "Duration [s]":sgl, "Current High [A]":sgl, "Current Low [A]":sgl, "Voltage High [V]":sgl, "Voltage Low [V]":sgl, "Change":bool, "Current Control":T16, "Period [s]":sgl, "Pulse Width [s]":sgl, "Profile":u8, "Voltage Control":bool}
  T14 = typedef "DCM - FPGA.lvlib/DI - Drive State.ctl" = enum8{"Idle", "HV Current Control", "LV Current Control", "Back Boost", "Piezo Charge", "Piezo Discharge"}
  T15 = typedef "DCM - FPGA - DI.lvlib/Phase Step.ctl" = enum8{"Duration", "First Peak", "End of Cmd", "Branch", "2-Phase Duration"}
  T16 = typedef "DCM - FPGA - DI.lvlib/Control.ctl" = enum8{"Closed Loop", "Fixed Period", "Fixed On Pulse", "Fixed Off Pulse", "Open Loop", "Profile"}
  T17 = typedef "DSI-Shared.lvlib/DI-Phase-Array-2D.ctl" = T13[][]
  T18 = typedef "DCM - FPGA - DI.lvlib/Capture Event.ctl" = enum8{"Unused", "Injector A1", "Injector A2", "Injector A3", "Injector A4", "Injector A5", "Injector A6", "Injector A7", "Injector A8/PumpA", "Injector B1", "Injector B2", "Injector B3", "Injector B4", "Injector B5", "Injector B6", "Injector B7", "Injector B8/PumpB", "User OS", "Diff IO 1", "Diff IO 2", "Diff IO 3", "Diff IO 4", "Diff IO 5", "Diff IO 6", "Diff IO 7", "Diff IO 8", "Aux 1", "Aux 2", "Aux 3", "Aux 4", "Aux 5", "Aux 6", "Aux 7", "Aux 8", "Aux 9", "Aux 10", "Aux 11", "Aux 12", "Aux 13", "Aux 14", "Aux 15", "Aux 16"}
  T19 = typedef "DCM - RT.lvclass/System State.ctl" = cluster{"System ADC":T20, "IO Lock":bool, "HH Mode Config Error":bool, "Fan Speed 1 [RPM]":sgl, "Fan Speed 2 [RPM]":sgl, "Firmware Major Rev":u16, "Firmware Minor Rev":u16, "Internal Fault":T21, "Fault Value":dbl}
  T20 = typedef "DCM - RT.lvclass/System ADC.ctl" = cluster{"AI 1 [V]":sgl, "AI 2 [V]":sgl, "AI 3 [V]":sgl, "AI 4 [V]":sgl, "AI 5 [V]":sgl, "AI 6 [V]":sgl, "AI 7 [V]":sgl, "AI 8 [V]":sgl, "AI 9 [V]":sgl, "AI 10 [V]":sgl, "AI 11 [V]":sgl, "AI 12 [V]":sgl, "Temp HH 1-6 [C]":sgl, "Temp HH 7-12 [C]":sgl, "Temp DI A [C]":sgl, "Temp DI Zener A [C]":sgl, "Temp DI B [C]":sgl, "Temp DI Zener B [C]":sgl, "Temp CPU [C]":sgl, "Temp Fan Intake [C]":sgl, "Temp Secondary A [C]":sgl, "Temp Primary A [C]":sgl, "Temp Boost B [C]":sgl, "Primary Range [V]":sgl, "Primary A1A2 [V]":sgl, "Primary A3A4 [V]":sgl, "Primary B3B4 [V]":sgl, "Primary B1B2 [V]":sgl, "Secondary A1A2 [V]":sgl, "Secondary A3A4 [V]":sgl, "Secondary B3B4 [V]":sgl, "Secondary B1B2 [V]":sgl, "Ext HV A [V]":sgl, "Ext HV B [V]":sgl, "FET Driver [V]":sgl, "Fan [V]":sgl, "Battery [V]":sgl, "DRVP [V]":sgl, "Key [V]":sgl, "DI Zener A [V]":sgl, "DI Zener B [V]":sgl, "Pump Zener A [V]":sgl, "Pump Zener B [V]":sgl, "MPRD [V]":sgl}
  T21 = typedef "DCM - RT.lvclass/Internal Fault.ctl" = enum32{"None", "Temp HH 1-6", "Temp HH 7-12", "Temp DI A", "Temp DI Zener A", "Temp DI B", "Temp DI Zener B", "Temp Intake", "Temp Primary A", "Temp Secondary A", "Temp Boost B", "Temp CPU", "Low Battery", "Inrush Protection", "A Run Enable", "B Run Enable"}
  T22 = typedef "DCM - FPGA.lvlib/DI - ADC Signals.ctl" = enum8{"I LS A1/A5", "I LS A2/A6", "I LS A3/A7", "I LS A4", "I LS A8/PumpA", "V PZ A1", "V PZ A2", "V PZ A3", "V PZ A4", "V S A1", "V S A2", "V S A3", "V S A4", "V S A5", "V S A6", "V S A7", "V S A8", "V Pump A", "V Secondary A1A2", "V Secondary A3A4", "V Ext HV A", "------------------------ ", "I LS B1/B5", "I LS B2/B6", "I LS B3/B7", "I LS B4", "I LS B8/PumpB", "V PZ B1", "V PZ B2", "V PZ B3", "V PZ B4", "V S B1", "V S B2", "V S B3", "V S B4", "V S B5", "V S B6", "V S B7", "V S B8", "V Pump B", "V Secondary B1B2", "V Secondary B3B4", "V Ext HV B", "-------------------------  ", "AI 1", "AI 2", "AI 3", "AI 4", "AI 5", "AI 6", "AI 7", "AI 8", "AI 9", "AI 10", "AI 11", "AI 12", "-------------------------   ", "V DRVP"}
  T23 = enum32{"Injector Phase Array Setup", "Sync Pump Phase Array Setup", "Phase Array Custom Profile", "Injector Commands Setup", "Sync Pump Commands Setup", "Status/Faults"}
  T24 = typedef "DI Command Element.ctl" = cluster{"Mode":enum8{"Off", "Direct", "Calibration", "Triggered Multi-Pulse", "Engine Position Tracking"}, "Digital Input":T9, "Default Profile Index":u8, "Cal Freq [Hz]":sgl, "Cal Duration [s]":sgl, "Cal Increment [s]":sgl, "Cal Pulses":u16, "TMP Command Sequence":cluster{"Duration [s]":sgl, "CmdLevel":bool, "Continue":bool, "Profile Select":u8}[], "EPT TDC Offset [CAD]":sgl, "EPT Window Start [DBTDC]":sgl, "EPT Window End [DBTDC]":sgl, "EPT Angles":cluster{"Enable":bool, "Timing [CAD]":sgl, "Duration [s]":sgl, "Profile Select":u8}[], "EPT Skip Fire":bool, "Skip Fire Index":u8, "EPT Precharge Duration [s]":sgl, "EPT Precharge Profile Index":u8}
  T25 = typedef "DCM - UI.lvlib/Bank B.ctl" = u8
  T26 = typedef "Pump Command Element.ctl" = cluster{"Mode":enum8{"Off", "Direct", "Calibration", "Triggered Multi-Pulse", "Engine Position Tracking"}, "Digital Input":T9, "Default Profile Index":u8, "Cal Freq [Hz]":sgl, "Cal Duration [s]":sgl, "Cal Increment [s]":sgl, "Cal Pulses":u16, "TMP Command Sequence":cluster{"Duration [s]":sgl, "CmdLevel":bool, "Continue":bool, "Profile Select":u8}[], "EPT TDC Offset [CAD]":sgl, "EPT Window Start [DBTDC]":sgl, "EPT Window End [DBTDC]":sgl, "EPT Angles":cluster{"Enable":bool, "Timing [CAD]":sgl, "Duration [s]":sgl, "Profile Select":u8}[], "EPT Skip Fire":bool, "Skip Fire Index":u8, "EPT Precharge Duration [s]":sgl, "EPT Precharge Profile Index":u8}
  T27 = cluster{"DI-B-1 Clear":bool, "DI-B-2 Clear":bool, "DI-B-3 Clear":bool, "DI-B-4 Clear":bool, "DI-B-5 Clear":bool, "DI-B-6 Clear":bool, "DI-B-7 Clear":bool, "DI-B-8 Clear":bool}
  T28 = typedef "DCM - FPGA.lvlib/DI - Faults.ctl" = cluster{"HV Fault":bool, "LV Fault":bool, "LS Fault":bool, "MUX Fault":bool, "Open Warning":bool}
  T29 = enum32{"Invalid", "Standard", "Closed", "Hidden", "Minimized", "Maximized"}
  T30 = enum8{"Enabled", "Disabled", "Disabled and Grayed Out"}
  T31 = cluster{"Configuration":T4, "Power Supply Enable":bool, "Boost Voltage [V]":sgl, "Inject Enable":bool, "Zener Enable":bool, "Zener Voltage [V]":sgl, "Pump Zener Enable":bool, "Pump Zener Voltage [V]":sgl, "Boost Clamp [V]":sgl}
  T32 = typedef "DCM - UI.lvlib/Configuration.ctl" = cluster{"Configuration":T4, "Boost Voltage [V]":sgl, "Zener Enable":bool, "Zener Voltage [V]":sgl}
  T33 = typedef "DCM - UI.lvlib/Injector Configuration.ctl" = cluster{"Resistance [Ohm]":sgl, "Inductance [Henery]":sgl, "Capacitance [Farad]":sgl}
  T34 = typedef "DCM - UI.lvlib/System Configuration.ctl" = cluster{"Battery [V]":sgl, "Engine Speed [RPM]":sgl, "Rotations":u8, "Injector Configuration":T33, "Description":string}
  T35 = cluster{"DRVP [V]":sgl, "Primary B1B2 [V]":sgl, "Primary B3B4 [V]":sgl, "Secondary B1B2 [V]":sgl, "Secondary B3B4 [V]":sgl, "Ext HV B [V]":sgl, "DI Zener B [V]":sgl, "Pump Zener B [V]":sgl, "BoostClampV":sgl}
  T36 = typedef "LVStringsAndValuesArrayTypeDef_U8.ctl" = cluster{"String":string, "Value":u8}[]
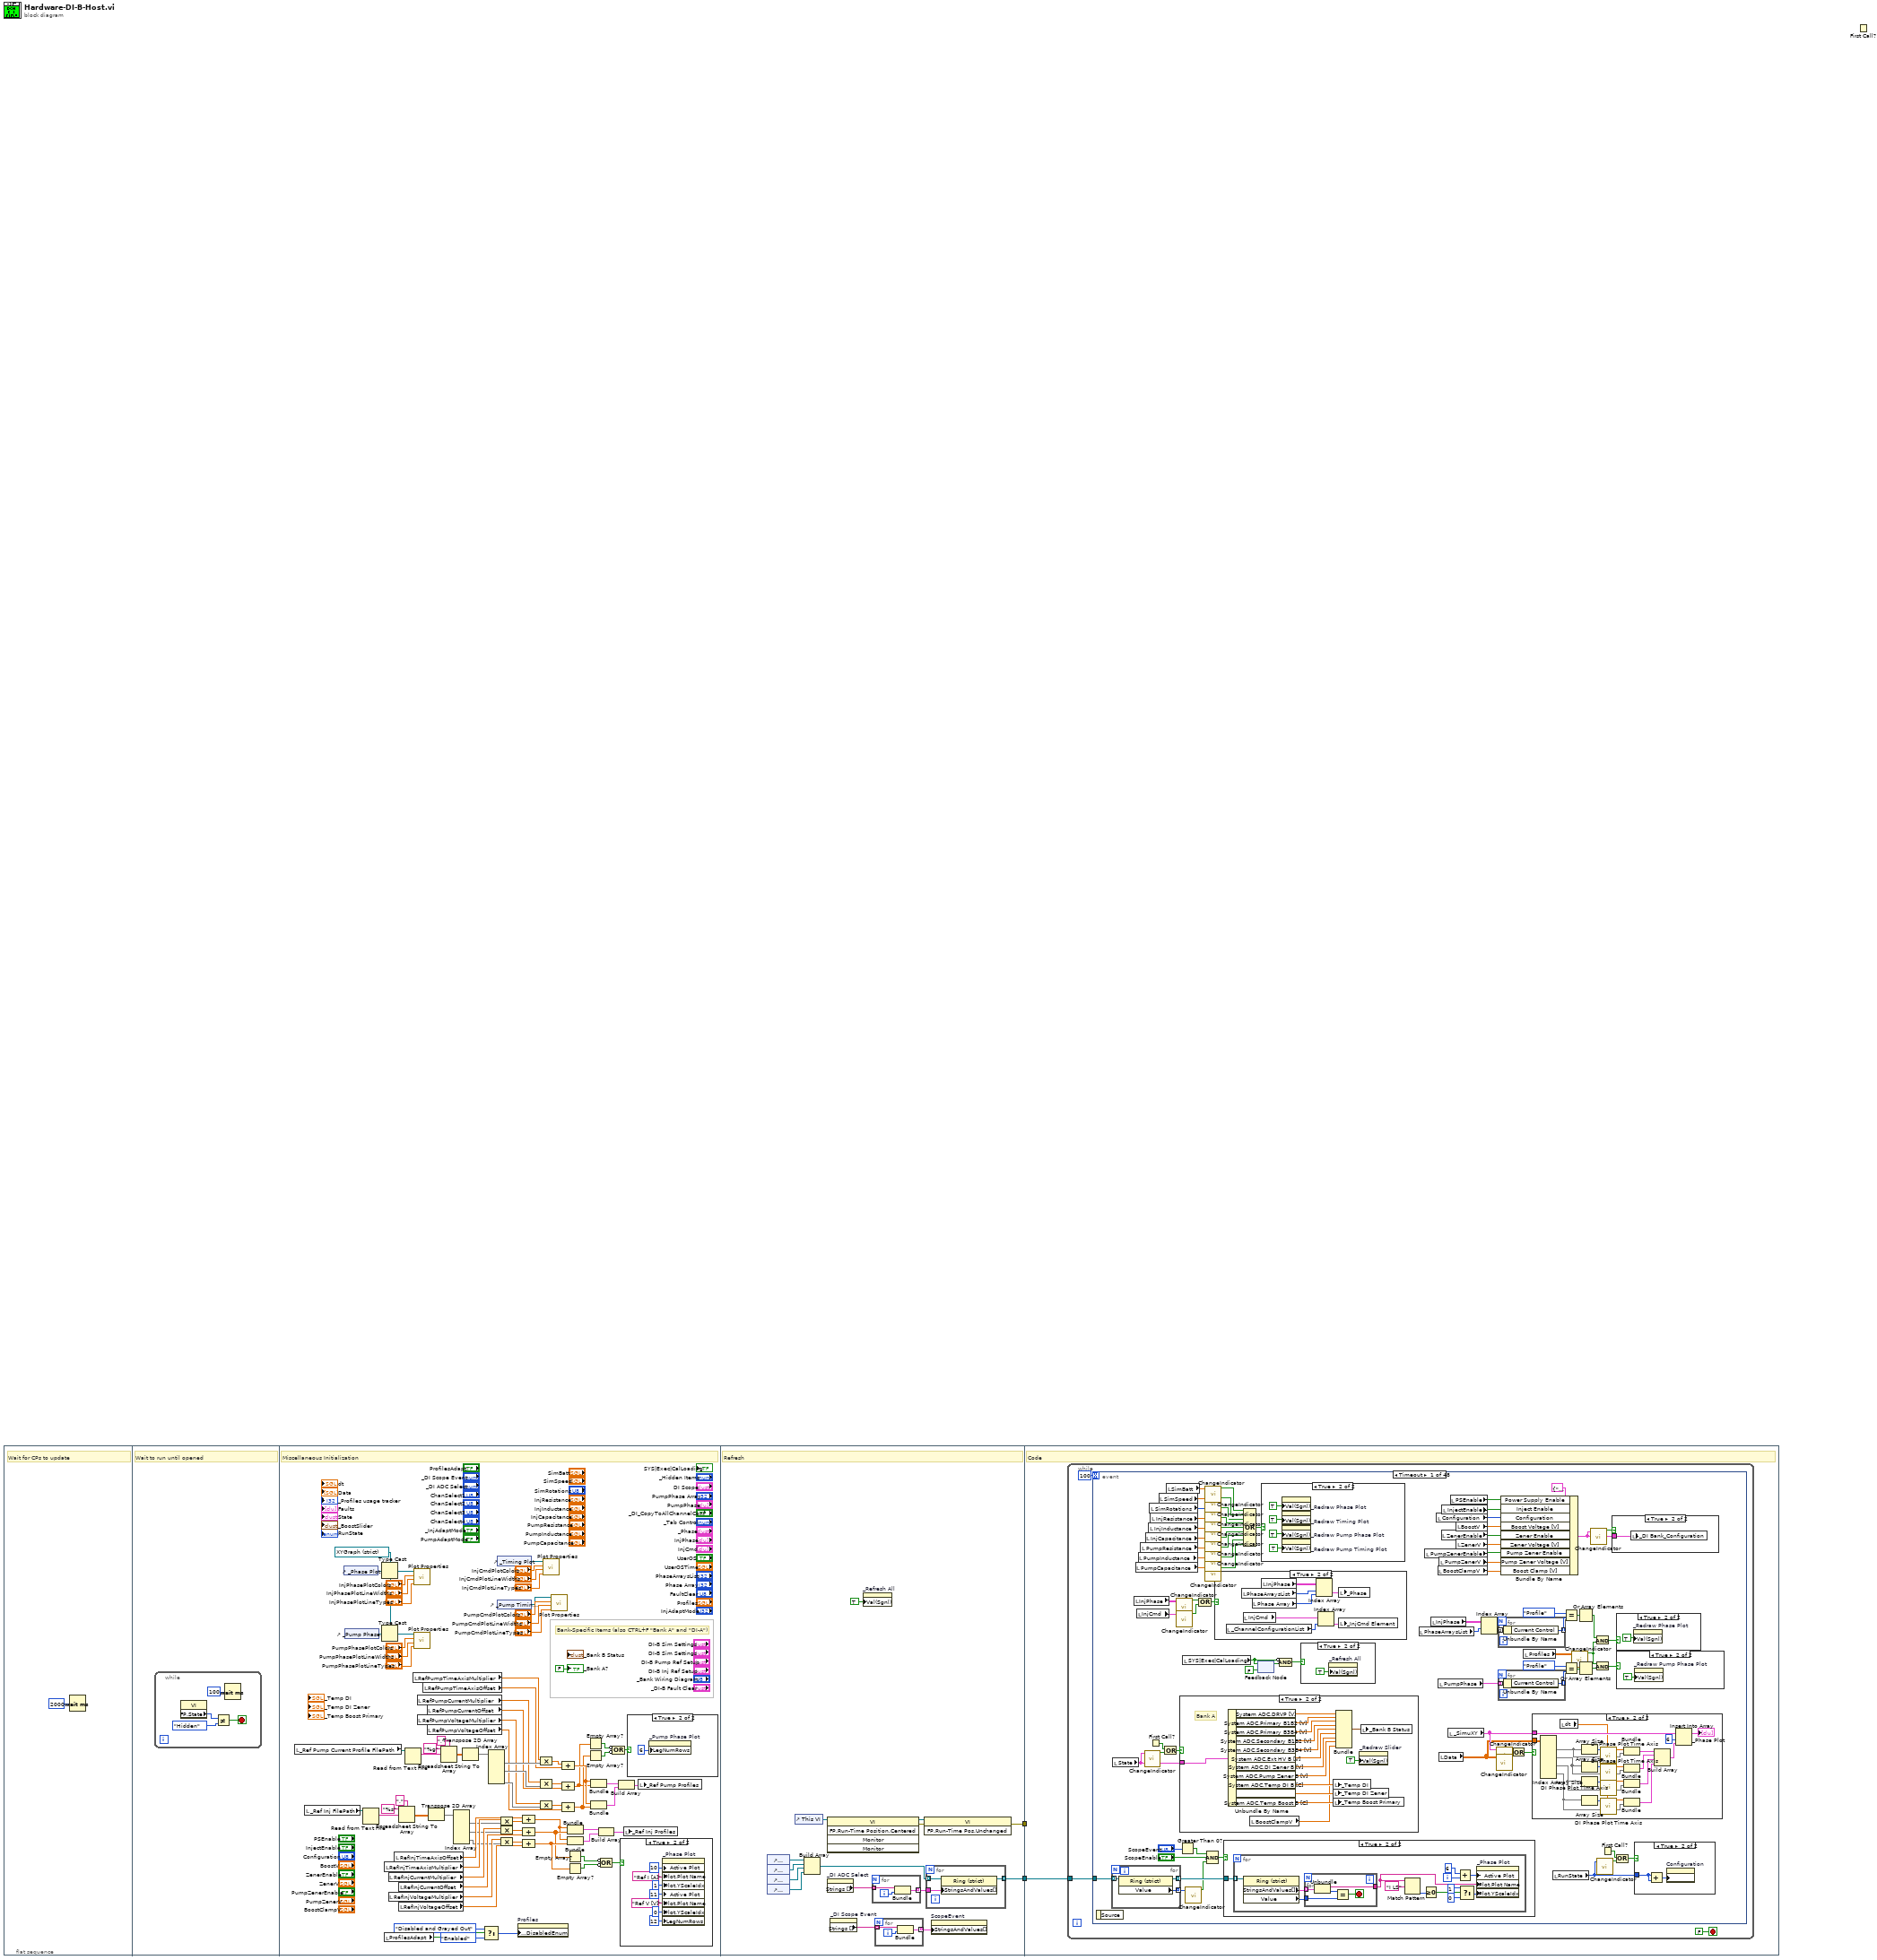
[diagram p0: block diagram]
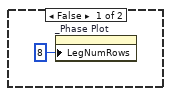
[diagram p2: hidden frame]
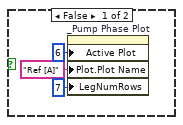
[diagram p3: hidden frame]
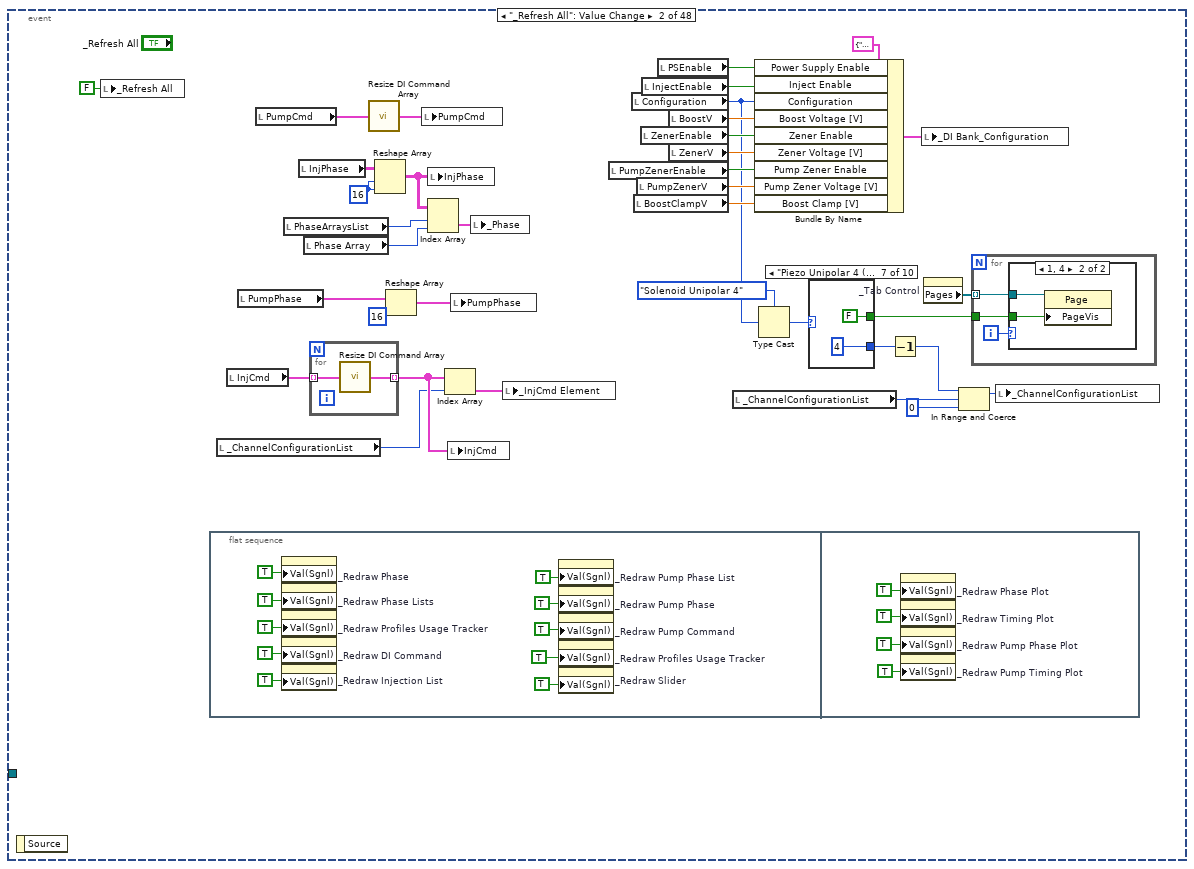
[diagram p14: hidden frame]
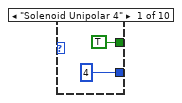
[diagram p15: hidden frame]
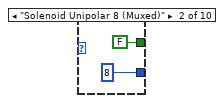
[diagram p16: hidden frame]
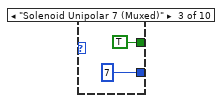
[diagram p17: hidden frame]
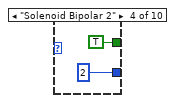
[diagram p18: hidden frame]
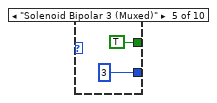
[diagram p19: hidden frame]
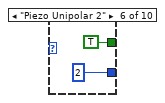
[diagram p20: hidden frame]
diagram:
  n1 = flat-sequence {
    tunnel: [w112] -> w2
    tunnel: [w101] -> w1
    tunnel: w2 -> [w122]
    tunnel: w1 -> [_]
    frame #0 {
      # "Wait for CPs to update"
      n2 = Wait (ms)(milliseconds to wait=u32 2000) -> ()  [unwired: 1 out]
    }
    frame #1 {
      # "Wait to run until opened"
      n3 = while {
        stop <- w5 stop-if-true
        n4 = property class="VI"() -> ("FP.State"=w6:T29)  [unwired: 2 in, 2 out]
        n5 = Not Equal?(x=w6, y=T29."Hidden" ("Front Panel Window:State")) -> (x != y?=w5:bool)
        n6 = Wait (ms)(milliseconds to wait=u32 100) -> ()  [unwired: 1 out]
      }
    }
    frame #2 {
      w14 = refnum<vi> refnum ("XYGraph in")
      # "Bank-Specific Items (also CTRL+F \"Bank A\" and \"DI-A\")"
      # "Miscellaneous Initialization"
      n7 = local read "_Ref Pump Current Profile FilePath"() -> (w54:path)
      n8 = local read "_Ref Inj FilePath"() -> (w20:path)
      n9 = control-ref of="_Phase Plot"() -> (w84:refnum<vi>)
      n10 = control-ref of="_Pump Phase Plot"() -> (w13:refnum<vi>)
      n11 = Read from Text File(file (use dialog)=w20) -> (text=w16:string)  [unwired: 3 in, 3 out]
      n12 = Type Cast(type=w14, x=w84) -> (*(type *) &x=w85:refnum<vi>)
      n13 = Type Cast(type=w14, x=w13) -> (*(type *) &x=w80:refnum<vi>)
      n14 = local read "RefInjTimeAxisMultiplier"() -> (w37:sgl)
      n15 = local read "ProfilesAdapt"() -> (w10:bool)
      n16 = local read "RefInjCurrentMultiplier"() -> (w38:sgl)
      n17 = local read "RefInjVoltageMultiplier"() -> (w40:sgl)
      n18 = local read "RefInjTimeAxisOffset"() -> (w36:sgl)
      n19 = local read "RefInjCurrentOffset"() -> (w39:sgl)
      n20 = local read "RefInjVoltageOffset"() -> (w41:sgl)
      n21 = Spreadsheet String To Array(delimiter (Tab)=",", format string="%s", spreadsheet string=w16) -> (array=w19:dbl[][])  [unwired: 1 in]
      n22 = Read from Text File(file (use dialog)=w54) -> (text=w58:string)  [unwired: 3 in, 3 out]
      n23 = local read "RefPumpTimeAxisMultiplier"() -> (w53:sgl)
      n24 = call "Plot Properties.vi"("LineTypes"="InjPhasePlotLineTypes", "LineWidths"="InjPhasePlotLineWidths", "PlotColors"="InjPhasePlotColors", "XYGraph in"=w85) -> ()  [unwired: 8 in]
      n25 = call "Plot Properties.vi"("LineTypes"="PumpPhasePlotLineTypes", "LineWidths"="PumpPhasePlotLineWidths", "PlotColors"="PumpPhasePlotColors", "XYGraph in"=w80) -> ()  [unwired: 8 in]
      n26 = local read "RefPumpCurrentMultiplier"() -> (w51:sgl)
      n27 = local read "RefPumpVoltageMultiplier"() -> (w49:sgl)
      n28 = local read "RefPumpTimeAxisOffset"() -> (w52:sgl)
      n29 = local read "RefPumpCurrentOffset"() -> (w50:sgl)
      n30 = local read "RefPumpVoltageOffset"() -> (w48:sgl)
      n31 = Transpose 2D Array(2D array=w19) -> (transposed array=w15:dbl[][])
      n32 = Spreadsheet String To Array(delimiter (Tab)=",", format string="%g", spreadsheet string=w58) -> (array=w55:dbl[][])  [unwired: 1 in]
      n33 = Index Array(array=w15) -> (element #1=w30:dbl[], element #2=w31:dbl[], element #3=w32:dbl[])  [unwired: 6 in]
      n34 = Transpose 2D Array(2D array=w55) -> (transposed array=w59:dbl[][])
      n35 = Select(t=T30."Disabled and Grayed Out" ("Disabled"), s=w10, f=T30."Enabled" ("Disabled")) -> (s? t:f=w9:T30)
      n36 = Index Array(array=w59) -> (element #1=w62:dbl[], element #2=w60:dbl[], element #3=w65:dbl[])  [unwired: 6 in]
      n37 = control-ref of="_Timing Plot"() -> (w76:refnum<vi>)
      n38 = control-ref of="_Pump Timing Plot"() -> (w69:refnum<vi>)
      n39 = Compound Arithmetic op=MULTIPLY(w37, w30) -> (w29:dbl[])
      n40 = Compound Arithmetic op=MULTIPLY(w38, w31) -> (w28:dbl[])
      n41 = Compound Arithmetic op=MULTIPLY(w40, w32) -> (w27:dbl[])
      n42 = property on="Profiles" class="Arr (strict)"("Array Element.DisabledEnum"=w9) -> ()  [unwired: 2 in, 2 out]
      n43 = Compound Arithmetic op=ADD(w36, w29) -> (w33:dbl[])
      n44 = Compound Arithmetic op=ADD(w28, w39) -> (w34:dbl[])
      n45 = Compound Arithmetic op=ADD(w27, w41) -> (w35:dbl[])
      n46 = Compound Arithmetic op=MULTIPLY(w53, w62) -> (w61:dbl[])
      n47 = Compound Arithmetic op=MULTIPLY(w51, w60) -> (w63:dbl[])
      n48 = Compound Arithmetic op=MULTIPLY(w49, w65) -> (w64:dbl[])
      n49 = call "Plot Properties.vi"("LineTypes"="InjCmdPlotLineTypes", "LineWidths"="InjCmdPlotLineWidths", "PlotColors"="InjCmdPlotColors", "XYGraph in"=w76) -> ()  [unwired: 8 in]
      n50 = call "Plot Properties.vi"("LineTypes"="PumpCmdPlotLineTypes", "LineWidths"="PumpCmdPlotLineWidths", "PlotColors"="PumpCmdPlotColors", "XYGraph in"=w69) -> ()  [unwired: 8 in]
      n51 = Compound Arithmetic op=ADD(w61, w52) -> (w66:dbl[])
      n52 = Compound Arithmetic op=ADD(w63, w50) -> (w42:dbl[])
      n53 = Compound Arithmetic op=ADD(w64, w48) -> (w43:dbl[])
      n54 = Bundle(w33, w34) -> (w21:cluster{dbl[], dbl[]})  [unwired: 1 in]
      n55 = Bundle(w33, w35) -> (w22:cluster{dbl[], dbl[]})  [unwired: 1 in]
      n56 = Empty Array?(array=w34) -> (empty?=w24:bool)
      n57 = Empty Array?(array=w35) -> (empty?=w25:bool)
      n58 = Empty Array?(array=w42) -> (empty?=w45:bool)
      n59 = Empty Array?(array=w43) -> (empty?=w46:bool)
      n60 = Bundle(w66, w42) -> (w67:cluster{dbl[], dbl[]})  [unwired: 1 in]
      n61 = Bundle(w66, w43) -> (w68:cluster{dbl[], dbl[]})  [unwired: 1 in]
      n62 = Build Array(w21, w22) -> (w23:cluster{dbl[], dbl[]}[])
      n63 = Compound Arithmetic op=OR(invert w24, invert w25) -> (w26:bool)
      n64 = Compound Arithmetic op=OR(invert w45, invert w46) -> (w44:bool)
      n65 = Build Array(w67, w68) -> (w47:cluster{dbl[], dbl[]}[])
      n66 = case shown="True" w26 {
        frame False {
          n67 = property on="_Phase Plot" class="XYGraph (strict)"("LegNumRows"=u32 8 ("Legend:Number of Rows")) -> ()  [unwired: 2 in, 2 out]
        }
        frame True {
          n68 = property on="_Phase Plot" class="XYGraph (strict)"("Active Plot"=u32 10, "Plot.Plot Name"="Ref I [A]", "Plot.YScaleIdx"=u32 1 ("Plot.Y Scale Index"), "Active Plot"=u32 11, "Plot.Plot Name"="Ref V [V]", "Plot.YScaleIdx"=u32 0 ("Plot.Y Scale Index"), "LegNumRows"=u32 12 ("Legend:Number of Rows")) -> ()  [unwired: 2 in, 2 out]
        }
      }
      n69 = local write "_Ref Inj Profiles"(w23) -> ()
      n70 = case shown="True" w44 {
        frame False {
          n71 = property on="_Pump Phase Plot" class="XYGraph (strict)"("Active Plot"=u32 6, "Plot.Plot Name"="Ref [A]", "LegNumRows"=u32 7 ("Legend:Number of Rows")) -> ()  [unwired: 2 in, 2 out]
        }
        frame True {
          n72 = property on="_Pump Phase Plot" class="XYGraph (strict)"("LegNumRows"=u32 6 ("Legend:Number of Rows")) -> ()  [unwired: 2 in, 2 out]
        }
      }
      n73 = local write "_Ref Pump Profiles"(w47) -> ()
      "_Bank A?" <- FALSE ("_Bank A?")
    }
    frame #3 {
      # "Refresh"
      n74 = control-ref of="ChanSelect1"() -> (w104:refnum<vi>)
      n75 = control-ref of="ChanSelect2"() -> (w105:refnum<vi>)
      n76 = control-ref of="ChanSelect3"() -> (w106:refnum<vi>)
      n77 = control-ref of="ChanSelect4"() -> (w107:refnum<vi>)
      n78 = control-ref of="This VI"() -> (w111:refnum<vi>)
      n79 = Build Array(w104, w105, w106, w107) -> (w103:refnum<vi>[])
      n80 = invoke class="VI" method="FP.Run-Time Position.Centered"(reference=w111) -> (reference out=w110:refnum<vi>, error out=w109:errorcluster)  [unwired: 4 in, 3 out]
      n81 = property on="_DI ADC Select" class="Enum (strict)"() -> ("Strings []"=w108:string[])  [unwired: 2 in, 2 out]
      n82 = property on="_DI Scope Event" class="Enum (strict)"() -> ("Strings []"=w98:string[])  [unwired: 2 in, 2 out]
      n83 = property on="_Refresh All" class="Bool (strict)"("Val(Sgnl)"=TRUE ("Value (Signaling)")) -> ()  [unwired: 2 in, 2 out]
      n84 = for {
        tunnel: w108 -> [w121] mode=indexing
        tunnel: [w119] -> w102 mode=indexing
        i -> [w120]
        n85 = Bundle(w121, w120) -> (w119:cluster{string, i32})  [unwired: 1 in]
      }
      n86 = for {
        tunnel: w98 -> [w115] mode=indexing
        tunnel: [w113] -> w99 mode=indexing
        i -> [w114]
        n87 = Bundle(w115, w114) -> (w113:cluster{string, i32})  [unwired: 1 in]
      }
      n88 = invoke class="VI" method="FP.Run-Time Pos.Unchanged"(reference=w110, error in=w109) -> (error out=w101:errorcluster)  [unwired: 1 in, 2 out]
      n89 = for {
        tunnel: w103 -> [w118] mode=indexing
        tunnel: w102 -> [w117]
        tunnel: [w116] -> w112 mode=indexing
        n90 = property on="Property Node" class="Ring (strict)"(reference=w118, "StringsAndValues[]"=w117) -> (reference out=w116:refnum<vi>)  [unwired: 1 in, 1 out]
      }
      n91 = property on="ScopeEvent" class="Ring (strict)"("StringsAndValues[]"=w99) -> ()  [unwired: 2 in, 2 out]
    }
    frame #4 {
      # "Code"
      n92 = while {
        tunnel: w122 -> [w123]
        stop <- FALSE stop-if-true
        n93 = event shown="[0] Timeout" {
          selector: _ -> [_ _ _ _ _ _ _ _ _ _ _ _ _ _ _ _ _ _ _ _ _ _ _ _ _ _ _ _ _ _ _ _ _ _ _ _ _ _ _ _ _ _ _ _ _ _ _ _]
          dyn-events: _ -> [_ _ _ _ _ _ _ _ _ _ _ _ _ _ _ _ _ _ _ _ _ _ _ _ _ _ _ _ _ _ _ _ _ _ _ _ _ _ _ _ _ _ _ _ _ _ _ _]
          timeout: 100 -> [_ _ _ _ _ _ _ _ _ _ _ _ _ _ _ _ _ _ _ _ _ _ _ _ _ _ _ _ _ _ _ _ _ _ _ _ _ _ _ _ _ _ _ _ _ _ _ _]
          tunnel: w123 -> [w176 _ _ _ _ _ _ _ _ _ _ _ _ _ _ _ _ _ _ _ _ _ _ _ _ _ _ _ _ _ _ _ _ _ _ _ _ _ _ _ _ _ _ _ _ _ _ _]
          event Timeout {
            n94 = event-data() -> ()  [unwired: 1 in, 1 out]
            n95 = for {
              tunnel: w176 -> [w235] mode=indexing
              tunnel: [w234] -> w177 mode=indexing
              tunnel: [w233] -> w175 mode=indexing
              n96 = property on="Property Node" class="Ring (strict)"(reference=w235) -> (reference out=w234:refnum<vi>, "Value"=w233:u8)  [unwired: 1 in, 1 out]
            }
            n97 = local read "State"() -> (w145:T19)
            n98 = local read "InjPhase"() -> (w140:T17)
            n99 = local read "PumpCapacitance"() -> (w156:sgl)
            n100 = local read "InjCmd"() -> (w139:T6)
            n101 = local read "PumpInductance"() -> (w163:sgl)
            n102 = local read "PumpResistance"() -> (w162:sgl)
            n103 = call "ChangeIndicator.vi"("Input"=w145) -> ("Change"=w135:bool)  [unwired: 9 in]
            n104 = local read "InjCapacitance"() -> (w161:sgl)
            n105 = First Call?() -> (First Call?: T/F=w133:bool)
            n106 = local read "InjInductance"() -> (w160:sgl)
            n107 = local read "SimRotations"() -> (w158:u8)
            n108 = local read "InjResistance"() -> (w159:sgl)
            n109 = local read "SimSpeed"() -> (w157:sgl)
            n110 = Compound Arithmetic op=OR(w133, w135) -> (w134:bool)
            n111 = local read "SimBatt"() -> (w155:sgl)
            n112 = call "ChangeIndicator.vi"("Input"=w140) -> ("Change"=w138:bool)  [unwired: 9 in]
            n113 = call "ChangeIndicator.vi"("Input"=w139) -> ("Change"=w137:bool)  [unwired: 9 in]
            n114 = case shown="True" w134 {
              tunnel: w145 -> [_ w220]
              frame False {
              }
              frame True {
                # "Bank A"
                n115 = Unbundle By Name(w220) -> ("System ADC.DRVP [V]"=w232:sgl, "System ADC.Primary B1B2 [V]"=w231:sgl, "System ADC.Primary B3B4 [V]"=w230:sgl, "System ADC.Secondary B1B2 [V]"=w229:sgl, "System ADC.Secondary B3B4 [V]"=w228:sgl, "System ADC.Ext HV B [V]"=w227:sgl, "System ADC.DI Zener B [V]"=w226:sgl, "System ADC.Pump Zener B [V]"=w225:sgl, "System ADC.Temp DI B [C]"=w223:sgl, "System ADC.Temp DI Zener B [C]"=w222:sgl, "System ADC.Temp Boost B [C]"=w221:sgl)
                n116 = local read "BoostClampV"() -> (w218:sgl)
                n117 = local write "_Temp DI"(w223) -> ()
                n118 = local write "_Temp DI Zener"(w222) -> ()
                n119 = local write "_Temp Boost Primary"(w221) -> ()
                n120 = Bundle("DRVP [V]"=w232, "Primary B1B2 [V]"=w231, "Primary B3B4 [V]"=w230, "Secondary B1B2 [V]"=w229, "Secondary B3B4 [V]"=w228, "Ext HV B [V]"=w227, "DI Zener B [V]"=w226, "Pump Zener B [V]"=w225, "BoostClampV"=w218) -> (w224:T35)  [unwired: 1 in]
                n121 = property on="_Redraw Slider" class="Bool (strict)"("Val(Sgnl)"=TRUE ("Value (Signaling)")) -> ()  [unwired: 2 in, 2 out]
                n122 = local write "_Bank B Status"(w224) -> ()
              }
            }
            n123 = Greater Than 0?(x="ScopeEvent") -> (x > 0?=w201:bool)
            n124 = local read "SYS|Exec|CalLoading"() -> (w143:bool)
            n125 = call "ChangeIndicator.vi"("Input"=w175) -> ("Change"=w174:bool)  [unwired: 9 in]
            n126 = Compound Arithmetic op=OR(w138, w137) -> (w136:bool)
            n127 = call "ChangeIndicator.vi"("Input"=w155) -> ("Change"=w164:bool)  [unwired: 9 in]
            n128 = call "ChangeIndicator.vi"("Input"=w157) -> ("Change"=w165:bool)  [unwired: 9 in]
            n129 = call "ChangeIndicator.vi"("Input"=w158) -> ("Change"=w166:bool)  [unwired: 9 in]
            n130 = call "ChangeIndicator.vi"("Input"=w159) -> ("Change"=w167:bool)  [unwired: 9 in]
            n131 = call "ChangeIndicator.vi"("Input"=w160) -> ("Change"=w168:bool)  [unwired: 9 in]
            n132 = call "ChangeIndicator.vi"("Input"=w161) -> ("Change"=w169:bool)  [unwired: 9 in]
            n133 = call "ChangeIndicator.vi"("Input"=w162) -> ("Change"=w170:bool)  [unwired: 9 in]
            n134 = call "ChangeIndicator.vi"("Input"=w163) -> ("Change"=w171:bool)  [unwired: 9 in]
            n135 = call "ChangeIndicator.vi"("Input"=w156) -> ("Change"=w172:bool)  [unwired: 9 in]
            n136 = Compound Arithmetic op=AND(w201, "ScopeEnable", w174) -> (w199:bool)
            n137 = case shown="True" w136 {
              frame False {
              }
              frame True {
                n138 = local read "_ChannelConfigurationList"() -> (w210:i32)
                n139 = local read "PhaseArraysList"() -> (w206:i32)
                n140 = local read "InjCmd"() -> (w209:T6)
                n141 = local read "Phase Array"() -> (w205:i32)
                n142 = local read "InjPhase"() -> (w211:T17)
                n143 = Index Array(array=w211, index (row)=w206, index (col)=w205) -> (element=w207:T13)
                n144 = Index Array(array=w209, index=w210) -> (element=w208:T7)
                n145 = local write "_Phase"(w207) -> ()
                n146 = local write "_InjCmd Element"(w208) -> ()
              }
            }
            n147 = case shown="True" w199 {
              tunnel: w177 -> [_ w264]
              frame False {
              }
              frame True {
                n148 = for {
                  tunnel: w264 -> [w265] mode=indexing
                  i -> [w268]
                  n149 = property on="Property Node" class="Ring (strict)"(reference=w265) -> ("StringsAndValues[]"=w271:T36, "Value"=w272:u8)  [unwired: 1 in, 2 out]
                  n150 = for {
                    tunnel: w271 -> [w282] mode=indexing
                    tunnel: [w279] -> w275
                    tunnel: w272 -> [w278]
                    stop <- w280 stop-if-true
                    n151 = Unbundle(w282) -> ("String"=w279:string, "Value"=w281:u8)
                    n152 = Equal?(x=w281, y=w278) -> (x = y?=w280:bool)
                  }
                  n153 = Match Pattern(string=w275, regular expression="I LS") -> (offset past match=w274:i32)  [unwired: 1 in, 3 out]
                  n154 = Greater Or Equal To 0?(x=w274) -> (x >= 0?=w269:bool)
                  n155 = Add(x=u32 6 ("Active Plot"), y=w268) -> (x+y=w266:u32)
                  n156 = Select(t=u32 1 ("Active Y Scale"), s=w269, f=u32 0 ("Active Y Scale")) -> (s? t:f=w277:u32)
                  n157 = property on="_Phase Plot" class="XYGraph (strict)"("Active Plot"=w266, "Plot.Plot Name"=w275, "Plot.YScaleIdx"=w277) -> ()  [unwired: 2 in, 2 out]
                }
              }
            }
            n158 = Compound Arithmetic op=OR(w164, w165, w166, w167, w168, w169, w170, w171, w172) -> (w173:bool)
            n159 = feedback-in #1(w143) -> ()
            n160 = feedback #1(FALSE ("SYS|Exec|CalLoading")) -> (w144:bool)
            n161 = case shown="True" w173 {
              frame False {
              }
              frame True {
                n162 = property on="_Redraw Phase Plot" class="Bool (strict)"("Val(Sgnl)"=TRUE ("Value (Signaling)")) -> ()  [unwired: 2 in, 2 out]
                n163 = property on="_Redraw Timing Plot" class="Bool (strict)"("Val(Sgnl)"=TRUE ("Value (Signaling)")) -> ()  [unwired: 2 in, 2 out]
                n164 = property on="_Redraw Pump Phase Plot" class="Bool (strict)"("Val(Sgnl)"=TRUE ("Value (Signaling)")) -> ()  [unwired: 2 in, 2 out]
                n165 = property on="_Redraw Pump Timing Plot" class="Bool (strict)"("Val(Sgnl)"=TRUE ("Value (Signaling)")) -> ()  [unwired: 2 in, 2 out]
              }
            }
            n166 = Compound Arithmetic op=AND(invert w143, w144) -> (w141:bool)
            n167 = case shown="True" w141 {
              frame False {
              }
              frame True {
                n168 = property on="_Refresh All" class="Bool (strict)"("Val(Sgnl)"=TRUE ("Value (Signaling)")) -> ()  [unwired: 2 in, 2 out]
              }
            }
            n169 = local read "PhaseArraysList"() -> (w183:i32)
            n170 = local read "PumpZenerEnable"() -> (w131:bool)
            n171 = local read "InjPhase"() -> (w184:T17)
            n172 = local read "Configuration"() -> (w151:u8)
            n173 = local read "BoostClampV"() -> (w147:sgl)
            n174 = local read "PumpPhase"() -> (w191:T12)
            n175 = local read "Data"() -> (w197:sgl[][])
            n176 = local read "PumpZenerV"() -> (w148:sgl)
            n177 = local read "ZenerEnable"() -> (w149:bool)
            n178 = local read "InjectEnable"() -> (w152:bool)
            n179 = local read "_SimuXY"() -> (w198:cluster{"Array":dbl[], "Array":dbl[]}[])
            n180 = local read "PSEnable"() -> (w153:bool)
            n181 = local read "BoostV"() -> (w150:sgl)
            n182 = local read "ZenerV"() -> (w146:sgl)
            n183 = Index Array(array=w184, index (row)=w183) -> (element=w182:T13[])  [unwired: 1 in]
            n184 = call "ChangeIndicator.vi"("Input"=w198) -> ("Change"=w195:bool)  [unwired: 9 in]
            n185 = call "ChangeIndicator.vi"("Input"=w197) -> ("Change"=w196:bool)  [unwired: 9 in]
            n186 = for {
              tunnel: [w241] -> w180 mode=indexing
              tunnel: w182 -> [w240] mode=indexing
              n187 = Unbundle By Name(w240) -> ("Current Control"=w241:T16)
            }
            n188 = for {
              tunnel: [w238] -> w189 mode=indexing
              tunnel: w191 -> [w237] mode=indexing
              n189 = Unbundle By Name(w237) -> ("Current Control"=w238:T16)
            }
            n190 = Bundle By Name(cluster=T31 {"Configuration"=enum."Solenoid Unipolar 4", "Power Supply Enable"=FALSE, "Boost Voltage [V]"=0.0, "Inject Enable"=FALSE, "Zener Enable"=FALSE, "Zener Voltage [V]"=0.0, "Pump Zener Enable"=FALSE, "Pump Zener Voltage [V]"=0.0, "Boost Clamp [V]"=0.0} ("_DI Bank_Configuration"), "Power Supply Enable"=w153, "Inject Enable"=w152, "Configuration"=w151, "Boost Voltage [V]"=w150, "Zener Enable"=w149, "Zener Voltage [V]"=w146, "Pump Zener Enable"=w131, "Pump Zener Voltage [V]"=w148, "Boost Clamp [V]"=w147) -> (w154:T31)
            n191 = Or(x=w195, y=w196) -> (x .or. y?=w194:bool)
            n192 = local read "Profiles"() -> (w181:sgl[][])
            n193 = case shown="True" w194 {
              tunnel: w198 -> [_ w257]
              tunnel: w197 -> [_ w256]
              frame False {
              }
              frame True {
                n194 = Index Array(array=w256) -> (element #1=w243:sgl[], element #2=w255:sgl[], element #3=w249:sgl[], element #4=w246:sgl[])  [unwired: 8 in]
                n195 = local read "dt"() -> (w242:sgl)
                n196 = Array Size(array=w243) -> (size(s)=w263:i32)
                n197 = Array Size(array=w255) -> (size(s)=w254:i32)
                n198 = Array Size(array=w249) -> (size(s)=w252:i32)
                n199 = Array Size(array=w246) -> (size(s)=w248:i32)
                n200 = call "DI Phase Plot Time Axis.vi"("dt"=w242, "Array Size"=w263) -> ("Array"=w262:dbl[])  [unwired: 9 in]
                n201 = call "DI Phase Plot Time Axis.vi"("dt"=w242, "Array Size"=w254) -> ("Array"=w253:dbl[])  [unwired: 9 in]
                n202 = call "DI Phase Plot Time Axis.vi"("dt"=w242, "Array Size"=w252) -> ("Array"=w250:dbl[])  [unwired: 9 in]
                n203 = call "DI Phase Plot Time Axis.vi"("dt"=w242, "Array Size"=w248) -> ("Array"=w247:dbl[])  [unwired: 9 in]
                n204 = Bundle("Array"=w262, "Data"=w243) -> (w258:cluster{"Array":dbl[], "Data":sgl[]})  [unwired: 1 in]
                n205 = Bundle("Array"=w253, "Data"=w255) -> (w251:cluster{"Array":dbl[], "Data":sgl[]})  [unwired: 1 in]
                n206 = Bundle("Array"=w250, "Data"=w249) -> (w245:cluster{"Array":dbl[], "Data":sgl[]})  [unwired: 1 in]
                n207 = Bundle("Array"=w247, "Data"=w246) -> (w244:cluster{"Array":dbl[], "Data":sgl[]})  [unwired: 1 in]
                n208 = Build Array(w258, w251, w245, w244) -> (w260:cluster{"Array":dbl[], "Data":sgl[]}[])
                n209 = Insert Into Array(array=w257, index=6, new element=w260) -> (→"_Phase Plot":cluster{"Array":dbl[], "Array":dbl[]}[])
              }
            }
            n210 = local read "RunState"() -> (w127:T1)
            n211 = Equal?(x=Control."Profile" ("Control"), y=w180) -> (x = y?=w179:bool[])
            n212 = Equal?(x=Control."Profile" ("Control"), y=w189) -> (x = y?=w190:bool[])
            n213 = call "ChangeIndicator.vi"("Input"=w181) -> ("Change"=w193:bool)  [unwired: 9 in]
            n214 = Or Array Elements(Boolean array=w179) -> (logical OR=w178:bool)
            n215 = Or Array Elements(Boolean array=w190) -> (logical OR=w192:bool)
            n216 = call "ChangeIndicator.vi"("Input"=w154) -> ("Change"=w126:bool)  [unwired: 9 in]
            n217 = Compound Arithmetic op=AND(w178, w193) -> (w186:bool)
            n218 = Compound Arithmetic op=AND(w193, w192) -> (w187:bool)
            n219 = call "ChangeIndicator.vi"("Input"=w127) -> ("Change"=w129:bool)  [unwired: 9 in]
            n220 = First Call?() -> (First Call?: T/F=w130:bool)
            n221 = case shown="True" w126 {
              tunnel: w154 -> [_ w213]
              frame False {
              }
              frame True {
                n222 = local write "_DI Bank_Configuration"(w213) -> ()
              }
            }
            n223 = case shown="True" w186 {
              frame False {
              }
              frame True {
                n224 = property on="_Redraw Phase Plot" class="Bool (strict)"("Val(Sgnl)"=TRUE ("Value (Signaling)")) -> ()  [unwired: 2 in, 2 out]
              }
            }
            n225 = case shown="True" w187 {
              frame False {
              }
              frame True {
                n226 = property on="_Redraw Pump Phase Plot" class="Bool (strict)"("Val(Sgnl)"=TRUE ("Value (Signaling)")) -> ()  [unwired: 2 in, 2 out]
              }
            }
            n227 = Compound Arithmetic op=OR(w130, w129) -> (w128:bool)
            n228 = case shown="True" w128 {
              tunnel: w127 -> [_ w204]
              frame False {
              }
              frame True {
                n229 = Add(x=w204, y=w204) -> (x+y=w203:u8)
                n230 = property on="Configuration" class="Enum (strict)"("DisabledEnum"=w203) -> ()  [unwired: 2 in, 2 out]
              }
            }
          }
          event "_Refresh All": Value Change {
            w308 = 16 ("dimension size")
            n231 = event-data() -> ()  [unwired: 1 in, 1 out]
            n232 = local write "_Refresh All"(FALSE ("_Refresh All")) -> ()
            n233 = flat-sequence {
              frame #0 {
                n234 = property on="_Redraw Phase" class="Bool (strict)"("Val(Sgnl)"=TRUE ("Value (Signaling)")) -> ()  [unwired: 2 in, 2 out]
                n235 = property on="_Redraw Phase Lists" class="Bool (strict)"("Val(Sgnl)"=TRUE ("Value (Signaling)")) -> ()  [unwired: 2 in, 2 out]
                n236 = property on="_Redraw Profiles Usage Tracker" class="Bool (strict)"("Val(Sgnl)"=TRUE ("Value (Signaling)")) -> ()  [unwired: 2 in, 2 out]
                n237 = property on="_Redraw DI Command" class="Bool (strict)"("Val(Sgnl)"=TRUE ("Value (Signaling)")) -> ()  [unwired: 2 in, 2 out]
                n238 = property on="_Redraw Injection List" class="Bool (strict)"("Val(Sgnl)"=TRUE ("Value (Signaling)")) -> ()  [unwired: 2 in, 2 out]
                n239 = property on="_Redraw Pump Phase List" class="Bool (strict)"("Val(Sgnl)"=TRUE ("Value (Signaling)")) -> ()  [unwired: 2 in, 2 out]
                n240 = property on="_Redraw Pump Phase" class="Bool (strict)"("Val(Sgnl)"=TRUE ("Value (Signaling)")) -> ()  [unwired: 2 in, 2 out]
                n241 = property on="_Redraw Pump Command" class="Bool (strict)"("Val(Sgnl)"=TRUE ("Value (Signaling)")) -> ()  [unwired: 2 in, 2 out]
                n242 = property on="_Redraw Profiles Usage Tracker" class="Bool (strict)"("Val(Sgnl)"=TRUE ("Value (Signaling)")) -> ()  [unwired: 2 in, 2 out]
                n243 = property on="_Redraw Slider" class="Bool (strict)"("Val(Sgnl)"=TRUE ("Value (Signaling)")) -> ()  [unwired: 2 in, 2 out]
              }
              frame #1 {
                n244 = property on="_Redraw Phase Plot" class="Bool (strict)"("Val(Sgnl)"=TRUE ("Value (Signaling)")) -> ()  [unwired: 2 in, 2 out]
                n245 = property on="_Redraw Timing Plot" class="Bool (strict)"("Val(Sgnl)"=TRUE ("Value (Signaling)")) -> ()  [unwired: 2 in, 2 out]
                n246 = property on="_Redraw Pump Phase Plot" class="Bool (strict)"("Val(Sgnl)"=TRUE ("Value (Signaling)")) -> ()  [unwired: 2 in, 2 out]
                n247 = property on="_Redraw Pump Timing Plot" class="Bool (strict)"("Val(Sgnl)"=TRUE ("Value (Signaling)")) -> ()  [unwired: 2 in, 2 out]
              }
            }
            n248 = local read "_ChannelConfigurationList"() -> (w307:i32)
            n249 = local read "InjCmd"() -> (w313:T6)
            n250 = local read "PumpPhase"() -> (w315:T12)
            n251 = local read "PumpCmd"() -> (w316:T26)
            n252 = local read "PhaseArraysList"() -> (w305:i32)
            n253 = local read "InjPhase"() -> (w314:T17)
            n254 = local read "Phase Array"() -> (w304:i32)
            n255 = for {
              tunnel: [w359] -> w312 mode=indexing
              tunnel: w313 -> [w358] mode=indexing
              n256 = call "Resize DI Command Array.vi"("Command in"=w358) -> ("Command out"=w359:T7)
            }
            n257 = call "Resize DI Command Array.vi"("Command in"=w316) -> ("Command out"=w317:T7)
            n258 = Reshape Array(w314, w308, w308) -> (w303:T17)
            n259 = Reshape Array(w315, 16 ("dimension size")) -> (w309:T12)
            n260 = local write "PumpCmd"(w317) -> ()
            n261 = local write "InjPhase"(w303) -> ()
            n262 = Index Array(array=w303, index (row)=w305, index (col)=w304) -> (element=w306:T13)
            n263 = Index Array(array=w312, index=w307) -> (element=w311:T7)
            n264 = local write "InjCmd"(w312) -> ()
            n265 = local write "PumpPhase"(w309) -> ()
            n266 = local write "_Phase"(w306) -> ()
            n267 = local write "_InjCmd Element"(w311) -> ()
            n268 = local read "PumpZenerEnable"() -> (w284:bool)
            n269 = local read "Configuration"() -> (w283:u8)
            n270 = local read "BoostClampV"() -> (w287:sgl)
            n271 = local read "PumpZenerV"() -> (w288:sgl)
            n272 = local read "ZenerEnable"() -> (w289:bool)
            n273 = local read "InjectEnable"() -> (w291:bool)
            n274 = local read "PSEnable"() -> (w292:bool)
            n275 = local read "BoostV"() -> (w290:sgl)
            n276 = local read "ZenerV"() -> (w286:sgl)
            n277 = local read "_ChannelConfigurationList"() -> (w297:i32)
            n278 = Bundle By Name(cluster=T31 {"Configuration"=enum."Solenoid Unipolar 4", "Power Supply Enable"=FALSE, "Boost Voltage [V]"=0.0, "Inject Enable"=FALSE, "Zener Enable"=FALSE, "Zener Voltage [V]"=0.0, "Pump Zener Enable"=FALSE, "Pump Zener Voltage [V]"=0.0, "Boost Clamp [V]"=0.0} ("_DI Bank_Configuration"), "Power Supply Enable"=w292, "Inject Enable"=w291, "Configuration"=w283, "Boost Voltage [V]"=w290, "Zener Enable"=w289, "Zener Voltage [V]"=w286, "Pump Zener Enable"=w284, "Pump Zener Voltage [V]"=w288, "Boost Clamp [V]"=w287) -> (w293:T31)
            n279 = Type Cast(type=DI_-_Bank_Configuration."Solenoid Unipolar 4" ("Configuration"), x=w283) -> (*(type *) &x=w295:T4)
            n280 = case shown="\"Piezo Unipolar 4 (Muxed)\"" w295 {
              tunnel: [4 8 7 2 3 2 4 3 2 3] -> w300
              tunnel: [TRUE ("Value (Signaling)") FALSE ("Value (Signaling)") TRUE ("Value (Signaling)") TRUE ("Value (Signaling)") TRUE ("Value (Signaling)") TRUE ("Value (Signaling)") FALSE ("Value (Signaling)") TRUE ("Value (Signaling)") TRUE ("Value (Signaling)") TRUE ("Value (Signaling)")] -> w294
              frame "Solenoid Unipolar 4" {
              }
              frame "Solenoid Unipolar 8 (Muxed)" {
              }
              frame "Solenoid Unipolar 7 (Muxed)" {
              }
              frame "Solenoid Bipolar 2" {
              }
              frame "Solenoid Bipolar 3 (Muxed)" {
              }
              frame "Piezo Unipolar 2" {
              }
              frame "Piezo Unipolar 4 (Muxed)" {
              }
              frame "Piezo Unipolar 3 (Muxed)" {
              }
              frame "Piezo Bipolar 2" {
              }
              frame "Piezo Bipolar 3 (Muxed)" {
              }
            }
            n281 = Decrement(x=w300) -> (x-1=w298:i32)
            n282 = local write "_DI Bank_Configuration"(w293) -> ()
            n283 = property on="_Tab Control" class="TabCtl (strict)"() -> ("Pages"=w301:refnum<vi>[])  [unwired: 2 in, 2 out]
            n284 = In Range and Coerce(upper limit=w298, x=w297, lower limit=0) -> (coerced(x)=w296:i32)  [unwired: 1 out]
            n285 = for {
              tunnel: w301 -> [w341] mode=indexing
              tunnel: w294 -> [w339]
              i -> [w340]
              n286 = case shown="1, 4" w340 {
                tunnel: w341 -> [_ w343]
                tunnel: w339 -> [_ w342]
                frame 0, Default {
                }
                frame 1, 4 {
                  n287 = property class="Page"(reference=w343, "PageVis"=w342) -> ()  [unwired: 1 in, 2 out]
                }
              }
            }
            n288 = local write "_ChannelConfigurationList"(w296) -> ()
          }
          event "PhaseArraysList": Value Change {
            n289 = event-data() -> ()  [unwired: 1 in, 1 out]
            n290 = local read "PhaseArraysList"() -> (w361:i32)
            n291 = local read "Phase Array"() -> (w360:i32)
            n292 = local read "InjPhase"() -> (w362:T17)
            n293 = property on="_Redraw Phase Lists" class="Bool (strict)"("Val(Sgnl)"=TRUE ("Value (Signaling)")) -> ()  [unwired: 2 in, 2 out]
            n294 = property on="_Redraw Phase Plot" class="Bool (strict)"("Val(Sgnl)"=TRUE ("Value (Signaling)")) -> ()  [unwired: 2 in, 2 out]
            n295 = property on="_Redraw Phase" class="Bool (strict)"("Val(Sgnl)"=TRUE ("Value (Signaling)")) -> ()  [unwired: 2 in, 2 out]
            n296 = Index Array(array=w362, index (row)=w361, index (col)=w360) -> (element=w363:T13)
            n297 = local write "_Phase"(w363) -> ()
          }
          event "_MovePhaseArrayListDown": Value Change {
            n298 = event-data() -> ()  [unwired: 1 in, 6 out]
            n299 = local read "PhaseArraysList"() -> (w374:i32)
            n300 = local read "InjPhase"() -> (w377:T17)
            n301 = property on="_Redraw Phase Lists" class="Bool (strict)"("Val(Sgnl)"=TRUE ("Value (Signaling)")) -> ()  [unwired: 2 in, 2 out]
            n302 = property on="_Redraw Phase Plot" class="Bool (strict)"("Val(Sgnl)"=TRUE ("Value (Signaling)")) -> ()  [unwired: 2 in, 2 out]
            n303 = property on="_Redraw Phase" class="Bool (strict)"("Val(Sgnl)"=TRUE ("Value (Signaling)")) -> ()  [unwired: 2 in, 2 out]
            n304 = Delete From Array(array=w377, index (row)=w374) -> (deleted portion=w375:T13[], array with subset deleted=w376:T17)  [unwired: 2 in]
            n305 = Increment(x=w374) -> (x+1=w369:i32)
            n306 = local write "_MovePhaseArrayListDown"(FALSE ("_MovePhaseArrayListDown")) -> ()
            n307 = In Range and Coerce(upper limit=15, x=w369, lower limit=0) -> (coerced(x)=w368:i32)  [unwired: 1 out]
            n308 = local write "PhaseArraysList"(w368) -> ()
            n309 = local read "Phase Array"() -> (w373:i32)
            n310 = Insert Into Array(array=w376, index (row)=w368, new element=w375) -> (w367:T17)  [unwired: 1 in]
            n311 = local write "InjPhase"(w367) -> ()
            n312 = Index Array(array=w367, index (row)=w368, index (col)=w373) -> (element=w372:T13)
            n313 = local write "_Phase"(w372) -> ()
          }
          event "_MovePhaseArrayListUp": Value Change {
            n314 = event-data() -> ()  [unwired: 1 in, 6 out]
            n315 = local read "PhaseArraysList"() -> (w390:i32)
            n316 = local read "InjPhase"() -> (w393:T17)
            n317 = property on="_Redraw Phase Lists" class="Bool (strict)"("Val(Sgnl)"=TRUE ("Value (Signaling)")) -> ()  [unwired: 2 in, 2 out]
            n318 = property on="_Redraw Phase Plot" class="Bool (strict)"("Val(Sgnl)"=TRUE ("Value (Signaling)")) -> ()  [unwired: 2 in, 2 out]
            n319 = property on="_Redraw Phase" class="Bool (strict)"("Val(Sgnl)"=TRUE ("Value (Signaling)")) -> ()  [unwired: 2 in, 2 out]
            n320 = Delete From Array(array=w393, index (row)=w390) -> (deleted portion=w391:T13[], array with subset deleted=w392:T17)  [unwired: 2 in]
            n321 = Decrement(x=w390) -> (x-1=w385:i32)
            n322 = In Range and Coerce(upper limit=15, x=w385, lower limit=0) -> (coerced(x)=w384:i32)  [unwired: 1 out]
            n323 = local write "_MovePhaseArrayListUp"(FALSE ("_MovePhaseArrayListUp")) -> ()
            n324 = local write "PhaseArraysList"(w384) -> ()
            n325 = local read "Phase Array"() -> (w389:i32)
            n326 = Insert Into Array(array=w392, index (row)=w384, new element=w391) -> (w382:T17)  [unwired: 1 in]
            n327 = local write "InjPhase"(w382) -> ()
            n328 = Index Array(array=w382, index (row)=w384, index (col)=w389) -> (element=w388:T13)
            n329 = local write "_Phase"(w388) -> ()
          }
          event "Phase Array": Value Change {
            n330 = event-data() -> ()  [unwired: 1 in, 1 out]
            n331 = local read "PhaseArraysList"() -> (w398:i32)
            n332 = local read "Phase Array"() -> (w397:i32)
            n333 = local read "InjPhase"() -> (w399:T17)
            n334 = property on="_Redraw Phase" class="Bool (strict)"("Val(Sgnl)"=TRUE ("Value (Signaling)")) -> ()  [unwired: 2 in, 2 out]
            n335 = Index Array(array=w399, index (row)=w398, index (col)=w397) -> (element=w400:T13)
            n336 = local write "_Phase"(w400) -> ()
          }
          event Value Change {
            # "(Except Configuration)"
            n337 = event-data() -> ()  [unwired: 1 in, 6 out]
            n338 = local read "State"() -> (w403:T19)
            n339 = Unbundle By Name(w403) -> ("System ADC.Battery [V]"=w412:sgl, "System ADC.DRVP [V]"=w413:sgl, "System ADC.Ext HV A [V]"=w414:sgl, "System ADC.Ext HV B [V]"=w415:sgl)
            n340 = Unbundle By Name("_DI Bank_Configuration") -> ("Power Supply Enable"=w425:bool, "Inject Enable"=w424:bool, "Boost Voltage [V]"=w405:sgl, "DI Zener Enable"=w423:bool, "DI Zener Voltage [V]"=w421:sgl, "Pump Zener Enable"=w417:bool, "Pump Zener Voltage [V]"=w418:sgl, "Boost Clamp [V]"=w410:sgl)
            n341 = local read "_Bank A?"() -> (w407:bool)
            n342 = Select(t=w414, s=w407, f=w415) -> (s? t:f=w406:sgl)
            n343 = Build Array(w405, w412, w413, w406) -> (w411:sgl[])
            n344 = property on="PSEnable" class="Bool (strict)"("Val(Sgnl)"=w425) -> ()  [unwired: 2 in, 2 out]
            n345 = property on="InjectEnable" class="Bool (strict)"("Val(Sgnl)"=w424) -> ()  [unwired: 2 in, 2 out]
            n346 = property on="BoostV" class="DigNum (strict)"("Val(Sgnl)"=w405) -> ()  [unwired: 2 in, 2 out]
            n347 = property on="ZenerEnable" class="Bool (strict)"("Val(Sgnl)"=w423) -> ()  [unwired: 2 in, 2 out]
            n348 = property on="ZenerV" class="DigNum (strict)"("Val(Sgnl)"=w421) -> ()  [unwired: 2 in, 2 out]
            n349 = property on="PumpZenerEnable" class="Bool (strict)"("Val(Sgnl)"=w417) -> ()  [unwired: 2 in, 2 out]
            n350 = property on="PumpZenerV" class="DigNum (strict)"("Val(Sgnl)"=w418) -> ()  [unwired: 2 in, 2 out]
            n351 = Array Max & Min(array=w411) -> (max value=w404:sgl)  [unwired: 3 out]
            n352 = Add(x=5.0 ("y"), y=w404) -> (x+y=w408:dbl)
            n353 = Max & Min(x=w410, y=w408) -> (max(x,y)=w402:dbl)  [unwired: 1 out]
            n354 = property on="BoostClampV" class="DigNum (strict)"("Val(Sgnl)"=w402) -> ()  [unwired: 2 in, 2 out]
            n355 = property on="Boost Clamp [V]" class="DigNum (strict)"("Value"=w402) -> ()  [unwired: 2 in, 2 out]
            n356 = property on="_Redraw Slider" class="Bool (strict)"("Val(Sgnl)"=TRUE ("Value (Signaling)")) -> ()  [unwired: 2 in, 2 out]
            n357 = property on="_Redraw Phase Plot" class="Bool (strict)"("Val(Sgnl)"=TRUE ("Value (Signaling)")) -> ()  [unwired: 2 in, 2 out]
            n358 = property on="_Redraw Pump Phase Plot" class="Bool (strict)"("Val(Sgnl)"=TRUE ("Value (Signaling)")) -> ()  [unwired: 2 in, 2 out]
          }
          event Value Change {
            n359 = event-data() -> ("NewVal"=w426:T4)  [unwired: 1 in, 5 out]
            n360 = local read "_ChannelConfigurationList"() -> (w429:i32)
            n361 = case shown="\"Piezo Unipolar 3 (Muxed)\"" w426 {
              tunnel: [4 8 7 2 3 2 4 3 2 3] -> w432
              tunnel: [TRUE ("Value (Signaling)") FALSE ("Value (Signaling)") TRUE ("Value (Signaling)") TRUE ("Value (Signaling)") TRUE ("Value (Signaling)") TRUE ("Value (Signaling)") FALSE ("Value (Signaling)") TRUE ("Value (Signaling)") TRUE ("Value (Signaling)") TRUE ("Value (Signaling)")] -> w427
              frame "Solenoid Unipolar 4" {
              }
              frame "Solenoid Unipolar 8 (Muxed)" {
              }
              frame "Solenoid Unipolar 7 (Muxed)" {
              }
              frame "Solenoid Bipolar 2" {
              }
              frame "Solenoid Bipolar 3 (Muxed)" {
              }
              frame "Piezo Unipolar 2" {
              }
              frame "Piezo Unipolar 4 (Muxed)" {
              }
              frame "Piezo Unipolar 3 (Muxed)" {
              }
              frame "Piezo Bipolar 2" {
              }
              frame "Piezo Bipolar 3 (Muxed)" {
              }
            }
            n362 = local write "_Bank Wiring Diagram"(w426) -> ()
            n363 = property on="Configuration" class="DigNum (strict)"("Val(Sgnl)"=w426) -> ()  [unwired: 2 in, 2 out]
            n364 = Decrement(x=w432) -> (x-1=w430:i32)
            n365 = property on="_Tab Control" class="TabCtl (strict)"() -> ("Pages"=w433:refnum<vi>[])  [unwired: 2 in, 2 out]
            n366 = In Range and Coerce(upper limit=w430, x=w429, lower limit=0) -> (coerced(x)=w428:i32)  [unwired: 1 out]
            n367 = for {
              tunnel: w433 -> [w464] mode=indexing
              tunnel: w427 -> [w462]
              i -> [w463]
              n368 = case shown="1, 4" w463 {
                tunnel: w464 -> [_ w466]
                tunnel: w462 -> [_ w465]
                frame 0, Default {
                }
                frame 1, 4 {
                  n369 = property class="Page"(reference=w466, "PageVis"=w465) -> ()  [unwired: 1 in, 2 out]
                }
              }
            }
            n370 = local write "_ChannelConfigurationList"(w428) -> ()
            n371 = property on="_Redraw Phase Lists" class="Bool (strict)"("Val(Sgnl)"=TRUE ("Value (Signaling)")) -> ()  [unwired: 2 in, 2 out]
            n372 = property on="_Redraw Phase Plot" class="Bool (strict)"("Val(Sgnl)"=TRUE ("Value (Signaling)")) -> ()  [unwired: 2 in, 2 out]
            n373 = property on="_Redraw Phase" class="Bool (strict)"("Val(Sgnl)"=TRUE ("Value (Signaling)")) -> ()  [unwired: 2 in, 2 out]
            n374 = property on="_Redraw Injection List" class="Bool (strict)"("Val(Sgnl)"=TRUE ("Value (Signaling)")) -> ()  [unwired: 2 in, 2 out]
            n375 = property on="_Redraw Timing Plot" class="Bool (strict)"("Val(Sgnl)"=TRUE ("Value (Signaling)")) -> ()  [unwired: 2 in, 2 out]
            n376 = property on="_Redraw Pump Phase Plot" class="Bool (strict)"("Val(Sgnl)"=TRUE ("Value (Signaling)")) -> ()  [unwired: 2 in, 2 out]
            n377 = property on="_Redraw Pump Phase List" class="Bool (strict)"("Val(Sgnl)"=TRUE ("Value (Signaling)")) -> ()  [unwired: 2 in, 2 out]
            n378 = property on="_Redraw Pump Phase" class="Bool (strict)"("Val(Sgnl)"=TRUE ("Value (Signaling)")) -> ()  [unwired: 2 in, 2 out]
          }
          event "SimInjDuration": Value Change {
            n379 = event-data() -> ()  [unwired: 1 in, 1 out]
            n380 = property on="_Redraw Phase Plot" class="Bool (strict)"("Val(Sgnl)"=TRUE ("Value (Signaling)")) -> ()  [unwired: 2 in, 2 out]
          }
          event Value Change {
            n381 = event-data() -> ()  [unwired: 1 in, 1 out]
            n382 = property on="_Redraw Phase Lists" class="Bool (strict)"("Val(Sgnl)"=TRUE ("Value (Signaling)")) -> ()  [unwired: 2 in, 2 out]
            n383 = property on="_Redraw Phase Plot" class="Bool (strict)"("Val(Sgnl)"=TRUE ("Value (Signaling)")) -> ()  [unwired: 2 in, 2 out]
            n384 = property on="_Redraw Phase" class="Bool (strict)"("Val(Sgnl)"=TRUE ("Value (Signaling)")) -> ()  [unwired: 2 in, 2 out]
            n385 = property on="_Redraw Profiles Usage Tracker" class="Bool (strict)"("Val(Sgnl)"=TRUE ("Value (Signaling)")) -> ()  [unwired: 2 in, 2 out]
            n386 = local read "PhaseArraysList"() -> (w475:i32)
            n387 = local read "Phase Array"() -> (w474:i32)
            n388 = local read "InjPhase"() -> (w476:T17)
            n389 = local read "_Phase"() -> (w473:T13)
            n390 = Replace Array Subset(array=w476, new element=w473, index (row)=w475, index (col)=w474) -> (w468:T17)
            n391 = local write "InjPhase"(w468) -> ()
          }
          event "_Remove Phase": Value Change {
            n392 = event-data() -> ()  [unwired: 1 in, 1 out]
            n393 = local write "_Remove Phase"(FALSE ("Remove Phase")) -> ()
            n394 = local read "PhaseArraysList"() -> (w487:i32)
            n395 = local read "Phase Array"() -> (w480:i32)
            n396 = local read "InjPhase"() -> (w486:T17)
            n397 = Index Array(array=w486, index (row)=w487) -> (element=w488:T13[])  [unwired: 1 in]
            n398 = property on="_Redraw Phase Lists" class="Bool (strict)"("Val(Sgnl)"=TRUE ("Value (Signaling)")) -> ()  [unwired: 2 in, 2 out]
            n399 = property on="_Redraw Phase Plot" class="Bool (strict)"("Val(Sgnl)"=TRUE ("Value (Signaling)")) -> ()  [unwired: 2 in, 2 out]
            n400 = property on="_Redraw Phase" class="Bool (strict)"("Val(Sgnl)"=TRUE ("Value (Signaling)")) -> ()  [unwired: 2 in, 2 out]
            n401 = property on="_Redraw Profiles Usage Tracker" class="Bool (strict)"("Val(Sgnl)"=TRUE ("Value (Signaling)")) -> ()  [unwired: 2 in, 2 out]
            n402 = Array Size(array=w488) -> (size(s)=w490:i32)
            n403 = Delete From Array(array=w488, index=w480) -> (array with subset deleted=w489:T13[])  [unwired: 1 in, 1 out]
            n404 = Reshape Array(w489, w490) -> (w481:T13[])
            n405 = Replace Array Subset(array=w486, new element=w481, index (row)=w487) -> (w477:T17)  [unwired: 1 in]
            n406 = Index Array(array=w481, index=w480) -> (element=w479:T13)
            n407 = local write "InjPhase"(w477) -> ()
            n408 = local write "_Phase"(w479) -> ()
          }
          event "_Insert Phase": Value Change {
            n409 = event-data() -> ()  [unwired: 1 in, 1 out]
            n410 = local write "_Insert Phase"(FALSE ("Remove Phase")) -> ()
            n411 = local read "PhaseArraysList"() -> (w503:i32)
            n412 = local read "Phase Array"() -> (w494:i32)
            n413 = local read "InjPhase"() -> (w502:T17)
            n414 = Index Array(array=w502, index (row)=w503) -> (element=w496:T13[])  [unwired: 1 in]
            n415 = property on="_Redraw Phase Lists" class="Bool (strict)"("Val(Sgnl)"=TRUE ("Value (Signaling)")) -> ()  [unwired: 2 in, 2 out]
            n416 = property on="_Redraw Phase Plot" class="Bool (strict)"("Val(Sgnl)"=TRUE ("Value (Signaling)")) -> ()  [unwired: 2 in, 2 out]
            n417 = property on="_Redraw Phase" class="Bool (strict)"("Val(Sgnl)"=TRUE ("Value (Signaling)")) -> ()  [unwired: 2 in, 2 out]
            n418 = property on="_Redraw Profiles Usage Tracker" class="Bool (strict)"("Val(Sgnl)"=TRUE ("Value (Signaling)")) -> ()  [unwired: 2 in, 2 out]
            n419 = Array Size(array=w496) -> (size(s)=w504:i32)
            n420 = Index Array(array=w496, index=w494) -> (element=w495:T13)
            n421 = Insert Into Array(array=w496, index=w494, new element=w495) -> (w493:T13[])
            n422 = Reshape Array(w493, w504) -> (w497:T13[])
            n423 = Replace Array Subset(array=w502, new element=w497, index (row)=w503) -> (w491:T17)  [unwired: 1 in]
            n424 = local write "InjPhase"(w491) -> ()
          }
          event "_Redraw Phase Lists": Value Change {
            n425 = event-data() -> ()  [unwired: 1 in, 1 out]
            n426 = local write "_Redraw Phase Lists"(FALSE ("Redraw Phase Lists")) -> ()
            n427 = local read "PhaseArraysList"() -> (w515:i32)
            n428 = local read "Phase Array"() -> (w510:i32)
            n429 = property on="Configuration" class="Enum (strict)"() -> ("Value"=w505:T4)  [unwired: 2 in, 2 out]
            n430 = Bundle By Name(cluster=T32 {"Configuration"=enum."Solenoid Unipolar 4", "Boost Voltage [V]"=0.0, "Zener Enable"=FALSE, "Zener Voltage [V]"=0.0} ("Configuration"), "Configuration"=w505) -> (w508:T32)
            n431 = local read "InjPhase"() -> (w506:T17)
            n432 = control-ref of="PhaseArraysList"() -> (w521:refnum<vi>)
            n433 = control-ref of="Phase Array"() -> (w520:refnum<vi>)
            n434 = In Range and Coerce(upper limit=15, x=w515, lower limit=0) -> (coerced(x)=w516:i32, In Range?=w517:bool)
            n435 = In Range and Coerce(upper limit=15, x=w510, lower limit=0) -> (coerced(x)=w509:i32, In Range?=w518:bool)
            n436 = case shown="False" w517 {
              tunnel: w516 -> [w523 _]
              frame False {
                n437 = property on="PhaseArraysList" class="LstBox (strict)"("Val(Sgnl)"=w523) -> ()  [unwired: 2 in, 2 out]
              }
              frame True {
              }
            }
            n438 = case shown="False" w518 {
              tunnel: w509 -> [w522 _]
              frame False {
                n439 = property on="Phase Array" class="LstBox (strict)"("Val(Sgnl)"=w522) -> ()  [unwired: 2 in, 2 out]
              }
              frame True {
              }
            }
            n440 = property on="InjPhase" class="Arr (strict)"("Val(Sgnl)"=w506) -> ()  [unwired: 2 in, 2 out]
            n441 = call <vilib>:"Phase Listbox.vi"(8:"Phase Arrays"=w506, "Configuration"=w508, "Phase Array"=w520, 11:"Phase Arrays"=w521) -> ()  [unwired: 7 in, 1 out]
          }
          event "_Redraw Phase Plot": Value Change {
            n442 = event-data() -> ()  [unwired: 1 in, 1 out]
            n443 = local read "_DI Bank_Configuration"() -> (w554:T3)
            n444 = local read "InjCapacitance"() -> (w524:sgl)
            n445 = local read "InjInductance"() -> (w525:sgl)
            n446 = local read "InjResistance"() -> (w526:sgl)
            n447 = Bundle By Name(cluster=T33 {"Resistance [Ohm]"=1.0, "Inductance [Henery]"=0.001, "Capacitance [Farad]"=5e-06} ("Injector Configuration"), "Resistance [Ohm]"=w526, "Inductance [Henery]"=w525, "Capacitance [Farad]"=w524) -> (w528:T33)
            n448 = local read "SimBatt"() -> (w527:sgl)
            n449 = Unbundle By Name(w554) -> ("Configuration"=w553:T4, "Boost Voltage [V]"=w552:sgl, "DI Zener Enable"=w551:bool, "DI Zener Voltage [V]"=w550:sgl)
            n450 = local read "_Ref Inj Profiles"() -> (w541:cluster{"Array":dbl[], "Array":dbl[]}[])
            n451 = local read "PhaseArraysList"() -> (w560:i32)
            n452 = local read "InjPhase"() -> (w561:T17)
            n453 = Bundle By Name(cluster=T34 {"Battery [V]"=13.7, "Engine Speed [RPM]"=0.0, "Rotations"=0, "Injector Configuration"={"Resistance [Ohm]"=1.0, "Inductance [Henery]"=0.001, "Capacitance [Farad]"=5e-06}, "Description"=""} ("System"), "Battery [V]"=w527, "Injector Configuration"=w528) -> (w557:T34)
            n454 = local read "Profiles"() -> (w530:sgl[][])
            n455 = Bundle By Name(cluster=T32 {"Configuration"=enum."Solenoid Unipolar 4", "Boost Voltage [V]"=0.0, "Zener Enable"=FALSE, "Zener Voltage [V]"=0.0} ("Configuration"), "Configuration"=w553, "Boost Voltage [V]"=w552, "Zener Enable"=w551, "Zener Voltage [V]"=w550) -> (w555:T32)
            n456 = Index Array(array=w541) -> (element #1=w540:cluster{"Array":dbl[], "Array":dbl[]}, element #2=w539:cluster{"Array":dbl[], "Array":dbl[]})  [unwired: 2 in]
            n457 = Unbundle(w540) -> ("Array"=w549:dbl[], "Array"=w548:dbl[])
            n458 = Unbundle(w539) -> ("Array"=w538:dbl[], "Array"=w532:dbl[])
            n459 = Index Array(array=w561, index (row)=w560) -> (element=w562:T13[])  [unwired: 1 in]
            n460 = local write "_Redraw Phase Plot"(FALSE ("Redraw Phase Plot")) -> ()
            n461 = call <vilib>:"Phase Plot.vi"("Phase Arrays"=w562, "Profiles - Pulse Width [s]"=w530, "System"=w557, "Configuration"=w555, "Duration (1m) [s]"="SimInjDuration") -> ("Plot"=w543:cluster{"Array":sgl[], "Array":sgl[]}[])  [unwired: 13 in, 1 out]
            n462 = for {
              tunnel: w549 -> [w568] mode=indexing
              tunnel: [w568] -> w547 mode=indexing if=w566
              tunnel: [w567] -> w546 mode=indexing if=w566
              tunnel: w548 -> [w567] mode=indexing
              n463 = Greater Or Equal To 0?(x=w568) -> (x >= 0?=w566:bool)
            }
            n464 = for {
              tunnel: w538 -> [w565] mode=indexing
              tunnel: [w565] -> w537 mode=indexing if=w563
              tunnel: [w564] -> w536 mode=indexing if=w563
              tunnel: w532 -> [w564] mode=indexing
              n465 = Greater Or Equal To 0?(x=w565) -> (x >= 0?=w563:bool)
            }
            n466 = Empty Array?(array=w548) -> (empty?=w535:bool)
            n467 = Empty Array?(array=w532) -> (empty?=w534:bool)
            n468 = Compound Arithmetic op=OR(invert w535, invert w534) -> (w533:bool)
            n469 = Bundle(w547, w546) -> (w545:cluster{dbl[], dbl[]})  [unwired: 1 in]
            n470 = Bundle(w537, w536) -> (w531:cluster{dbl[], dbl[]})  [unwired: 1 in]
            n471 = case shown="True" w533 {
              tunnel: w543 -> [w570 w581]
              tunnel: [w570 w580] -> w542
              tunnel: w545 -> [_ w579]
              tunnel: w531 -> [_ w578]
              frame False {
                n472 = property on="_Phase Plot" class="XYGraph (strict)"("LegNumRows"=u32 10 ("Legend:Number of Rows")) -> ()  [unwired: 2 in, 2 out]
              }
              frame True {
                n473 = Build Array (concatenate)(w581, w579, w578) -> (w580:cluster{"Array":dbl[], "Array":dbl[]}[])
                n474 = property on="_Phase Plot" class="XYGraph (strict)"("Active Plot"=u32 10, "Plot.Plot Name"="Ref I [A]", "Plot.YScaleIdx"=u32 1 ("Plot.Y Scale Index"), "Active Plot"=u32 11, "Plot.Plot Name"="Ref V [V]", "Plot.YScaleIdx"=u32 0 ("Plot.Y Scale Index"), "LegNumRows"=u32 12 ("Legend:Number of Rows")) -> ()  [unwired: 2 in, 2 out]
              }
            }
            "_SimuXY" <- w542
          }
          event "_Redraw Phase": Value Change {
            n475 = event-data() -> ()  [unwired: 1 in, 1 out]
            n476 = local write "_Redraw Phase"(FALSE ("Redraw Phase")) -> ()
            n477 = property on="Configuration" class="Enum (strict)"() -> ("Value"=w582:T4)  [unwired: 2 in, 2 out]
            n478 = Bundle By Name(cluster=T32 {"Configuration"=enum."Solenoid Unipolar 4", "Boost Voltage [V]"=0.0, "Zener Enable"=FALSE, "Zener Voltage [V]"=0.0} ("Configuration"), "Configuration"=w582) -> (w585:T32)
            n479 = control-ref of="_Phase"() -> (w583:refnum<vi>)
            n480 = call <vilib>:"Disable Phase Array.vi"("Configuration"=w585, "Phase Ref"=w583) -> ()  [unwired: 10 in]
          }
          event "ProfilesAdapt": Value Change {
            n481 = event-data() -> ("NewVal"=w589:bool)  [unwired: 1 in]
            n482 = Select(t=T30."Disabled and Grayed Out" ("Disabled"), s=w589, f=T30."Enabled" ("Disabled")) -> (s? t:f=w587:T30)
            n483 = property on="Profiles" class="Arr (strict)"("Array Element.DisabledEnum"=w587) -> ()  [unwired: 2 in, 2 out]
          }
          event "_Redraw Profiles Usage Tracker": Value Change {
            n484 = event-data() -> ()  [unwired: 1 in, 6 out]
            n485 = local write "_Redraw Profiles Usage Tracker"(FALSE ("_Redraw Profiles Usage Tracker")) -> ()
            n486 = local read "InjPhase"() -> (w591:T17)
            n487 = control-ref of="_Profiles usage tracker"() -> (w593:refnum<vi>)
            n488 = call "Format Phase Profiles Tracker.vi"("InjPhase"=w591, "Listbox Ref"=w593) -> ()  [unwired: 10 in]
          }
          event "_Ref Inj FilePath": Value Change {
            n489 = event-data() -> ()  [unwired: 1 in, 6 out]
            n490 = Read from Text File(file (use dialog)="_Ref Inj FilePath") -> (text=w615:string)  [unwired: 3 in, 3 out]
            n491 = Spreadsheet String To Array(delimiter (Tab)=",", format string="%s", spreadsheet string=w615) -> (array=w618:dbl[][])  [unwired: 1 in]
            n492 = Transpose 2D Array(2D array=w618) -> (transposed array=w612:dbl[][])
            n493 = Index Array(array=w612) -> (element #1=w605:dbl[], element #2=w601:dbl[], element #3=w598:dbl[])  [unwired: 6 in]
            n494 = property on="_Redraw Phase Plot" class="Bool (strict)"("Val(Sgnl)"=TRUE ("Value (Signaling)")) -> ()  [unwired: 2 in, 2 out]
            n495 = Compound Arithmetic op=MULTIPLY("RefInjTimeAxisMultiplier", w605) -> (w608:dbl[])
            n496 = Compound Arithmetic op=MULTIPLY("RefInjCurrentMultiplier", w601) -> (w607:dbl[])
            n497 = Compound Arithmetic op=MULTIPLY("RefInjVoltageMultiplier", w598) -> (w606:dbl[])
            n498 = Compound Arithmetic op=ADD("RefInjTimeAxisOffset", w608) -> (w596:dbl[])
            n499 = Compound Arithmetic op=ADD(w607, "RefInjCurrentOffset") -> (w595:dbl[])
            n500 = Compound Arithmetic op=ADD(w606, "RefInjVoltageOffset") -> (w594:dbl[])
            n501 = Bundle(w596, w595) -> (w611:cluster{dbl[], dbl[]})  [unwired: 1 in]
            n502 = Bundle(w596, w594) -> (w609:cluster{dbl[], dbl[]})  [unwired: 1 in]
            n503 = Build Array(w611, w609) -> (→"_Ref Inj Profiles":cluster{dbl[], dbl[]}[])
          }
          event "_Save Profile": Value Change {
            n504 = event-data() -> ()  [unwired: 1 in, 1 out]
            n505 = local read "PhaseArraysList"() -> (w621:i32)
            n506 = local read "InjPhase"() -> (w620:T17)
            n507 = Index Array(array=w620, index (row)=w621) -> (element=w619:T13[])  [unwired: 1 in]
            n508 = call <vilib>:"Save Phase Array.vi"("Phase Array"=w619) -> ()  [unwired: 11 in]
          }
          event "_Apply Profile": Value Change {
            n509 = event-data() -> ()  [unwired: 1 in, 6 out]
            n510 = local read "PhaseArraysList"() -> (w624:i32)
            n511 = local read "InjPhase"() -> (w625:T17)
            n512 = call <vilib>:"Load Phase Array.vi"() -> ("error out"=w622:errorcluster, "Phase Array"=w623:T13[])  [unwired: 10 in]
            n513 = case shown="No Error" w622 {
              selector: w622 -> [_ w634]
              tunnel: w623 -> [w633 _]
              tunnel: w625 -> [w632 _]
              tunnel: w624 -> [w631 _]
              frame No Error {
                n514 = Replace Array Subset(array=w632, new element=w633, index (row)=w631) -> (w626:T17)  [unwired: 1 in]
                n515 = property on="_Redraw Phase Lists" class="Bool (strict)"("Val(Sgnl)"=TRUE ("Value (Signaling)")) -> ()  [unwired: 2 in, 2 out]
                n516 = property on="_Redraw Phase Plot" class="Bool (strict)"("Val(Sgnl)"=TRUE ("Value (Signaling)")) -> ()  [unwired: 2 in, 2 out]
                n517 = property on="_Redraw Phase" class="Bool (strict)"("Val(Sgnl)"=TRUE ("Value (Signaling)")) -> ()  [unwired: 2 in, 2 out]
                n518 = property on="_Redraw Profiles Usage Tracker" class="Bool (strict)"("Val(Sgnl)"=TRUE ("Value (Signaling)")) -> ()  [unwired: 2 in, 2 out]
                n519 = local write "InjPhase"(w626) -> ()
              }
              frame Error {
                n520 = call <vilib>:"Simple Error Handler.vi"("error in (no error)"=w634) -> ()  [unwired: 4 in, 5 out]
              }
            }
          }
          event "_ChannelConfigurationList": Value Change {
            n521 = event-data() -> ()  [unwired: 1 in, 1 out]
            n522 = local read "InjCmd"() -> (w645:T6)
            n523 = local read "InjAdaptMode"() -> (w642:u32)
            n524 = Number To Boolean Array(number=w642) -> (Boolean array=w641:bool[])
            n525 = Index Array(array=w645, index="_ChannelConfigurationList") -> (element=w644:T7)
            n526 = Index Array(array=w641, index="_ChannelConfigurationList") -> (element=w637:bool)
            n527 = property on="_Redraw Timing Plot" class="Bool (strict)"("Val(Sgnl)"=TRUE ("Value (Signaling)")) -> ()  [unwired: 2 in, 2 out]
            n528 = property on="_Redraw DI Command" class="Bool (strict)"("Val(Sgnl)"=TRUE ("Value (Signaling)")) -> ()  [unwired: 2 in, 2 out]
            n529 = local write "_InjCmd Element"(w644) -> ()
            n530 = Select(t=T30."Disabled and Grayed Out" ("Disabled"), s=w637, f=T30."Enabled" ("Disabled")) -> (s? t:f=w638:T30)
            n531 = local write "_InjAdaptMode"(w637) -> ()
            n532 = property on="_InjCmd Element" class="Clust (strict)"("DisabledEnum"=w638) -> ()  [unwired: 2 in, 2 out]
          }
          event Value Change {
            n533 = event-data() -> ()  [unwired: 1 in, 1 out]
            n534 = property on="_Redraw Injection List" class="Bool (strict)"("Val(Sgnl)"=TRUE ("Value (Signaling)")) -> ()  [unwired: 2 in, 2 out]
            n535 = property on="_Redraw Timing Plot" class="Bool (strict)"("Val(Sgnl)"=TRUE ("Value (Signaling)")) -> ()  [unwired: 2 in, 2 out]
            n536 = property on="_Redraw DI Command" class="Bool (strict)"("Val(Sgnl)"=TRUE ("Value (Signaling)")) -> ()  [unwired: 2 in, 2 out]
            n537 = local read "_ChannelConfigurationList"() -> (w652:i32)
            n538 = local read "InjCmd"() -> (w653:T6)
            n539 = call "Resize DI Command Array.vi"("Command in"="_InjCmd Element") -> ("Command out"=w647:T7)
            n540 = Replace Array Subset(array=w653, new element=w647, index=w652) -> (w646:T6)
            n541 = local write "InjCmd"(w646) -> ()
          }
          event "_InjAdaptMode": Value Change {
            n542 = event-data() -> ("NewVal"=w654:bool)  [unwired: 1 in]
            n543 = local read "_ChannelConfigurationList"() -> (w659:i32)
            n544 = local read "InjAdaptMode"() -> (w660:u32)
            n545 = Number To Boolean Array(number=w660) -> (Boolean array=w661:bool[])
            n546 = Replace Array Subset(array=w661, new element=w654, index=w659) -> (w662:bool[])
            n547 = case shown="True" w654 {
              frame False {
                n548 = property on="_Redraw DI Command" class="Bool (strict)"("Val(Sgnl)"=TRUE ("Value (Signaling)")) -> ()  [unwired: 2 in, 2 out]
              }
              frame True {
              }
            }
            n549 = Boolean Array To Number(Boolean array=w662) -> (number=w658:u32)
            n550 = property on="InjAdaptMode" class="DigNum (strict)"("Val(Sgnl)"=w658) -> ()  [unwired: 2 in, 2 out]
            n551 = Select(t=T30."Disabled and Grayed Out" ("Disabled"), s=w654, f=T30."Enabled" ("Disabled")) -> (s? t:f=w655:T30)
            n552 = property on="_InjCmd Element" class="Clust (strict)"("DisabledEnum"=w655) -> ()  [unwired: 2 in, 2 out]
          }
          event "_DI_CopyToAllChannelConf": Value Change {
            # "Copy selected cmd channel to active cmd channels; coerce all non-active channels to OFF command state"
            n553 = event-data() -> ()  [unwired: 1 in, 1 out]
            n554 = local read "_DI Bank_Configuration"() -> (w671:T3)
            n555 = local write "_DI_CopyToAllChannelConf"(FALSE ("_Copy To All")) -> ()
            n556 = property on="_Redraw Injection List" class="Bool (strict)"("Val(Sgnl)"=TRUE ("Value (Signaling)")) -> ()  [unwired: 2 in, 2 out]
            n557 = Unbundle By Name(w671) -> ("Configuration"=w672:T4)
            n558 = local read "_ChannelConfigurationList"() -> (w666:i32)
            n559 = case shown="\"Piezo Unipolar 2\"" w672 {
              tunnel: [bool[] [TRUE, TRUE, TRUE, TRUE, FALSE, FALSE, FALSE, FALSE] bool[] [TRUE, TRUE, TRUE, TRUE, TRUE, TRUE, TRUE, FALSE] bool[] [TRUE, TRUE, TRUE, TRUE, TRUE, TRUE, TRUE, TRUE] bool[] [FALSE, TRUE, FALSE, TRUE, FALSE, FALSE, FALSE, FALSE] bool[] [FALSE, TRUE, TRUE, TRUE, FALSE, FALSE, FALSE, FALSE] bool[] [FALSE, TRUE, FALSE, TRUE, FALSE, FALSE, FALSE, FALSE] bool[] [FALSE, TRUE, TRUE, TRUE, FALSE, FALSE, FALSE, FALSE] bool[] [TRUE, TRUE, TRUE, TRUE, FALSE, FALSE, FALSE, FALSE] bool[] [FALSE, TRUE, FALSE, TRUE, FALSE, FALSE, FALSE, FALSE] bool[] [FALSE, TRUE, TRUE, TRUE, FALSE, FALSE, FALSE, FALSE]] -> w668
              frame "Solenoid Unipolar 4", Default {
              }
              frame "Solenoid Unipolar 7 (Muxed)" {
              }
              frame "Solenoid Unipolar 8 (Muxed)" {
              }
              frame "Solenoid Bipolar 2" {
              }
              frame "Solenoid Bipolar 3 (Muxed)" {
              }
              frame "Piezo Unipolar 2" {
              }
              frame "Piezo Unipolar 3 (Muxed)" {
              }
              frame "Piezo Unipolar 4 (Muxed)" {
              }
              frame "Piezo Bipolar 2" {
              }
              frame "Piezo Bipolar 3 (Muxed)" {
              }
            }
            n560 = local read "InjCmd"() -> (w667:T6)
            n561 = Index Array(array=w667, index=w666) -> (element=w669:T7)
            n562 = for {
              N: 8 -> [_]
              shift-right: [w674] -> w664
              shift-left: w667 -> [w678]
              tunnel: w669 -> [w676]
              tunnel: w668 -> [w675] mode=indexing
              i -> [w677]
              n563 = in-place {
                in-place-border: w676 -> [w681]
                in-place-border: w675 -> [w682]
                n564 = in-place-array #2(w678, w677) -> (w679:T7)
                n565 = case shown="False" w682 {
                  tunnel: w681 -> [_ w684]
                  tunnel: [w683 w684] -> w680
                  tunnel: w679 -> [w683 _]
                  frame False {
                  }
                  frame True {
                  }
                }
                n566 = in-place-array #2(w680) -> (w674:T6)  [unwired: 1 out]
              }
            }
            n567 = local write "InjCmd"(w664) -> ()
          }
          event "_Plot Selector (T=TMP, F=EPT)": Value Change {
            n568 = event-data() -> ()  [unwired: 1 in, 6 out]
            n569 = property on="_Redraw Timing Plot" class="Bool (strict)"("Val(Sgnl)"=TRUE ("Value (Signaling)")) -> ()  [unwired: 2 in, 2 out]
          }
          event "_Redraw Timing Plot": Value Change {
            n570 = event-data() -> ()  [unwired: 1 in, 6 out]
            n571 = local write "_Redraw Timing Plot"(FALSE ("_Redraw Timing Plot")) -> ()
            n572 = local read "SimRotations"() -> (w700:u8)
            n573 = local read "SimSpeed"() -> (w701:sgl)
            n574 = local read "_ChannelConfigurationList"() -> (w711:i32)
            n575 = local read "SimBatt"() -> (w702:sgl)
            n576 = local read "InjCmd"() -> (w712:T6)
            n577 = Bundle By Name(cluster=T34 {"Battery [V]"=13.7, "Engine Speed [RPM]"=1000.0, "Rotations"=2, "Injector Configuration"={"Resistance [Ohm]"=1.0, "Inductance [Henery]"=0.001, "Capacitance [Farad]"=5e-06}, "Description"=""} ("System Configuration"), "Battery [V]"=w702, "Engine Speed [RPM]"=w701, "Rotations"=w700) -> (w696:T34)
            n578 = Index Array(array=w712, index=w711) -> (element=w697:T7)
            n579 = Select(t="Time after Trigger [sec]" ("X Scale.Name Label.Text 2"), s="_Plot Selector (T=TMP, F=EPT)", f="Timing [DBTDC]" ("X Scale.Name Label.Text 2")) -> (s? t:f=w707:string)
            n580 = Select(t="Trigger" ("Plot.Plot Name 2"), s="_Plot Selector (T=TMP, F=EPT)", f="Window" ("Plot.Plot Name 2")) -> (s? t:f=w710:string)
            n581 = case shown="False" "_Plot Selector (T=TMP, F=EPT)" {
              tunnel: [w715 w718] -> w698
              tunnel: w697 -> [w716 w717]
              tunnel: w696 -> [w714 _]
              frame False {
                n582 = call "Injection Command Plot - EPT.vi"("System"=w714, "Injection Command"=w716) -> ("Plot"=w715:cluster{"Array":sgl[], "Array":sgl[]}[])  [unwired: 9 in]
              }
              frame True {
                n583 = call "Injection Command Plot - TMP.vi"("Injection Command"=w717) -> ("Plot"=w718:cluster{"Array":sgl[], "Array":sgl[]}[])  [unwired: 10 in]
              }
            }
            "_Timing Plot" <- w698
            n584 = property on="_Timing Plot" class="XYGraph (strict)"("XScale.NameLbl.Text"=w707, "Active Plot"=u32 0, "Plot.Plot Name"=w710) -> ()  [unwired: 2 in, 2 out]
          }
          event "_Redraw DI Command": Value Change {
            n585 = event-data() -> ()  [unwired: 1 in, 6 out]
            n586 = local write "_Redraw DI Command"(FALSE ("_Redraw DI Command")) -> ()
            n587 = control-ref of="_InjCmd Element"() -> (w719:refnum<vi>)
            n588 = call "Disable DI Command.vi"("Phase Ref"=w719) -> ()  [unwired: 11 in]
          }
          event "_Redraw Injection List": Value Change {
            n589 = event-data() -> ()  [unwired: 1 in, 1 out]
            n590 = local read "_DI Bank_Configuration"() -> (w726:T3)
            n591 = local read "InjCmd"() -> (w723:T6)
            n592 = local read "InjAdaptMode"() -> (w724:u32)
            n593 = local read "_Bank A?"() -> (w721:bool)
            n594 = control-ref of="_ChannelConfigurationList"() -> (w725:refnum<vi>)
            n595 = local write "_Redraw Injection List"(FALSE ("_Redraw Injection List")) -> ()
            n596 = call "Injection Configuration Listbox Setup.vi"("Bank A? (T)"=w721, "Inj Adapt Mode"=w724, "Command Cluster Array"=w723, "DI Bank Configuration"=w726, "Injection Configurations"=w725) -> ("Command Cluster Array"=w722:T7[])  [unwired: 6 in]
            n597 = property on="InjCmd" class="Arr (strict)"("Val(Sgnl)"=w722) -> ()  [unwired: 2 in, 2 out]
          }
          event "_DI-B Fault Clear": Value Change {
            n598 = event-data() -> ("NewVal"=w728:T27)  [unwired: 1 in]
            n599 = Cluster To Array(cluster=w728) -> (array=w730:bool[])
            n600 = Boolean Array To Number(Boolean array=w730) -> (number=w729:u8)
            n601 = property on="FaultClear" class="DigNum (strict)"("Val(Sgnl)"=w729) -> ()  [unwired: 2 in, 2 out]
          }
          event "PumpPhase Array": Value Change {
            n602 = event-data() -> ()  [unwired: 1 in, 6 out]
            n603 = local read "PumpPhase Array"() -> (w733:i32)
            n604 = local read "PumpPhase"() -> (w732:T12)
            n605 = property on="_Redraw Pump Phase" class="Bool (strict)"("Val(Sgnl)"=TRUE ("Value (Signaling)")) -> ()  [unwired: 2 in, 2 out]
            n606 = Index Array(array=w732, index=w733) -> (element=w734:T13)
            n607 = local write "_Pump Phase"(w734) -> ()
          }
          event "_Insert Pump Phase": Value Change {
            n608 = event-data() -> ()  [unwired: 1 in, 6 out]
            n609 = local read "PumpPhase Array"() -> (w738:i32)
            n610 = local read "PumpPhase"() -> (w739:T12)
            n611 = local write "_Insert Pump Phase"(FALSE ("_Insert Pump Phase 2")) -> ()
            n612 = Index Array(array=w739, index=w738) -> (element=w737:T13)
            n613 = property on="_Redraw Pump Phase" class="Bool (strict)"("Val(Sgnl)"=TRUE ("Value (Signaling)")) -> ()  [unwired: 2 in, 2 out]
            n614 = property on="_Redraw Pump Phase Plot" class="Bool (strict)"("Val(Sgnl)"=TRUE ("Value (Signaling)")) -> ()  [unwired: 2 in, 2 out]
            n615 = property on="_Redraw Pump Phase List" class="Bool (strict)"("Val(Sgnl)"=TRUE ("Value (Signaling)")) -> ()  [unwired: 2 in, 2 out]
            n616 = Insert Into Array(array=w739, index=w738, new element=w737) -> (w740:T12)
            n617 = local write "PumpPhase"(w740) -> ()
          }
          event "_Remove Pump Phase": Value Change {
            n618 = event-data() -> ()  [unwired: 1 in, 6 out]
            n619 = local read "PumpPhase Array"() -> (w747:i32)
            n620 = local read "PumpPhase"() -> (w745:T12)
            n621 = local write "_Remove Pump Phase"(FALSE ("_Remove Pump Phase")) -> ()
            n622 = property on="_Redraw Pump Phase" class="Bool (strict)"("Val(Sgnl)"=TRUE ("Value (Signaling)")) -> ()  [unwired: 2 in, 2 out]
            n623 = property on="_Redraw Pump Phase Plot" class="Bool (strict)"("Val(Sgnl)"=TRUE ("Value (Signaling)")) -> ()  [unwired: 2 in, 2 out]
            n624 = property on="_Redraw Pump Phase List" class="Bool (strict)"("Val(Sgnl)"=TRUE ("Value (Signaling)")) -> ()  [unwired: 2 in, 2 out]
            n625 = Delete From Array(array=w745, index=w747) -> (array with subset deleted=w746:T12)  [unwired: 1 in, 1 out]
            n626 = Index Array(array=w746, index=w747) -> (element=w748:T13)
            n627 = local write "_Pump Phase"(w748) -> ()
            n628 = local write "PumpPhase"(w746) -> ()
          }
          event Value Change {
            n629 = event-data() -> ()  [unwired: 1 in, 6 out]
            n630 = local read "PumpPhase Array"() -> (w756:i32)
            n631 = local read "PumpPhase"() -> (w755:T12)
            n632 = Replace Array Subset(array=w755, new element="_Pump Phase", index=w756) -> (w751:T12)
            n633 = property on="_Redraw Pump Phase List" class="Bool (strict)"("Val(Sgnl)"=TRUE ("Value (Signaling)")) -> ()  [unwired: 2 in, 2 out]
            n634 = property on="_Redraw Pump Phase" class="Bool (strict)"("Val(Sgnl)"=TRUE ("Value (Signaling)")) -> ()  [unwired: 2 in, 2 out]
            n635 = property on="_Redraw Pump Phase Plot" class="Bool (strict)"("Val(Sgnl)"=TRUE ("Value (Signaling)")) -> ()  [unwired: 2 in, 2 out]
            n636 = local write "PumpPhase"(w751) -> ()
          }
          event "SimPumpDuration": Value Change {
            n637 = event-data() -> ()  [unwired: 1 in, 6 out]
            n638 = property on="_Redraw Pump Phase Plot" class="Bool (strict)"("Val(Sgnl)"=TRUE ("Value (Signaling)")) -> ()  [unwired: 2 in, 2 out]
          }
          event "_Redraw Pump Phase Plot": Value Change {
            n639 = event-data() -> ()  [unwired: 1 in, 6 out]
            n640 = local read "_DI Bank_Configuration"() -> (w791:T3)
            n641 = local read "PumpCapacitance"() -> (w766:sgl)
            n642 = local read "PumpInductance"() -> (w767:sgl)
            n643 = local read "PumpResistance"() -> (w768:sgl)
            n644 = Bundle By Name(cluster=T33 {"Resistance [Ohm]"=1.0, "Inductance [Henery]"=0.001, "Capacitance [Farad]"=5e-06} ("Injector Configuration"), "Resistance [Ohm]"=w768, "Inductance [Henery]"=w767, "Capacitance [Farad]"=w766) -> (w764:T33)
            n645 = Unbundle By Name(w791) -> ("Boost Voltage [V]"=w790:sgl, "Pump Zener Enable"=w759:bool, "Pump Zener Voltage [V]"=w760:sgl)
            n646 = local read "SimBatt"() -> (w765:sgl)
            n647 = local read "_Ref Pump Profiles"() -> (w782:cluster{"Array":dbl[], "Array":dbl[]}[])
            n648 = Bundle By Name(cluster=T34 {"Battery [V]"=13.7, "Engine Speed [RPM]"=0.0, "Rotations"=0, "Injector Configuration"={"Resistance [Ohm]"=1.0, "Inductance [Henery]"=0.001, "Capacitance [Farad]"=5e-06}, "Description"=""} ("System"), "Battery [V]"=w765, "Injector Configuration"=w764) -> (w789:T34)
            n649 = Bundle By Name(cluster=T32 {"Configuration"=enum."Solenoid Unipolar 4", "Boost Voltage [V]"=0.0, "Zener Enable"=FALSE, "Zener Voltage [V]"=0.0} ("Configuration"), "Configuration"=DI_-_Bank_Configuration."Solenoid Unipolar 4", "Boost Voltage [V]"=w790, "Zener Enable"=w759, "Zener Voltage [V]"=w760) -> (w788:T32)
            n650 = local read "PumpPhase"() -> (w787:T12)
            n651 = Index Array(array=w782) -> (element #1=w781:cluster{"Array":dbl[], "Array":dbl[]}, element #2=w779:cluster{"Array":dbl[], "Array":dbl[]})  [unwired: 2 in]
            n652 = Unbundle(w781) -> ("Array"=w778:dbl[], "Array"=w780:dbl[])
            n653 = Unbundle(w779) -> ("Array"=w777:dbl[], "Array"=w771:dbl[])
            n654 = call <vilib>:"Phase Plot.vi"("Phase Arrays"=w787, "System"=w789, "Configuration"=w788, "Duration (1m) [s]"="SimPumpDuration") -> ("Plot"=w784:cluster{"Array":sgl[], "Array":sgl[]}[])  [unwired: 14 in, 1 out]
            n655 = for {
              tunnel: w778 -> [w798] mode=indexing
              tunnel: [w798] -> w786 mode=indexing if=w799
              tunnel: [w800] -> w785 mode=indexing if=w799
              tunnel: w780 -> [w800] mode=indexing
              n656 = Greater Or Equal To 0?(x=w798) -> (x >= 0?=w799:bool)
            }
            n657 = for {
              tunnel: w777 -> [w795] mode=indexing
              tunnel: [w795] -> w776 mode=indexing if=w796
              tunnel: [w797] -> w775 mode=indexing if=w796
              tunnel: w771 -> [w797] mode=indexing
              n658 = Greater Or Equal To 0?(x=w795) -> (x >= 0?=w796:bool)
            }
            n659 = Empty Array?(array=w780) -> (empty?=w772:bool)
            n660 = Empty Array?(array=w771) -> (empty?=w770:bool)
            n661 = local write "_Redraw Pump Phase Plot"(FALSE ("_Redraw Pump Phase Plot")) -> ()
            n662 = Compound Arithmetic op=OR(invert w772, invert w770) -> (w773:bool)
            n663 = Bundle(w786, w785) -> (w783:cluster{dbl[], dbl[]})  [unwired: 1 in]
            n664 = Bundle(w776, w775) -> (w774:cluster{dbl[], dbl[]})  [unwired: 1 in]
            n665 = case shown="True" w773 {
              tunnel: w784 -> [w802 w809]
              tunnel: [w802 w808] -> w763
              tunnel: w783 -> [_ w804]
              tunnel: w774 -> [_ w803]
              frame False {
                n666 = property on="_Pump Phase Plot" class="XYGraph (strict)"("LegNumRows"=u32 6 ("Legend:Number of Rows")) -> ()  [unwired: 2 in, 2 out]
              }
              frame True {
                n667 = Build Array (concatenate)(w809, w804, w803) -> (w808:cluster{"Array":dbl[], "Array":dbl[]}[])
                n668 = property on="_Pump Phase Plot" class="XYGraph (strict)"("Active Plot"=u32 6, "Plot.Plot Name"="Ref [A]", "LegNumRows"=u32 7 ("Legend:Number of Rows")) -> ()  [unwired: 2 in, 2 out]
              }
            }
            "_Pump Phase Plot" <- w763
          }
          event "_Redraw Pump Phase List": Value Change {
            n669 = event-data() -> ()  [unwired: 1 in, 6 out]
            n670 = local read "PumpPhase"() -> (w810:T12)
            n671 = local read "PumpPhase Array"() -> (w814:i32)
            n672 = control-ref of="PumpPhase Array"() -> (w817:refnum<vi>)
            n673 = Build Array(w810) -> (w816:T13[][])
            n674 = property on="PumpPhase" class="Arr (strict)"("Val(Sgnl)"=w810) -> ()  [unwired: 2 in, 2 out]
            n675 = call <vilib>:"Phase Listbox.vi"("Phase Arrays"=w816, "Phase Array"=w817) -> ()  [unwired: 9 in, 1 out]
            n676 = In Range and Coerce(upper limit=15, x=w814, lower limit=0) -> (coerced(x)=w815:i32, In Range?=w811:bool)
            n677 = case shown="False" w811 {
              tunnel: w815 -> [w819 _]
              frame False {
                n678 = property on="PumpPhase Array" class="LstBox (strict)"("Val(Sgnl)"=w819) -> ()  [unwired: 2 in, 2 out]
              }
              frame True {
              }
            }
            n679 = local write "_Redraw Pump Phase List"(FALSE ("_Redraw Pump Phase List")) -> ()
          }
          event "_Redraw Pump Phase": Value Change {
            n680 = event-data() -> ()  [unwired: 1 in, 1 out]
            n681 = local read "_DI Bank_Configuration"() -> (w828:T3)
            n682 = local write "_Redraw Pump Phase"(FALSE ("Redraw Phase")) -> ()
            n683 = Unbundle By Name(w828) -> ("Configuration"=w827:T4, "Boost Voltage [V]"=w826:sgl, "DI Zener Enable"=w825:bool, "DI Zener Voltage [V]"=w824:sgl)
            n684 = Bundle By Name(cluster=T32 {"Configuration"=enum."Solenoid Unipolar 4", "Boost Voltage [V]"=0.0, "Zener Enable"=FALSE, "Zener Voltage [V]"=0.0} ("Configuration"), "Configuration"=w827, "Boost Voltage [V]"=w826, "Zener Enable"=w825, "Zener Voltage [V]"=w824) -> (w822:T32)
            n685 = control-ref of="_Pump Phase"() -> (w821:refnum<vi>)
            n686 = call <vilib>:"Disable Phase Array.vi"("Pump (F)"=TRUE, "Configuration"=w822, "Phase Ref"=w821) -> ()  [unwired: 9 in]
          }
          event "_Ref Pump Current Profile FilePath": Value Change {
            n687 = event-data() -> ()  [unwired: 1 in, 6 out]
            n688 = Read from Text File(file (use dialog)="_Ref Pump Current Profile FilePath") -> (text=w850:string)  [unwired: 3 in, 3 out]
            n689 = Spreadsheet String To Array(delimiter (Tab)=",", format string="%g", spreadsheet string=w850) -> (array=w853:dbl[][])  [unwired: 1 in]
            n690 = Transpose 2D Array(2D array=w853) -> (transposed array=w849:dbl[][])
            n691 = Index Array(array=w849) -> (element #1=w844:dbl[], element #2=w846:dbl[], element #3=w837:dbl[])  [unwired: 6 in]
            n692 = Compound Arithmetic op=MULTIPLY("RefPumpTimeAxisMultiplier", w844) -> (w845:dbl[])
            n693 = Compound Arithmetic op=MULTIPLY("RefPumpCurrentMultiplier", w846) -> (w839:dbl[])
            n694 = Compound Arithmetic op=MULTIPLY("RefPumpVoltageMultiplier", w837) -> (w838:dbl[])
            n695 = Compound Arithmetic op=ADD(w845, "RefPumpTimeAxisOffset") -> (w833:dbl[])
            n696 = Compound Arithmetic op=ADD(w839, "RefPumpCurrentOffset") -> (w847:dbl[])
            n697 = Compound Arithmetic op=ADD(w838, "RefPumpVoltageOffset") -> (w834:dbl[])
            n698 = property on="_Redraw Pump Phase Plot" class="Bool (strict)"("Val(Sgnl)"=TRUE ("Value (Signaling)")) -> ()  [unwired: 2 in, 2 out]
            n699 = Bundle(w833, w847) -> (w832:cluster{dbl[], dbl[]})  [unwired: 1 in]
            n700 = Bundle(w833, w834) -> (w830:cluster{dbl[], dbl[]})  [unwired: 1 in]
            n701 = Build Array(w832, w830) -> (→"_Ref Pump Profiles":cluster{dbl[], dbl[]}[])
          }
          event "_Pump A Plot Selector (T=TMP, F=EPT)": Value Change {
            n702 = event-data() -> ()  [unwired: 1 in, 6 out]
            n703 = property on="_Redraw Pump Timing Plot" class="Bool (strict)"("Val(Sgnl)"=TRUE ("Value (Signaling)")) -> ()  [unwired: 2 in, 2 out]
          }
          event Value Change {
            n704 = event-data() -> ()  [unwired: 1 in, 6 out]
            n705 = property on="_Redraw Pump Timing Plot" class="Bool (strict)"("Val(Sgnl)"=TRUE ("Value (Signaling)")) -> ()  [unwired: 2 in, 2 out]
            n706 = property on="_Redraw Pump Command" class="Bool (strict)"("Val(Sgnl)"=TRUE ("Value (Signaling)")) -> ()  [unwired: 2 in, 2 out]
            n707 = call "Resize DI Command Array.vi"("Command in"="PumpCmd") -> ("Command out"=w856:T7)
            n708 = local write "PumpCmd"(w856) -> ()
          }
          event "_Redraw Pump Timing Plot": Value Change {
            n709 = event-data() -> ()  [unwired: 1 in, 6 out]
            n710 = local read "SimRotations"() -> (w864:u8)
            n711 = local read "SimSpeed"() -> (w865:sgl)
            n712 = local read "SimBatt"() -> (w866:sgl)
            n713 = Bundle By Name(cluster=T34 {"Battery [V]"=13.7, "Engine Speed [RPM]"=1000.0, "Rotations"=2, "Injector Configuration"={"Resistance [Ohm]"=1.0, "Inductance [Henery]"=0.001, "Capacitance [Farad]"=5e-06}, "Description"=""} ("System Configuration"), "Battery [V]"=w866, "Engine Speed [RPM]"=w865, "Rotations"=w864) -> (w861:T34)
            n714 = local read "PumpCmd"() -> (w862:T26)
            n715 = case shown="False" "_Pump A Plot Selector (T=TMP, F=EPT)" {
              tunnel: [w877 w880] -> w863
              tunnel: w862 -> [w878 w879]
              tunnel: w861 -> [w876 _]
              frame False {
                n716 = call "Injection Command Plot - EPT.vi"("System"=w876, "Injection Command"=w878) -> ("Plot"=w877:cluster{"Array":sgl[], "Array":sgl[]}[])  [unwired: 9 in]
              }
              frame True {
                n717 = call "Injection Command Plot - TMP.vi"("Injection Command"=w879) -> ("Plot"=w880:cluster{"Array":sgl[], "Array":sgl[]}[])  [unwired: 10 in]
              }
            }
            "_Pump Timing Plot" <- w863
            n718 = Select(t="Time after Trigger [sec]" ("X Scale.Name Label.Text 2"), s="_Pump A Plot Selector (T=TMP, F=EPT)", f="Timing [DBTDC]" ("X Scale.Name Label.Text 2")) -> (s? t:f=w870:string)
            n719 = Select(t="Trigger" ("Plot.Plot Name 2"), s="_Pump A Plot Selector (T=TMP, F=EPT)", f="Window" ("Plot.Plot Name 2")) -> (s? t:f=w873:string)
            n720 = property on="_Pump Timing Plot" class="XYGraph (strict)"("XScale.NameLbl.Text"=w870, "Active Plot"=u32 0, "Plot.Plot Name"=w873) -> ()  [unwired: 2 in, 2 out]
            n721 = local write "_Redraw Pump Timing Plot"(FALSE ("_Redraw Pump Timing Plot")) -> ()
          }
          event "_Redraw Pump Command": Value Change {
            n722 = event-data() -> ()  [unwired: 1 in, 6 out]
            n723 = local write "_Redraw Pump Command"(FALSE ("_Redraw Pump Command")) -> ()
            n724 = control-ref of="PumpCmd"() -> (w881:refnum<vi>)
            n725 = call "Disable DI Command.vi"("Pump Channel? (F)"=TRUE, "Phase Ref"=w881) -> ()  [unwired: 10 in]
          }
          event "PumpAdaptMode": Value Change {
            n726 = event-data() -> ("NewVal"=w884:bool)  [unwired: 1 in]
            n727 = case shown="False" w884 {
              frame False {
                n728 = property on="_Redraw Pump Command" class="Bool (strict)"("Val(Sgnl)"=TRUE ("Value (Signaling)")) -> ()  [unwired: 2 in, 2 out]
              }
              frame True {
              }
            }
            n729 = Select(t=T30."Disabled and Grayed Out" ("Disabled"), s=w884, f=T30."Enabled" ("Disabled")) -> (s? t:f=w885:T30)
            n730 = property on="PumpCmd" class="Clust (strict)"("DisabledEnum"=w885) -> ()  [unwired: 2 in, 2 out]
          }
          event "_Phase Plot": Plot Attribute Change {
            n731 = event-data() -> ()  [unwired: 1 in, 8 out]
            n732 = property on="_Phase Plot" class="XYGraph (strict)"() -> ("LegNumRows"=w892:u32)  [unwired: 2 in, 2 out]
            n733 = for {
              N: w892 -> [_]
              tunnel: [w895] -> w890 mode=indexing
              tunnel: [w894] -> w891 mode=indexing
              tunnel: [w893] -> w889 mode=indexing
              i -> [w896]
              n734 = property on="_Phase Plot" class="XYGraph (strict)"("Active Plot"=w896) -> ("Plot.Plot Color"=w895:u32, "Plot.Line Width"=w894:u8, "Plot.Line Style"=w893:u8)  [unwired: 2 in, 2 out]
            }
            n735 = property on="PumpPhasePlotColors" class="Arr (strict)"("Val(Sgnl)"=w890) -> ()  [unwired: 2 in, 2 out]
            n736 = property on="InjPhasePlotLineWidths" class="Arr (strict)"("Val(Sgnl)"=w891) -> ()  [unwired: 2 in, 2 out]
            n737 = property on="InjPhasePlotLineTypes" class="Arr (strict)"("Val(Sgnl)"=w889) -> ()  [unwired: 2 in, 2 out]
          }
          event "_Pump Phase Plot": Plot Attribute Change {
            n738 = event-data() -> ()  [unwired: 1 in, 8 out]
            n739 = property on="_Pump Phase Plot" class="XYGraph (strict)"() -> ("LegNumRows"=w900:u32)  [unwired: 2 in, 2 out]
            n740 = for {
              N: w900 -> [_]
              tunnel: [w903] -> w899 mode=indexing
              tunnel: [w902] -> w898 mode=indexing
              tunnel: [w901] -> w897 mode=indexing
              i -> [w904]
              n741 = property on="_Pump Phase Plot" class="XYGraph (strict)"("Active Plot"=w904) -> ("Plot.Plot Color"=w903:u32, "Plot.Line Width"=w902:u8, "Plot.Line Style"=w901:u8)  [unwired: 2 in, 2 out]
            }
            n742 = property on="PumpPhasePlotLineTypes" class="Arr (strict)"("Val(Sgnl)"=w897) -> ()  [unwired: 2 in, 2 out]
            n743 = property on="InjPhasePlotColors" class="Arr (strict)"("Val(Sgnl)"=w899) -> ()  [unwired: 2 in, 2 out]
            n744 = property on="PumpPhasePlotLineWidths" class="Arr (strict)"("Val(Sgnl)"=w898) -> ()  [unwired: 2 in, 2 out]
          }
          event "_Timing Plot": Plot Attribute Change {
            n745 = event-data() -> ()  [unwired: 1 in, 8 out]
            n746 = property on="_Timing Plot" class="XYGraph (strict)"() -> ("LegNumRows"=w908:u32)  [unwired: 2 in, 2 out]
            n747 = for {
              N: w908 -> [_]
              tunnel: [w911] -> w907 mode=indexing
              tunnel: [w910] -> w906 mode=indexing
              tunnel: [w909] -> w905 mode=indexing
              i -> [w912]
              n748 = property on="_Timing Plot" class="XYGraph (strict)"("ActXScl"=w912) -> ("Plot.Plot Color"=w911:u32, "Plot.Line Width"=w910:u8, "Plot.Line Style"=w909:u8)  [unwired: 2 in, 2 out]
            }
            n749 = property on="InjCmdPlotColors" class="Arr (strict)"("Val(Sgnl)"=w907) -> ()  [unwired: 2 in, 2 out]
            n750 = property on="InjCmdPlotLineWidths" class="Arr (strict)"("Val(Sgnl)"=w906) -> ()  [unwired: 2 in, 2 out]
            n751 = property on="InjCmdPlotLineTypes" class="Arr (strict)"("Val(Sgnl)"=w905) -> ()  [unwired: 2 in, 2 out]
          }
          event "_Pump Timing Plot": Plot Attribute Change {
            n752 = event-data() -> ()  [unwired: 1 in, 8 out]
            n753 = property on="_Pump Timing Plot" class="XYGraph (strict)"() -> ("LegNumRows"=w916:u32)  [unwired: 2 in, 2 out]
            n754 = for {
              N: w916 -> [_]
              tunnel: [w919] -> w915 mode=indexing
              tunnel: [w918] -> w914 mode=indexing
              tunnel: [w917] -> w913 mode=indexing
              i -> [w920]
              n755 = property on="_Pump Timing Plot" class="XYGraph (strict)"("ActXScl"=w920) -> ("Plot.Plot Color"=w919:u32, "Plot.Line Width"=w918:u8, "Plot.Line Style"=w917:u8)  [unwired: 2 in, 2 out]
            }
            n756 = property on="PumpCmdPlotColors" class="Arr (strict)"("Val(Sgnl)"=w915) -> ()  [unwired: 2 in, 2 out]
            n757 = property on="PumpCmdPlotLineWidths" class="Arr (strict)"("Val(Sgnl)"=w914) -> ()  [unwired: 2 in, 2 out]
            n758 = property on="PumpCmdPlotLineTypes" class="Arr (strict)"("Val(Sgnl)"=w913) -> ()  [unwired: 2 in, 2 out]
          }
          event "_Redraw Slider": Value Change {
            n759 = event-data() -> ()  [unwired: 1 in, 6 out]
            n760 = local write "_Redraw Slider"(FALSE ("_Redraw Slider")) -> ()
            n761 = local read "_DI Bank_Configuration"() -> (w922:T3)
            n762 = local read "_Bank A?"() -> (w921:bool)
            n763 = local read "State"() -> (w923:T19)
            n764 = call "DI Redraw Boost Slider.vi"("Bank A? (T)"=w921, "DCM System State"=w923, "DI Bank Configuration"=w922) -> ("Levels Slider"=w924:cluster{dbl, dbl, dbl, dbl})  [unwired: 8 in]
            n765 = local write "_BoostSlider"(w924) -> ()
          }
        }
      }
    }
  }
  n766 = First Call?() -> ()  [unwired: 1 out]
